vi "Trajectory Builder.vi"() -> ()   [LabVIEW 2025]
uses:
  Types/Limits.ctl
  Types/Overrides.ctl
  Types/Trajectory Data.ctl
  Types/Segment Type.ctl
  Types/Path Type.ctl
  Types/Drive Type.ctl
  Types/Angluar Limits.ctl
  Types/Command Editor Info.ctl
  Types/Single Cmd Info.ctl
  <vilib>/picture/picture.llb/imagedata.ctl
  <vilib>/Utility/miscctls.llb/LVPositionTypeDef.ctl
  Types/Full Command Info.ctl
  <vilib>/Utility/miscctls.llb/LVRowAndColumnTypeDef.ctl
  Types/Internal Path Stuff.ctl
  Types/Aquitaine File Data.ctl
  Types/Decision Tree.ctl
  Types/Sequencing Tree Node.ctl
  <vilib>/event_ctls.llb/lveventtype.ctl
  36995695-6583-4118-8a12-9ab3bbd2de6a.vi
  6a65ebb4-e776-4ba2-b94f-6ff829af6114.vi
  88e6daad-a1e9-44cd-90fd-d41817f6f65e.vi
  36995695-6583-4118-8a12-9ab3bbd2de6a.vi/4611cae3-c7be-41e2-9a5e-ea0ae78a7ced.vi
  6a65ebb4-e776-4ba2-b94f-6ff829af6114.vi/c0db33a9-eb6c-44d9-b982-8563e05d2734.vi
  6a65ebb4-e776-4ba2-b94f-6ff829af6114.vi/ae3535a8-0066-4e8d-a5de-b07ac05a7c65.vi
  6a65ebb4-e776-4ba2-b94f-6ff829af6114.vi/dda8e586-731b-4197-ad83-6a4d05585a0a.vi
  36995695-6583-4118-8a12-9ab3bbd2de6a.vi/4611cae3-c7be-41e2-9a5e-ea0ae78a7ced.vi/19e2e4cb-e3bb-4239-bd5f-680916605f5d.vi
  36995695-6583-4118-8a12-9ab3bbd2de6a.vi/4611cae3-c7be-41e2-9a5e-ea0ae78a7ced.vi/f72612c1-738a-48a1-9fcf-3db66cb27fb3.vi
  36995695-6583-4118-8a12-9ab3bbd2de6a.vi/4611cae3-c7be-41e2-9a5e-ea0ae78a7ced.vi/45406051-8994-464b-8b47-ac12a8cbadfa.vi
  36995695-6583-4118-8a12-9ab3bbd2de6a.vi/4611cae3-c7be-41e2-9a5e-ea0ae78a7ced.vi/dd886480-778c-48b1-8e4a-d6890e1a60dd.vi
  36995695-6583-4118-8a12-9ab3bbd2de6a.vi/4611cae3-c7be-41e2-9a5e-ea0ae78a7ced.vi/2e6e140f-e361-4312-a09e-e37273ac7fd1.vi
  36995695-6583-4118-8a12-9ab3bbd2de6a.vi/4611cae3-c7be-41e2-9a5e-ea0ae78a7ced.vi/3589548e-4c68-4568-af05-72ab28470577.vi
  36995695-6583-4118-8a12-9ab3bbd2de6a.vi/4611cae3-c7be-41e2-9a5e-ea0ae78a7ced.vi/cf64d4f5-91bd-4749-9577-68c6ded0155b.vi
  36995695-6583-4118-8a12-9ab3bbd2de6a.vi/4611cae3-c7be-41e2-9a5e-ea0ae78a7ced.vi/6f6fefe9-f25b-4595-b26f-75715299a794.vi
  36995695-6583-4118-8a12-9ab3bbd2de6a.vi/4611cae3-c7be-41e2-9a5e-ea0ae78a7ced.vi/c74ffb76-1048-4639-9a95-b6de96ba7014.vi
  Global Settings.vi
  <vilib>/Utility/cursorutil.llb/Set Cursor (Icon Pict).vi
  <vilib>/Analysis/1siggen.llb/Ramp Pattern by Delta.vi
  <vilib>/Comparison/Less/Less Functor/Less Functor.lvclass
  <vilib>/Analysis/NI_AALBase.lvlib
panel:
  in  "Open Aquitaine Editor":bool
  in  "Add Paths":bool
  in  "Aquitaine Add Selector":u16(ring) items=["Karthik.aqt"]
  in  "Delete AQT":bool
  in  "Push BORAQT":bool
  in  "Push AQT":bool
  in  "New AQT":bool
  in  "Zero Translational\n Velocity":bool
  in  "Delete":bool
  out "Picture":picture
  in  "New Page Selector":T1(radio)
  in  "Push":bool
  out "?":bool
  out "RS":bool=TRUE
  in  "Cache":T5
  in  "Zero Velocity":bool
  in  "Reverse Path":bool
  in  "Robot Backwards":bool
  out "Duration (s)":dbl format="%#.4g"
  out "Distance (ft)":dbl format="%#.1g"
  in  "Instructions":string="Directions:\nUse mouse to ...\n    move robot position (rectangle with arrow)\n    rotate robot (red arrow)\n    move waypoints (numbered circles)\nClick in open space to add a waypoint\nShift click to delete a waypoint\nHover over a waypoint and use arrow keys to nudge\n\nTime slider and Play button will run robot along path to test for collisions.\n\nNew creates a new path at default location\n\nAppend creates a path using current path's position and heading.\n\nTo add a command, move robot using Time slider and double click the Command in Palette.\n\nYou can modify command timing in the graph or Command Sequencer tree.\n\nEnable/disable a command by clicking on the enable column item.\n\nDelete a command by shift-clicking in the enable column.\n\nTo configure command parameters, Select the command name in the tree, Open Panel, enter parameters, and Inhale the parameters.\n\nYou may sometimes want to type values into WayPoints directly.\n\nOverrides allow you to set accel and V limits for any turn."
  out "Command Palette":picture
  in  "Directory":bool
  in  "Tab Control":T1(tab)
  in  "Vertical Reflection":bool
  in  "Angular Limits":T6={"Velocity (deg/s)"=6.0, "Accel (deg/s^2)"=360.0, "Jerk (deg/s^3)"=1000.0} {"Jerk (deg/s^3)" min=0.01 step=1.0; "Accel (deg/s^2)" min=0.01; "Velocity (deg/s)" min=0.01}
  in  "Path Type":T7
  in  "Overrides":T8 {"Angle Override" step=5.0; "Velocity Override" step=5.0; "Angular Override" step=5.0}
  in  "Horizontal Reflection":bool
  in  "Sample Period (s)":dbl=0.02 min=0.001 max=1.0 format="%#_6f"
  in  "Limits":T9={"Velocity (fps)"=6.0, "Accel (fps^2)"=15.0, "Jerk (fps^3)"=150.0, "StoopidFast (fps)"=6.0} {"StoopidFast (fps)" min=0.01; "Jerk (fps^3)" min=0.01 step=1.0; "Accel (fps^2)" min=0.01; "Velocity (fps)" min=0.01}
  in  "Conditions":T10 {"vFinal (fps)" min=0.0; "vInitial (fps)" min=0.0}
  in  "Drive Type":T11=enum."Holonomic"
  in  "Turn Rate (Bezier)":dbl=5.0 format="%#_13g"
  in  "Origin Reflection":bool
  in  "Current Limit":dbl=50.0 min=0.01
  in  "WayPoints":cluster{"x":dbl, "y":dbl, "th":dbl}[](array[cluster])
  in  "Turn Angle Limit (deg)":dbl=90.0
  in  "Allow Angles > 90":bool=TRUE
  in  "Stoopid Overlap %":dbl min=0.0
  in  "Unjank":bool
  in  "Turn Deceleration":bool=TRUE
  in  "Turn Acceleration":bool=TRUE
  out "Trajectory Data":T12
  in  "Open Command":bool
  in  "Inhale":bool
  in  "Command Sequence":string(tree)
  in  "Projects":u16(ring) items=["Robot Code Template.lvproj"]
  in  "Refresh":bool
  in  "Snap to foot":bool
  in  "Angle Limiter":enum16{"90", "45", "15", "1"}(ring)=enum."15"
  in  "Snap robot to baseline":bool
  in  "Background":u16(ring) items=["Rebuilt", "Reefscape"]
  in  "Robot Color":u32(colorbox)=14421504
  out "Field Size (ft)":cluster{"width":dbl, "height":dbl}={"width"=26.4166, "height"=57.5729} {"width" format="%#.2g"; "height" format="%#.2g"}
  in  "Robot Size (in)":cluster{"width":dbl, "height":dbl}={"width"=24.0, "height"=30.0}
  in  "Hide Path":bool
  in  "Draw?":bool
  in  "Draw Delete":bool
  in  "Draw Menu":i32[](listbox)
  in  "Time (s)":dbl(slide) scale=0.0..1.6400000000000001 scale format="%#.1g"
  in  "Play":bool
  out "fps":dbl[](graph)
  in  "Append":bool
  in  "Filename":string
  in  "Save":bool
  in  "New":bool
  in  "File Manager":enum32{"Bordeaux Files", "Aquitaine Files"}(tab)
  in  "Open":i32[](listbox)
  in  "Tree":string[](tree)
  # "Command Palette"
  # "StupidFast makes each linear segment into a\nvelocity ramp to max speed (for clothoid paths only)"
  # "Nicotine"
  # "A"
  # "V"
  # "O"
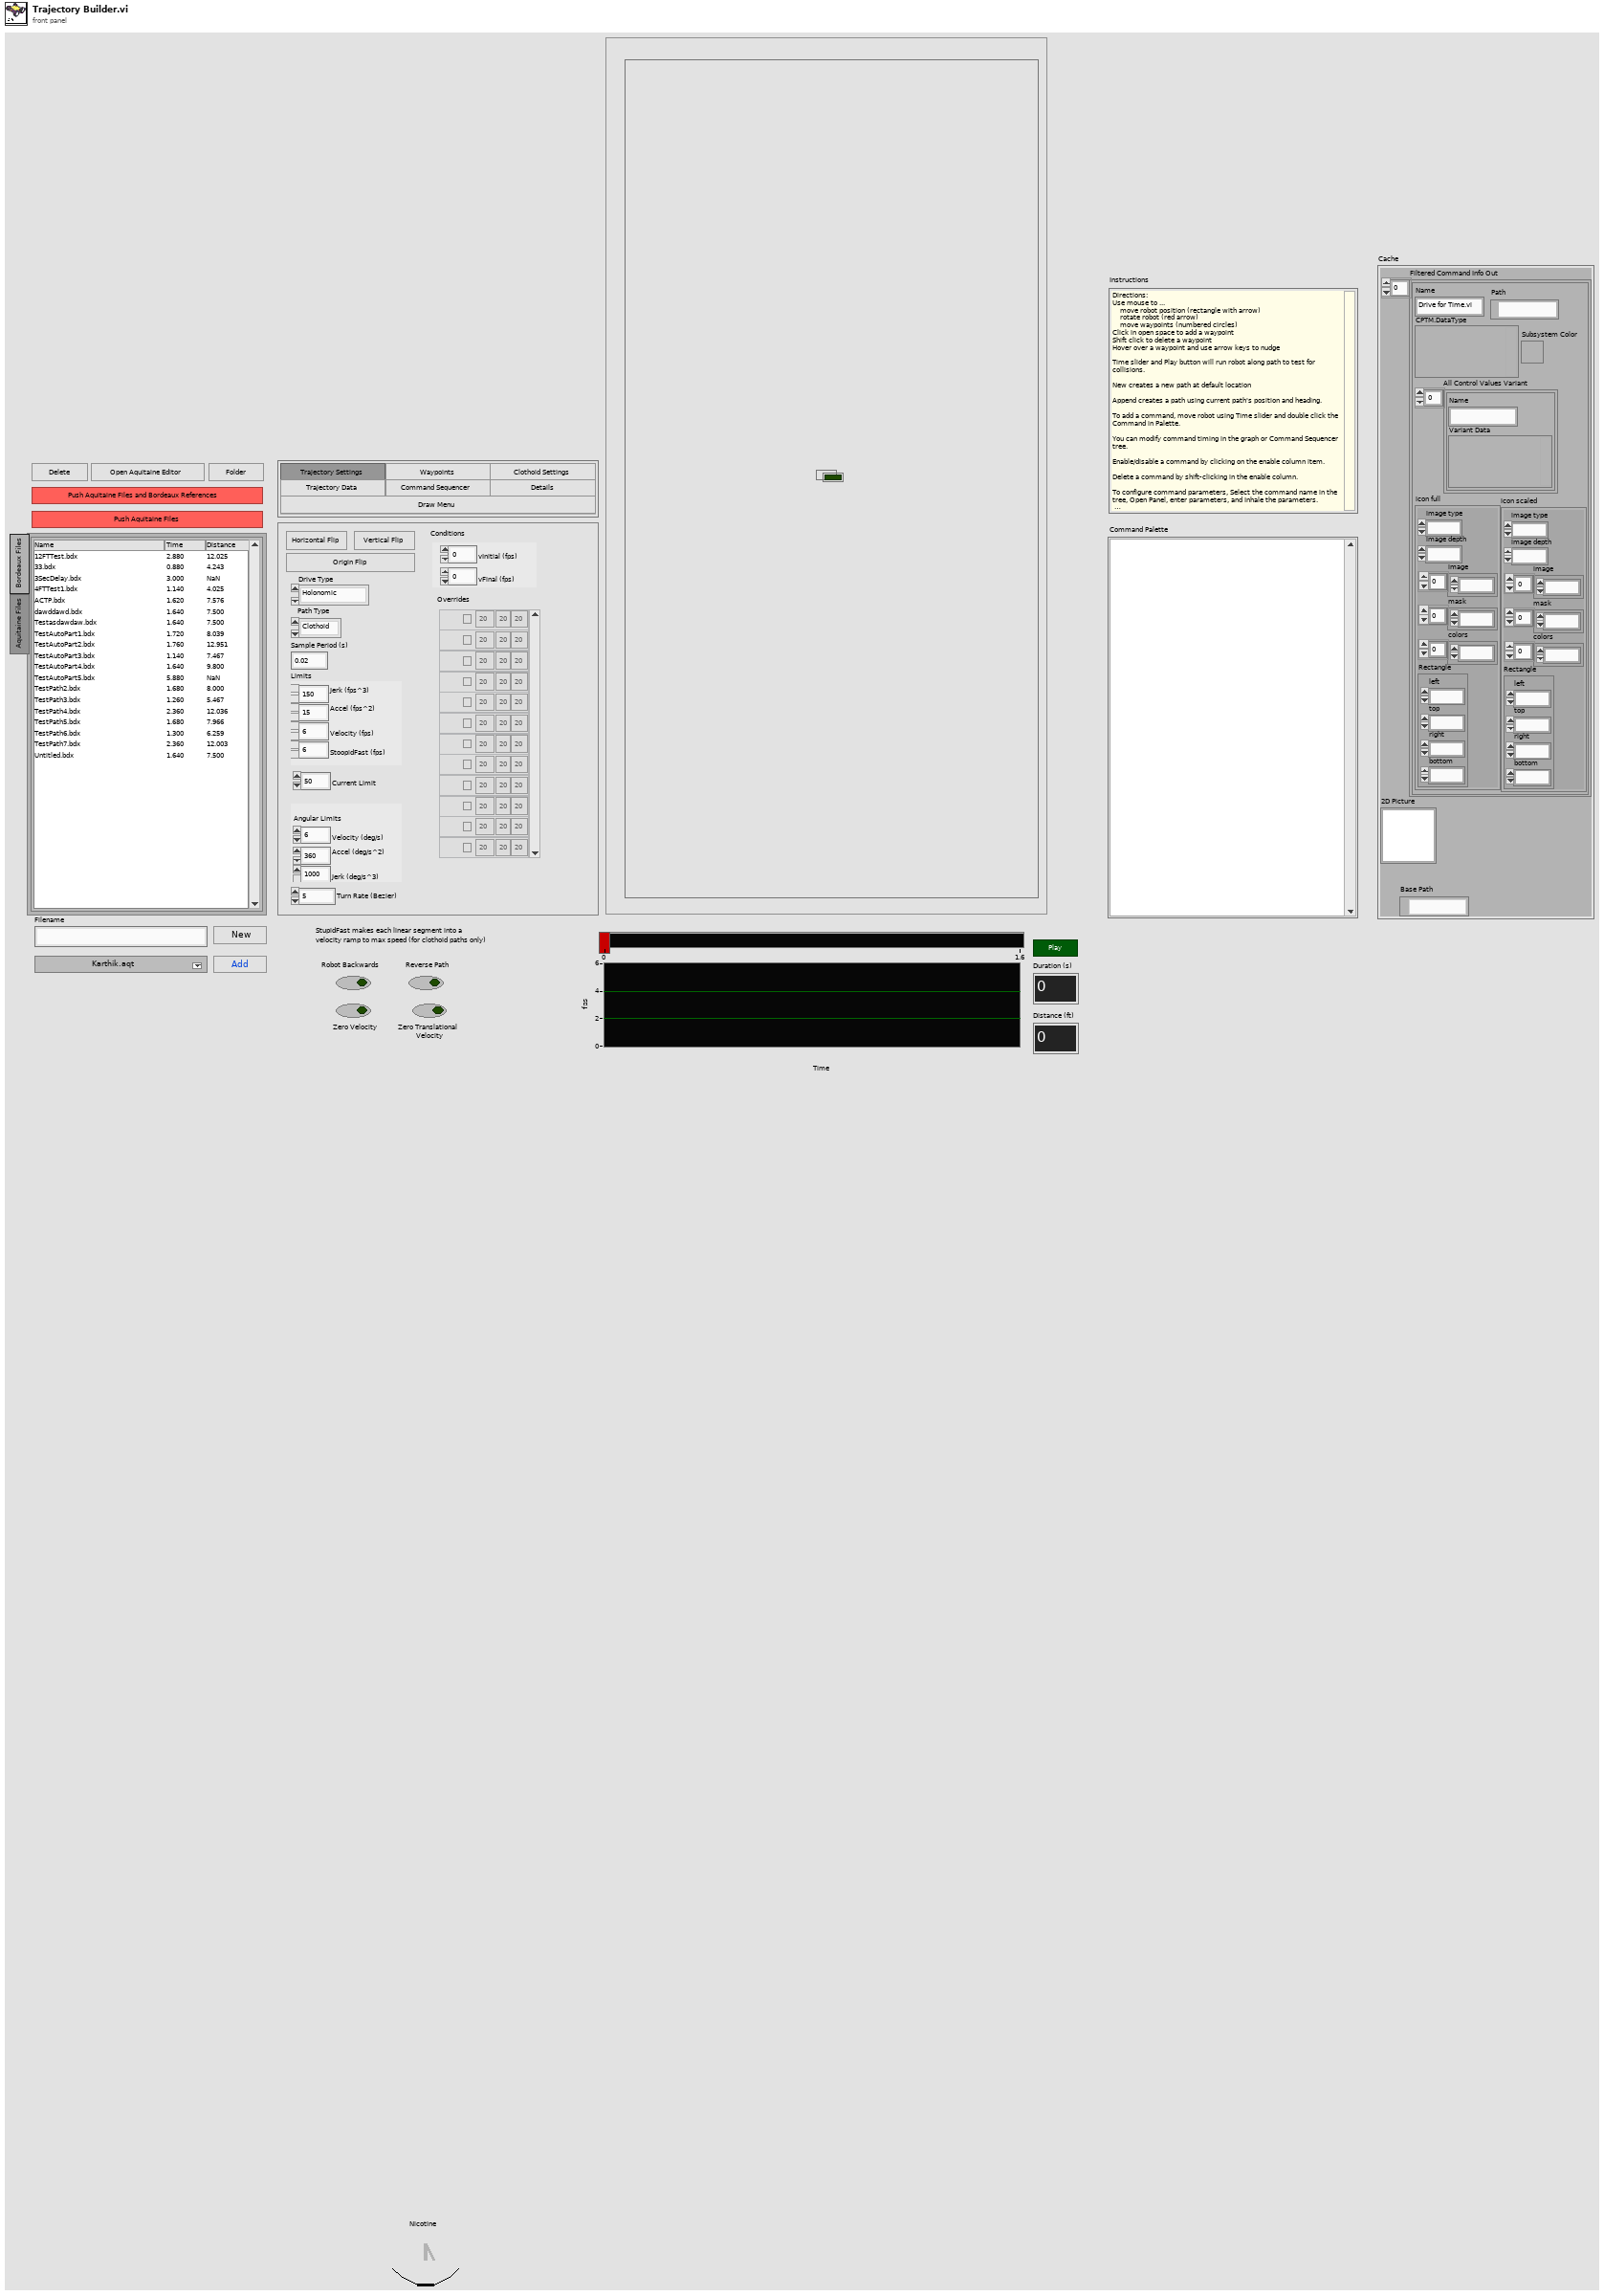
[diagram p1: front panel]
types:
  T1 = enum32{"Trajectory Settings", "Waypoints", "Clothoid Settings", "Trajectory Data", "Command Sequencer", "Details", "Draw Menu"}
  T2 = typedef "Command Editor Info.ctl" = T3[]
  T3 = typedef "Single Cmd Info.ctl" = cluster{"Name":string, "CPTM.DataType":variant, "All Control Values Variant":cluster{"Name":string, "Variant Data":variant}[], "icon full":T4, "icon scaled":T4, "Path":path, "Subsystem Color":u32}
  T4 = typedef "imagedata.ctl" = cluster{"image type":i32, "image depth":i32, "image":u8[], "mask":u8[], "colors":u32[], "Rectangle":cluster{"left":i16, "top":i16, "right":i16, "bottom":i16}}
  T5 = cluster{"Filtered Command Info Out":T2, "2D Picture":picture, "Base Path":path}
  T6 = typedef "Angluar Limits.ctl" = cluster{"Velocity (deg/s)":dbl, "Accel (deg/s^2)":dbl, "Jerk (deg/s^3)":dbl}
  T7 = typedef "Path Type.ctl" = enum16{"Clothoid", "Bezier"}
  T8 = typedef "Overrides.ctl" = cluster{"Count":string, "Angular Override":dbl, "Enabled?":bool, "Velocity Override":dbl, "Angle Override":dbl}[]
  T9 = typedef "Limits.ctl" = cluster{"Velocity (fps)":dbl, "Accel (fps^2)":dbl, "Jerk (fps^3)":dbl, "StoopidFast (fps)":dbl}
  T10 = cluster{"vInitial (fps)":dbl, "vFinal (fps)":dbl}
  T11 = typedef "Drive Type.ctl" = enum16{"Nonholonomic", "Holonomic"}
  T12 = typedef "Trajectory Data.ctl" = cluster{"Segment Name":string, "Type":T13, "Traj Pos Points":cluster{"x":dbl, "y":dbl, "th":dbl}[], "Traj Vel Points":cluster{"V":dbl, "Omega":dbl, "V vector":cluster{"y":dbl, "x":dbl}}[], "Accel Index":i32, "Decel Index":i32}[]
  T13 = typedef "Segment Type.ctl" = enum16{"Accel Straight", "Const Straight", "Blend", "Circle", "Bezier"}
  T14 = enum32{"Trajectory Settings", "Waypoints", "Clothoid Settings", "Trajectory Data", "Command Sequencer", "Details"}
  T15 = cluster{"Sample Period (s)":dbl, "Limits":T9, "Conditions":cluster{"vInitial (fps)":dbl, "vFinal (fps)":dbl}, "Overrides":T8, "Angular Limits":T6}
  T16 = typedef "LVRowAndColumnTypeDef.ctl" = cluster{"Row":i32, "Column":i32}
  T17 = typedef "Full Command Info.ctl" = cluster{"Start Time (s)":dbl, "End Time (s)":dbl, T3, "Visible":bool, "Enabled?":bool}[]
  T18 = typedef "LVPositionTypeDef.ctl" = cluster{"Left":i32, "Top":i32}
  T19 = cluster{"Index":i32, "Pt Test Results":enum16{"Miss", "Rect Hit", "Arrow Hit"}}
  T20 = cluster{"Drag Object":cluster{"Index":i32, "x":dbl, "y":dbl}, "Hover Object":cluster{"Index":i32, "Pt Test Results":enum16{"Miss", "Rect Hit", "Arrow Hit"}}, "Filename":string}
  T21 = cluster{"Trajectory Data":T12, "Points":cluster{"x":dbl, "y":dbl, "th":dbl}[], "output cluster":cluster{"Sample Period (s)":dbl, "Limits":T9, "Conditions":cluster{"vInitial (fps)":dbl, "vFinal (fps)":dbl}, "Overrides":T8, "Angular Limits":T6}, T17}
  T22 = typedef "Internal Path Stuff.ctl" = cluster{"Trajectory Data":T12, "Updated Waypoints":cluster{"x":dbl, "y":dbl, "th":dbl}[], cluster{"Sample Period (s)":dbl, "Limits":T9, "Conditions":cluster{"vInitial (fps)":dbl, "vFinal (fps)":dbl}, "Overrides":T8, "Angular Limits":T6}, "Commands out":T17}
  T23 = cluster{"Sample Period (s)":dbl, cluster{"Velocity (fps)":dbl, "Accel (fps^2)":dbl, "Jerk (fps^3)":dbl, "StoopidFast (fps)":dbl}, "Conditions":cluster{"vInitial (fps)":dbl, "vFinal (fps)":dbl}, "Overrides":T8, "Angular Limits":T6}
  T24 = typedef "Aquitaine File Data.ctl" = cluster{"Path References":path[], "Decision Tree":T25}
  T25 = typedef "Decision Tree.ctl" = cluster{"Tree":T26[], "Node To Index Lookup Map":map{i16, i16[]}}
  T26 = typedef "Sequencing Tree Node.ctl" = cluster{"Node Type":enum16{"Path", "Command", "Leaf"}, "ID":i16, "Path Data":cluster{"Path Name":string, "Outcome Name":string}, "Single Cmd Info":T3, "Child ID":i32[], "Parent ID":i32, "Drawing Info":cluster{"X":i32, "Y":i32, "Width":i32, "Height":i32}}
  T27 = typedef "lveventtype.ctl" = enum32{"Null", "Timeout", "Annotation Menu Selection", "Annotation Menu Selection?", "App Instance Close", "App Instance Close?", "Autoscale Range Change", "Bookmark Info Change", "Cell Edit", "Cell Edit?", "Cursor Grab", "Cursor Grab?", "Cursor Menu Selection", "Cursor Menu Selection?", "Cursor Move", "Cursor Release", "Data Change", "Direction Change", "Display State Change", "Drag Ended", "Drag Enter", "Drag Leave", "Drag Over", "Drag Source Update", "Drag Starting", "Drag Starting?", "Drop", "Exec State Change", "Key Down", "Key Down?", "Key Repeat", "Key Repeat?", "Key Up", "Listbox Double Click", "Menu Activation?", "Menu Selection (App)", "Menu Selection? (App)", "Menu Selection (User)", "Mouse Down", "Mouse Down?", "Mouse Enter", "Mouse Leave", "Mouse Move", "Mouse Up", "Mouse Wheel", "NI Security User Change (App)", "Pane Size", "Panel Close", "Panel Close?", "Panel Resize", "Plot Attribute Change", "Scale Range Change", "Shortcut Menu Activation?", "Shortcut Menu Selection (App)", "Shortcut Menu Selection? (App)", "Shortcut Menu Selection (User)", "Tree Double Click", "Tree Drag", "Tree Drag?", "Tree Drop", "Tree Drop?", "Tree Item Close", "Tree Item Close?", "Tree Item Open", "Tree Item Open?", "User Event", "Value Change"}
  T28 = enum32{"Invalid", "Standard", "Closed", "Hidden", "Minimized", "Maximized"}
  T29 = cluster{"width":dbl, "height":dbl, "width":dbl, "height":dbl}
  T30 = cluster{"status":bool, "code":bool, "source":bool}
  T31 = cluster{"Robot Backwards":bool, "Reverse Path":bool}
  T32 = cluster{cluster{"Robot Backwards":bool, "Reverse Path":bool}, "Trajectory Data":T12, "Commands out":T17, cluster{"Sample Period (s)":dbl, "Limits":T9, "Conditions":cluster{"vInitial (fps)":dbl, "vFinal (fps)":dbl}, "Overrides":T8, "Angular Limits":T6}, "Updated Waypoints":cluster{"x":dbl, "y":dbl, "th":dbl}[], cluster{"Time (s)":dbl, "Distance (ft)":dbl}, "Zero Velocity":bool, cluster{"Drive Type":T11, "Path Type":T7}, "Current Limit":dbl, "Zero Translational\n Velocity":bool}
  T33 = cluster{"Trajectory Data":T12, "Updated Waypoints":cluster{"x":dbl, "y":dbl, "th":dbl}[], cluster{"Sample Period (s)":dbl, "Limits":T9, "Conditions":cluster{"vInitial (fps)":dbl, "vFinal (fps)":dbl}, "Overrides":T8, "Angular Limits":T6}, "Commands out":T17}
  T34 = cluster{"Path References":path[], "Decision Tree":T25}
  T35 = cluster{"Velocity (fps)":dbl, "Accel (fps^2)":dbl, "Jerk (fps^3)":dbl, "StoopidFast (fps)":dbl}
  T36 = cluster{"Trajectory Data":T12, "Points out":cluster{"x":dbl, "y":dbl, "th":dbl}[], "Fields":cluster{"Sample Period (s)":dbl, cluster{"Velocity (fps)":dbl, "Accel (fps^2)":dbl, "Jerk (fps^3)":dbl, "StoopidFast (fps)":dbl}, "Conditions":cluster{"vInitial (fps)":dbl, "vFinal (fps)":dbl}, "Overrides":T8, "Angular Limits":T6}, "Commands out":T17}
  T37 = typedef "LVPoint32TypeDef.ctl" = cluster{"Horizontal":i32, "Vertical":i32}
  T38 = cluster{"Shift":bool, "Ctrl":bool, "Alt":bool, "Cmd":bool, "Opt":bool}
  T39 = typedef "LVBoundsTypeDef.ctl" = cluster{"Width":u32, "Height":u32}
  T40 = cluster{"Snap robot to baseline":bool, "Snap to foot":bool, "Angle Limiter":enum16{"90", "45", "15", "1"}}
  T41 = cluster{i32, "Pt Test Results":enum16{"Miss", "Rect Hit", "Arrow Hit"}}
  T42 = typedef "eventvkey.ctl" = enum16{"ASCII", "Enter", "Return", "Shift", "Ctrl", "Alt", "Cmd", "Opt", "Caps", "NumLock", "Clear", "Break", "Up", "Down", "Left", "Right", "Insert", "Delete", "Home", "End", "PageUp", "PageDown", "Escape", "Help", "Pause", "ScrollLock", "F1", "F2", "F3", "F4", "F5", "F6", "F7", "F8", "F9", "F10", "F11", "F12", "F13", "F14", "F15", "F16", "F17", "F18", "F19", "F20", "F21", "F22", "F23", "F24", "Play", "VolumeUp", "VolumeDown", "Mute", "Two Byte Char"}
  T43 = cluster{"Name":string, "CPTM.DataType":variant, "Get All Control Values Variant":cluster{"Name":string, "Variant Data":variant}[], "Color 256":T4, "Subsystem Color":u32}[]
  T44 = cluster{"Filtered Command Info Out":T2, "2D Picture":picture, "stripped path":path}
  T45 = cluster{"Start Time (s)":dbl, "End Time (s)":dbl, T3, "Visible":bool, "Enabled?":bool}
  T46 = cluster{void, void, cluster{"Label.Text":string, "Value":variant}[], void, void, void, void}
  T47 = cluster{"Time (s)":dbl, "Time (s)":dbl, T3, bool, bool}
  T48 = cluster{"Targets":refnum<vi>[], "Paths":path[], "Projects":u16}
  T49 = cluster{"Name":string, "Color":u32, "Style":i32, "Point Style":i32, "Name Visible":bool, "Allow Drag":bool, "Annotation Mode":i32, "Plot":i32, "Index":i32, "Position":cluster{"X":dbl, "Y":dbl}, "X Scale":i32, "Y Scale":u32, "Show Arrow":bool, "Lock Name":bool, "Plot Area":i32, "Label Offset":cluster{"X":dbl, "Y":dbl}}[]
  T50 = cluster{"Horizontal":dbl, "Vertical":dbl, "th":dbl}
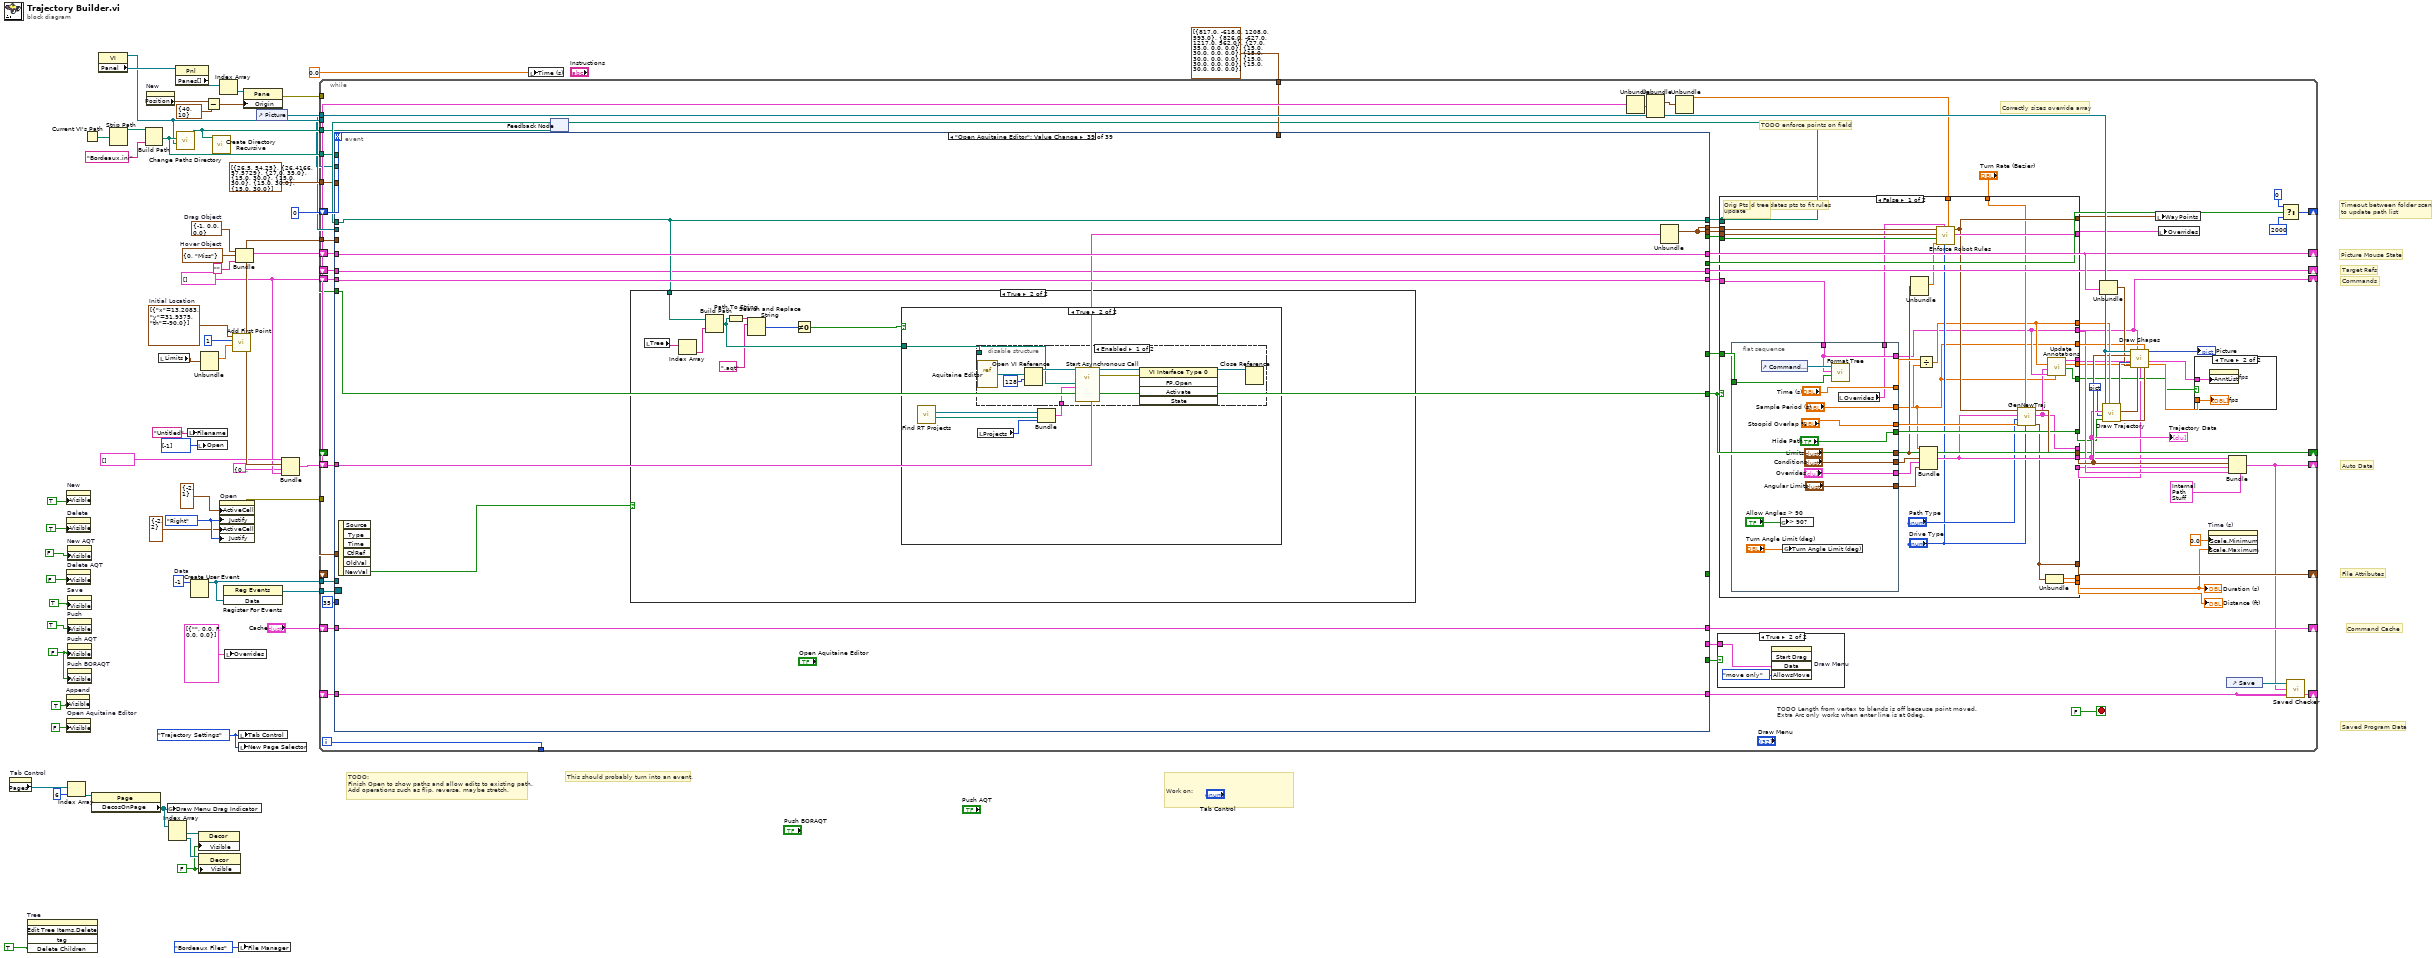
[diagram p0: block diagram]
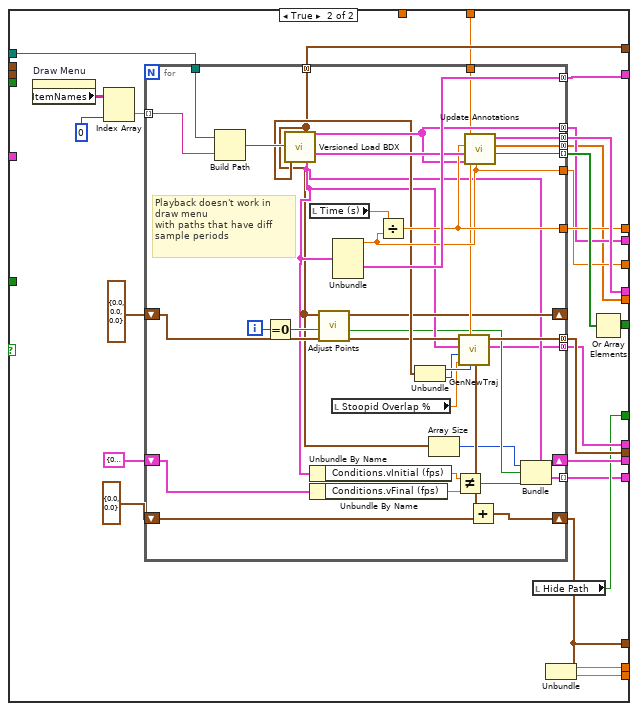
[diagram p2: hidden frame]
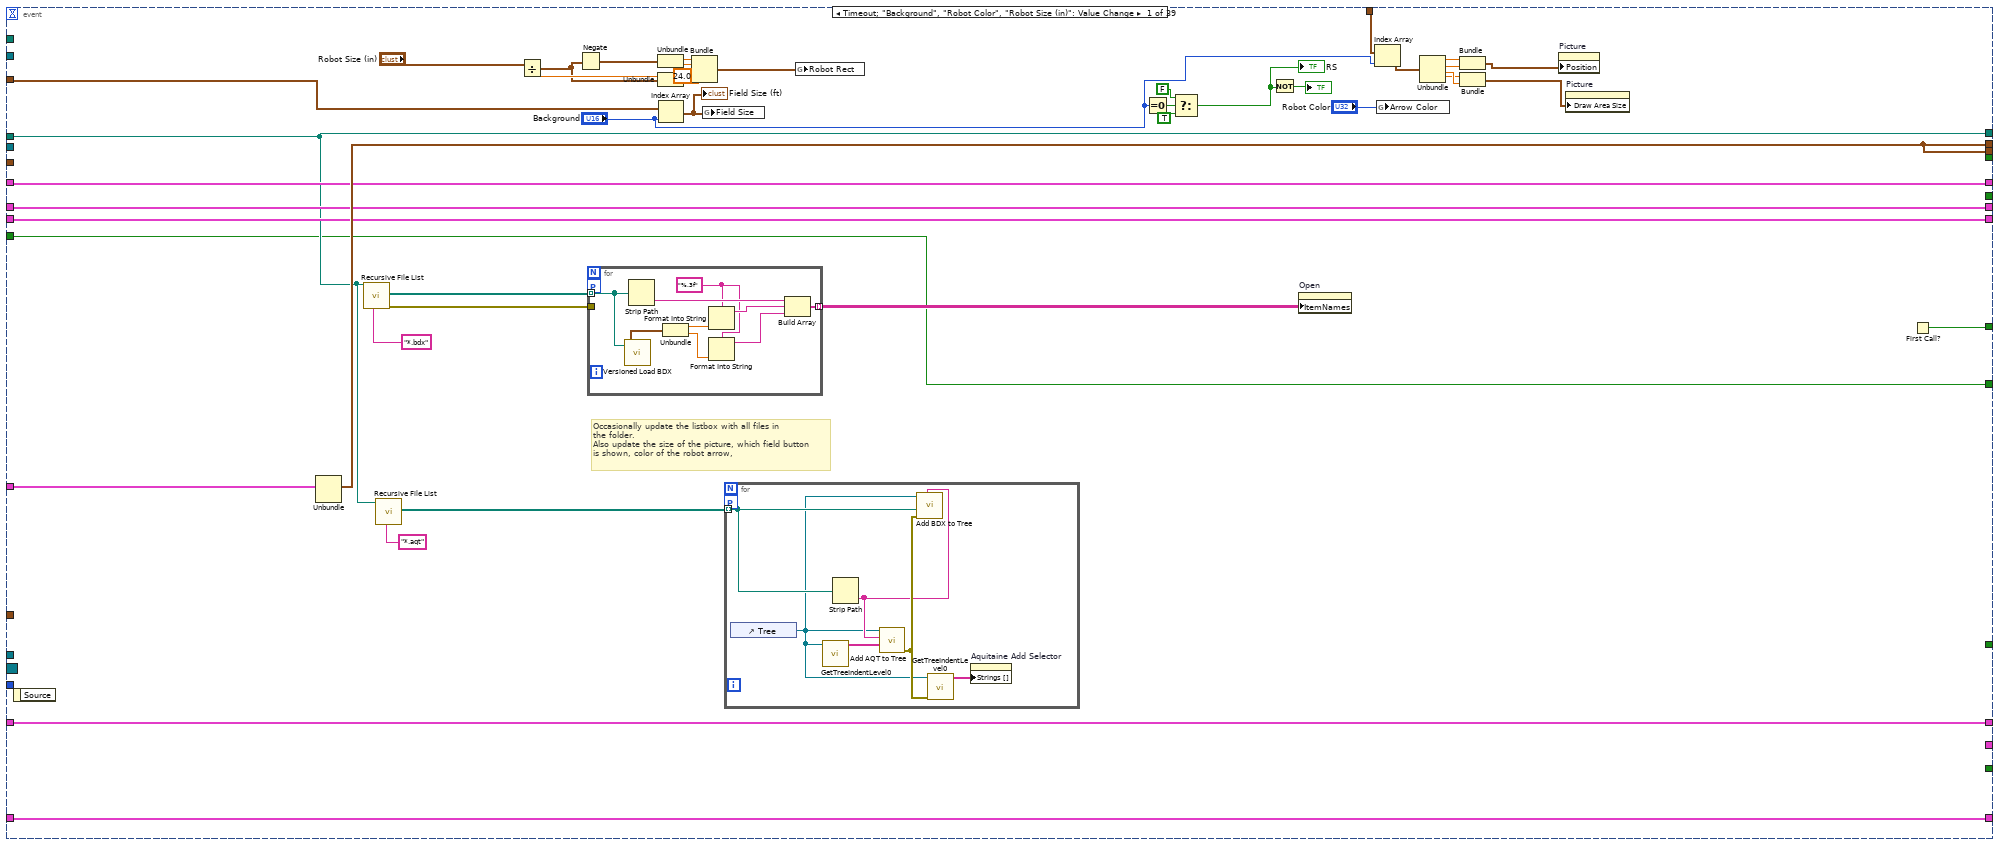
[diagram p4: hidden frame]
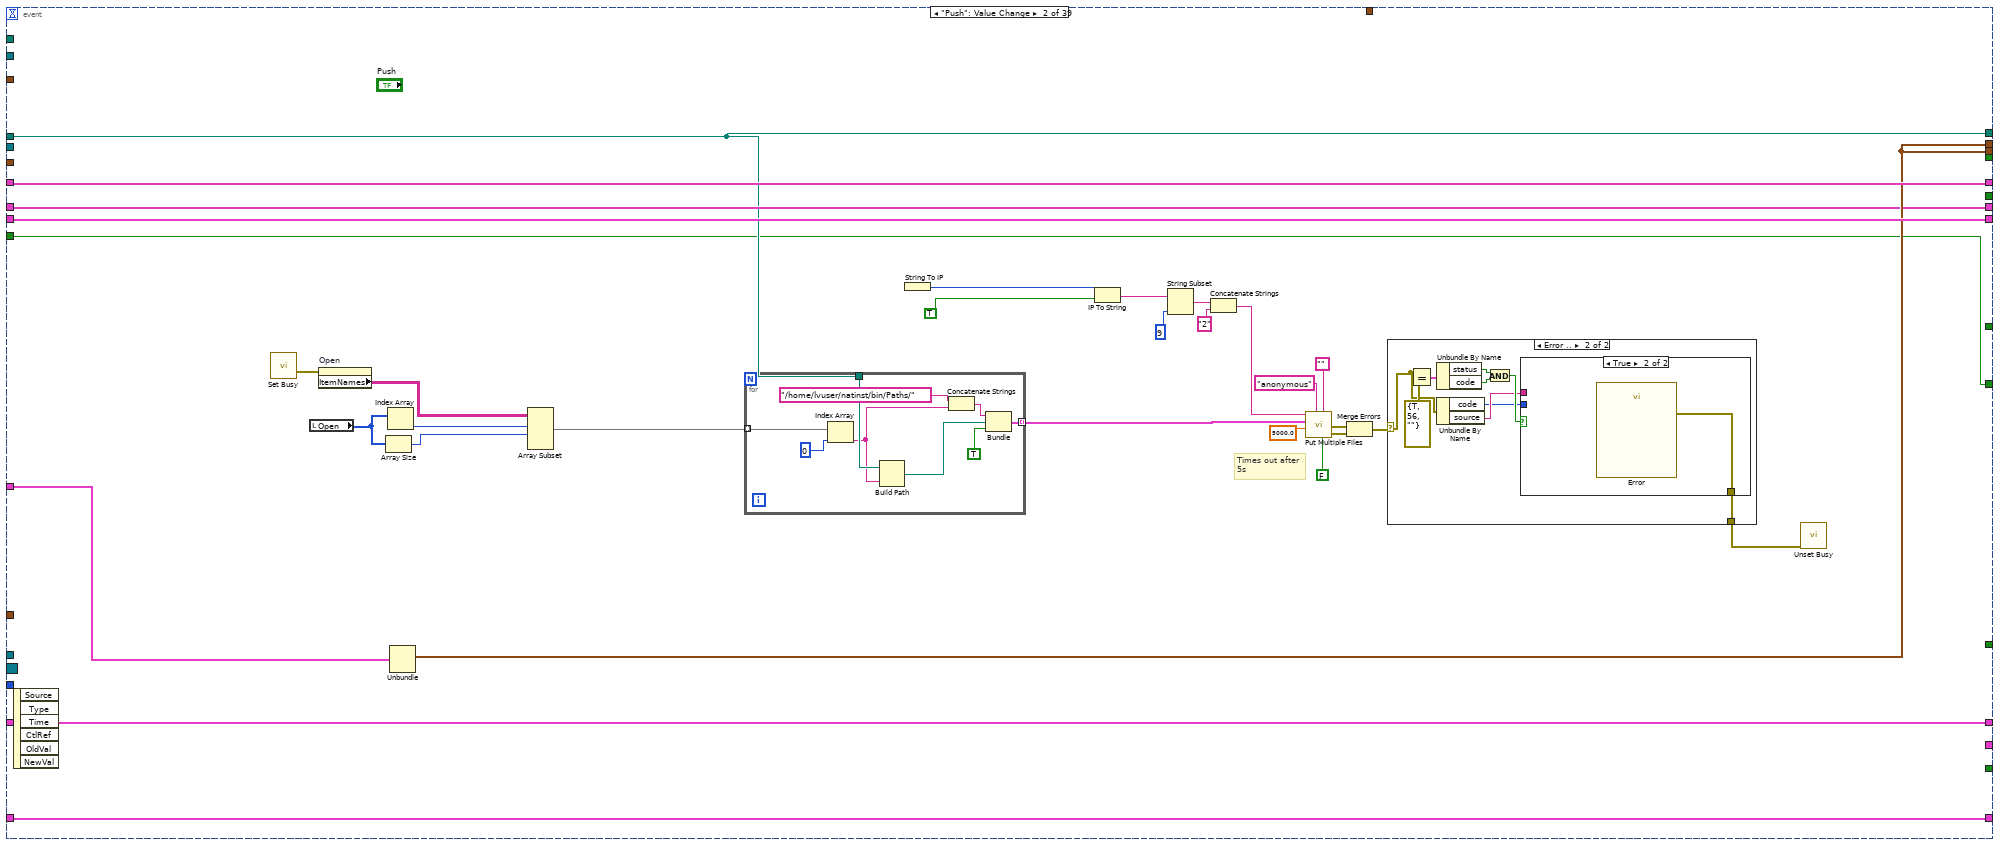
[diagram p5: hidden frame]
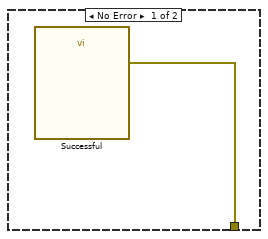
[diagram p6: hidden frame]
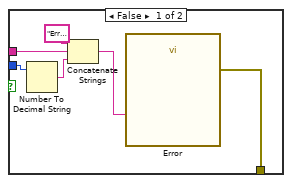
[diagram p7: hidden frame]
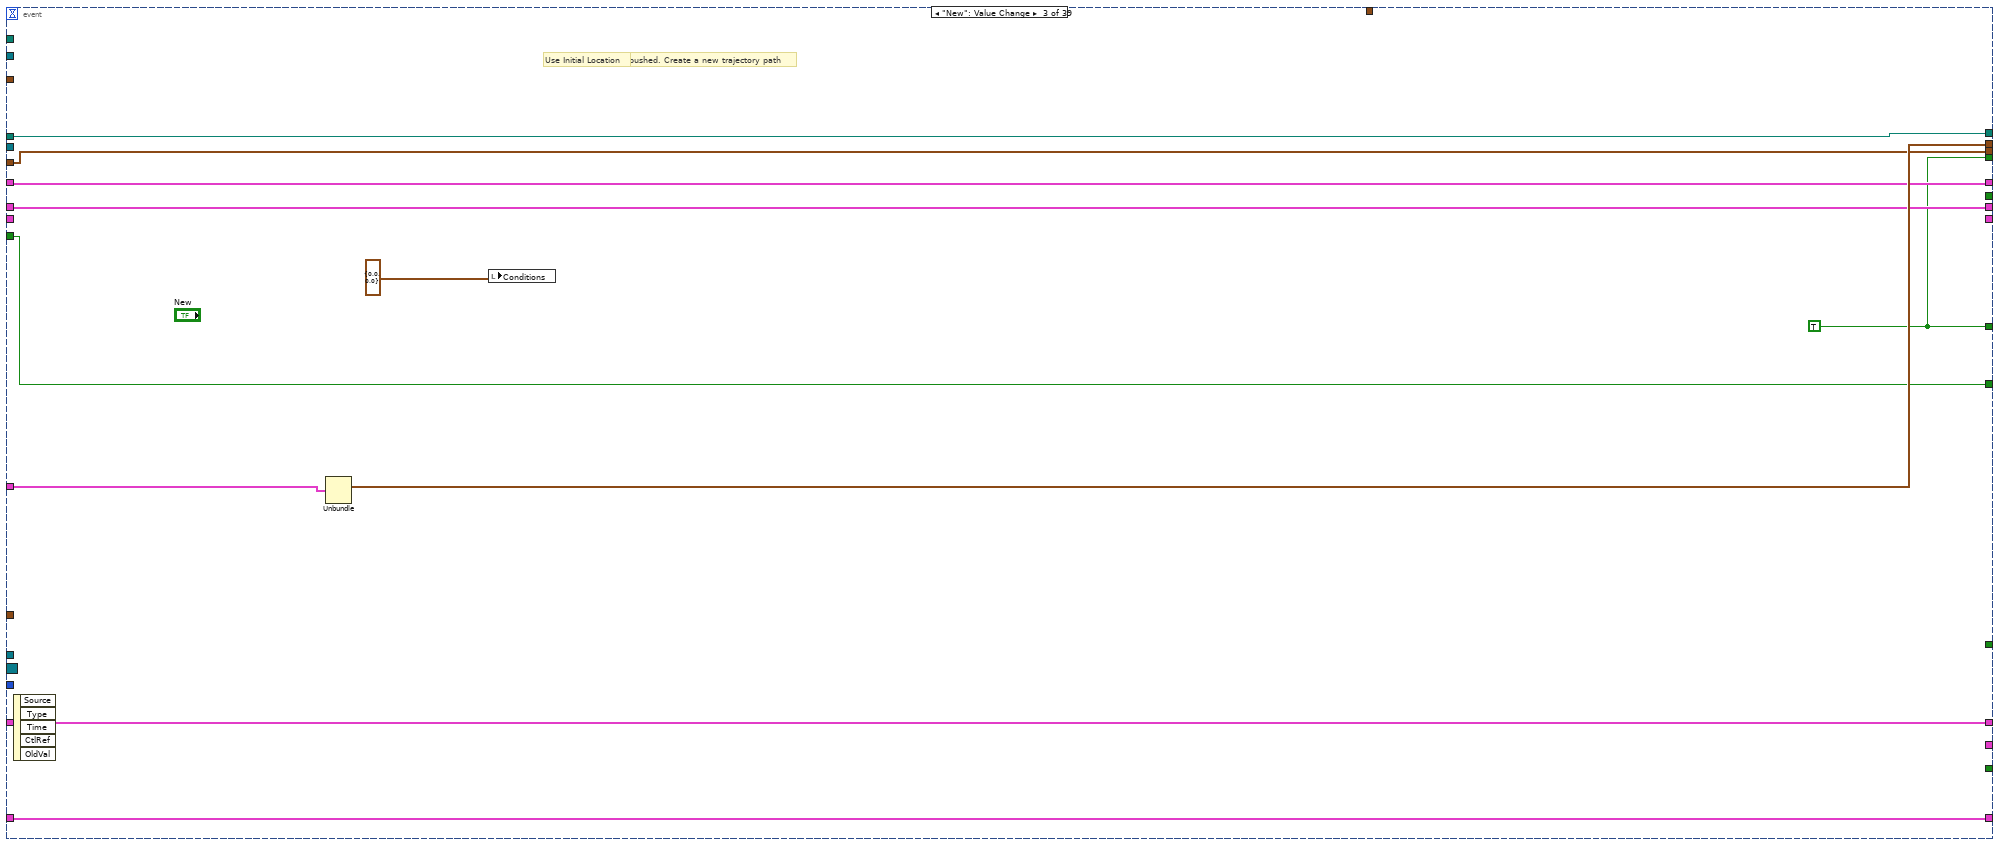
[diagram p8: hidden frame]
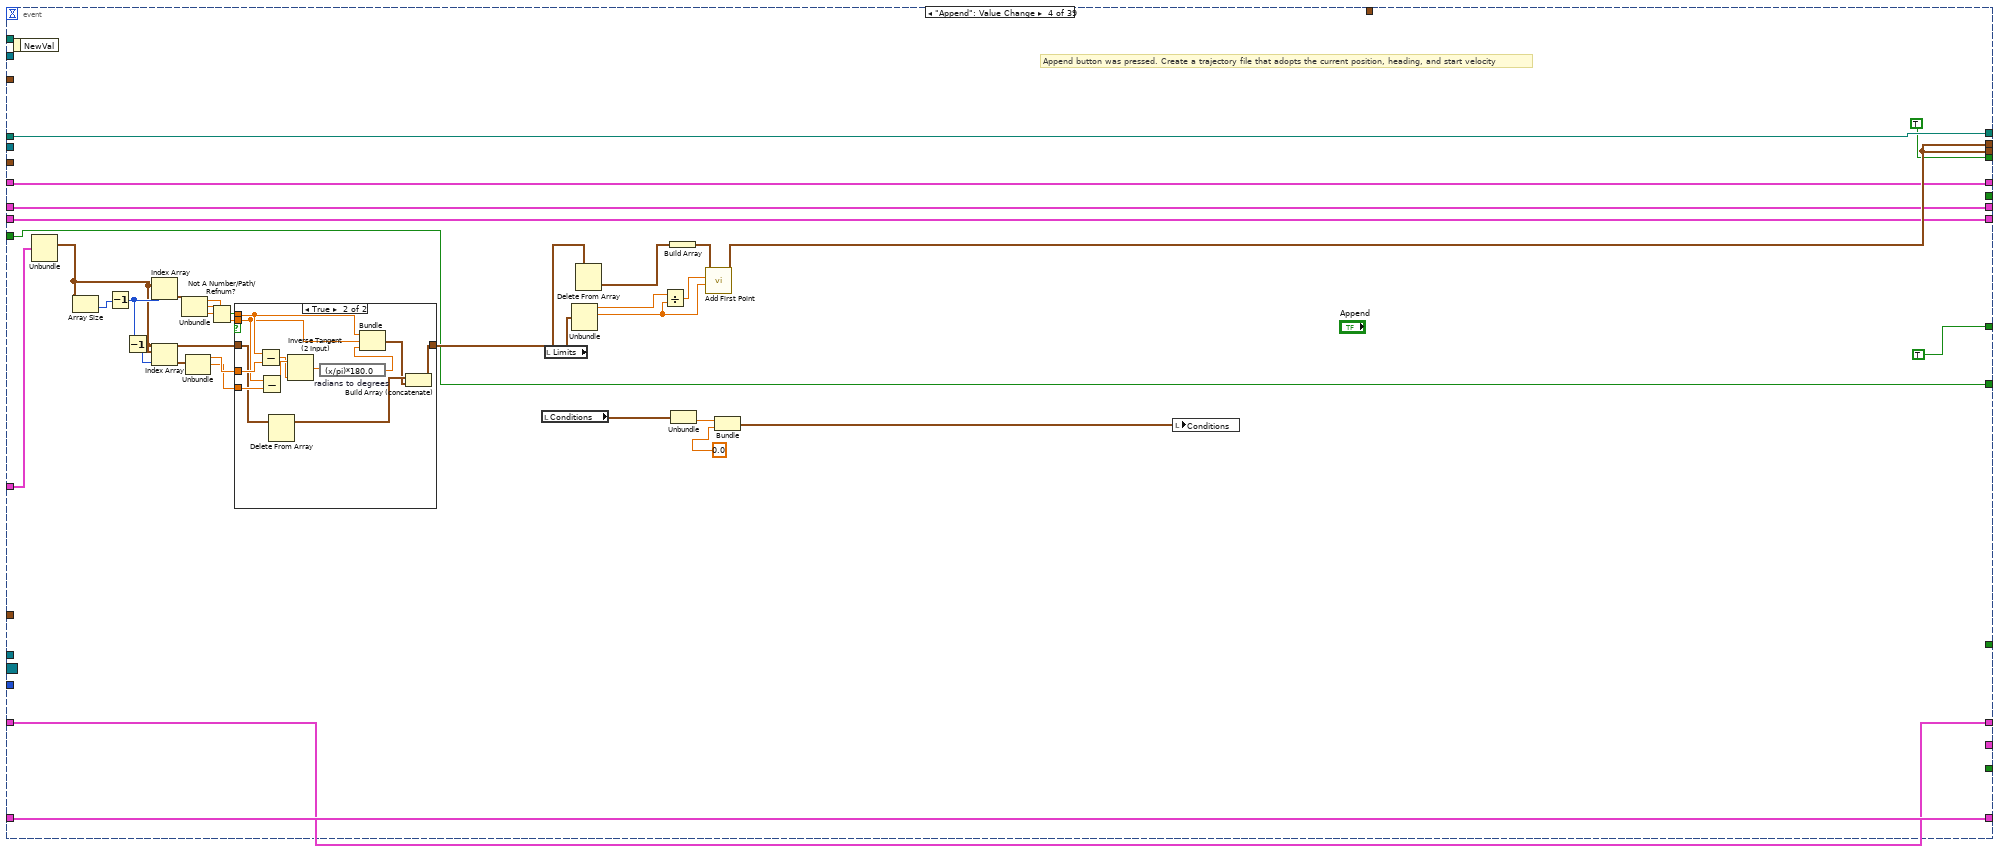
[diagram p9: hidden frame]
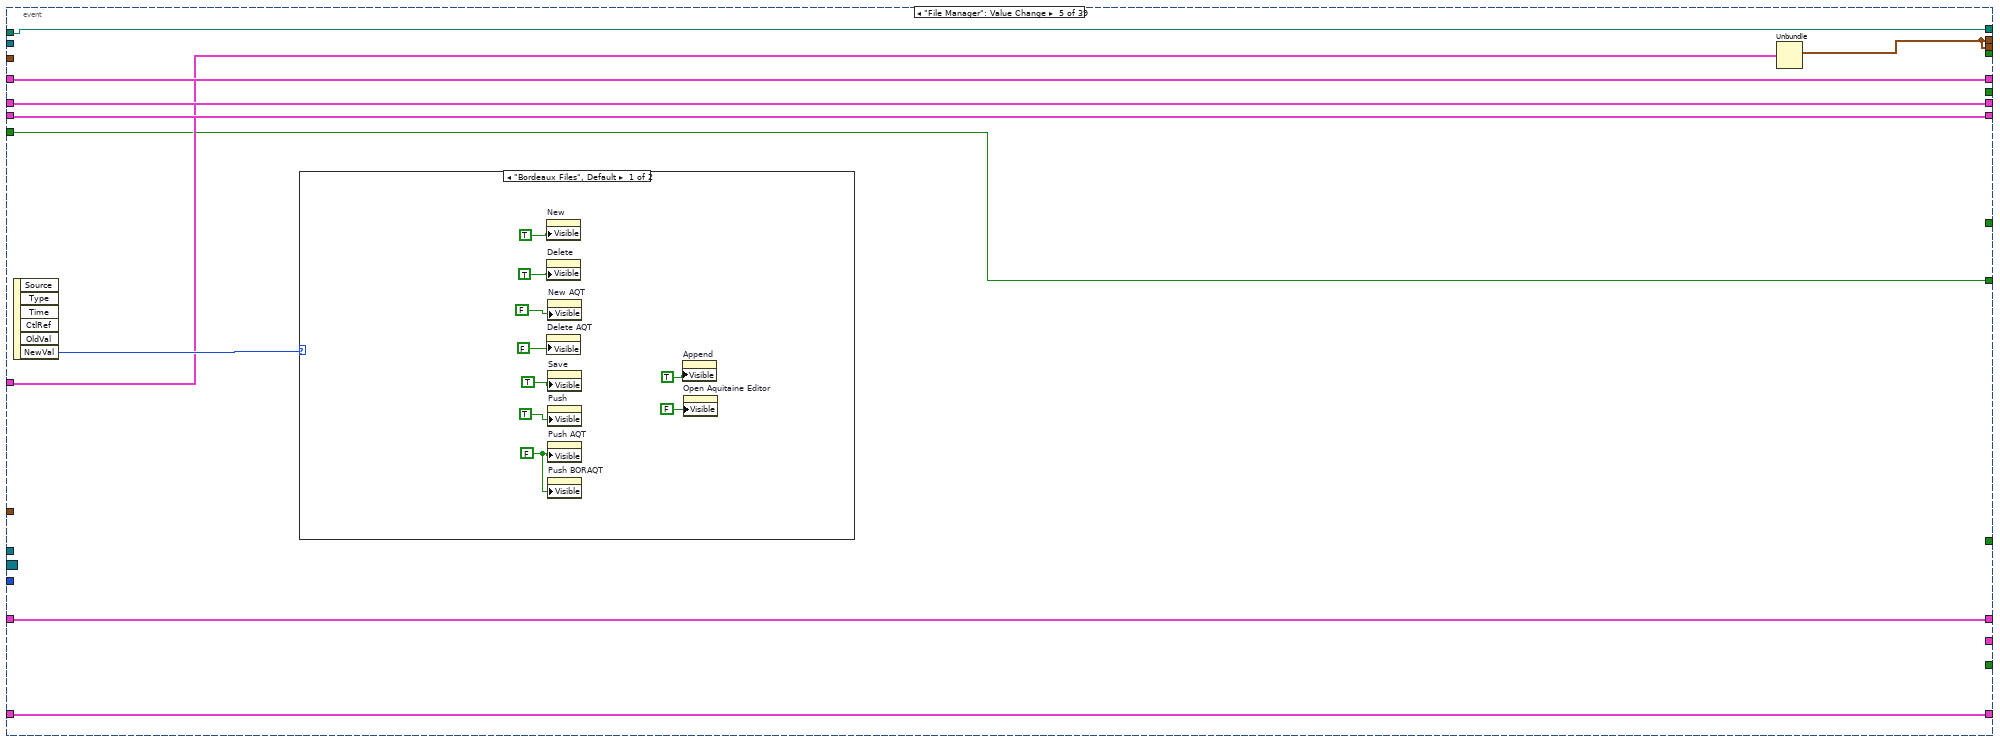
[diagram p11: hidden frame]
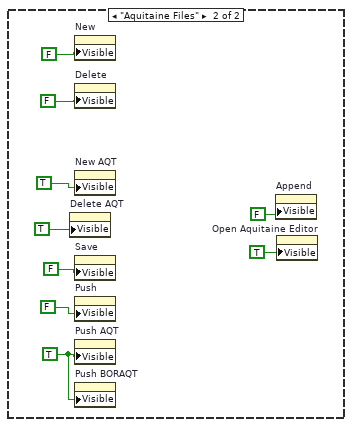
[diagram p12: hidden frame]
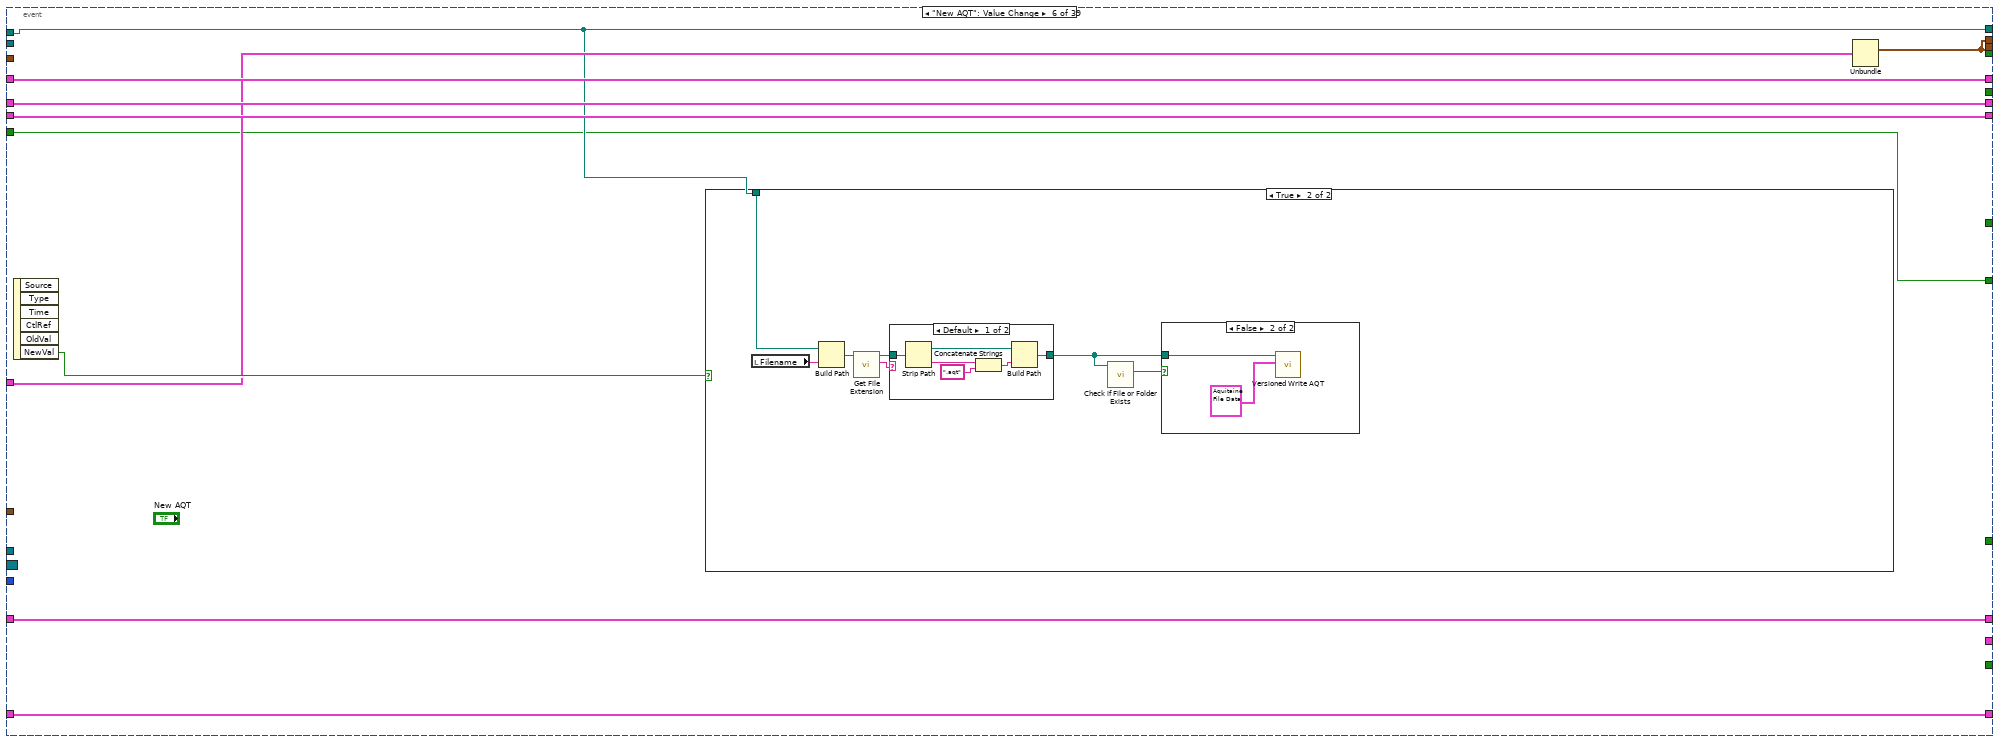
[diagram p13: hidden frame]
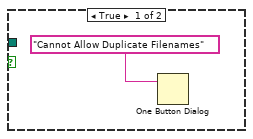
[diagram p15: hidden frame]
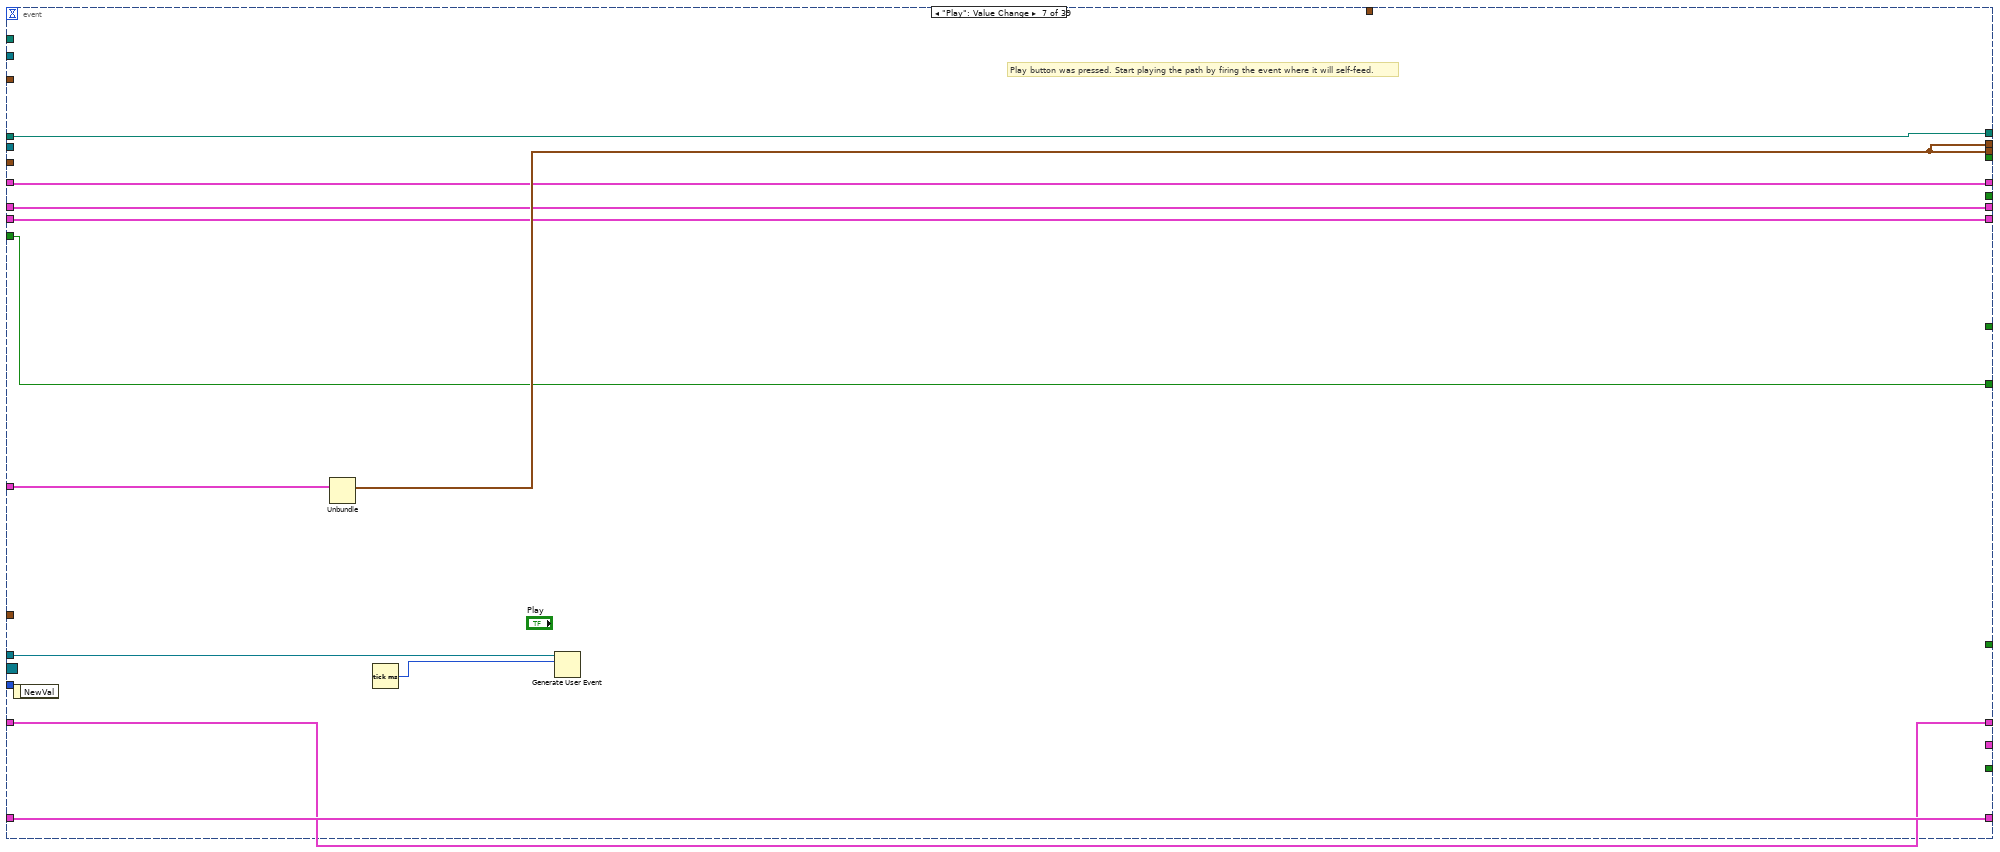
[diagram p17: hidden frame]
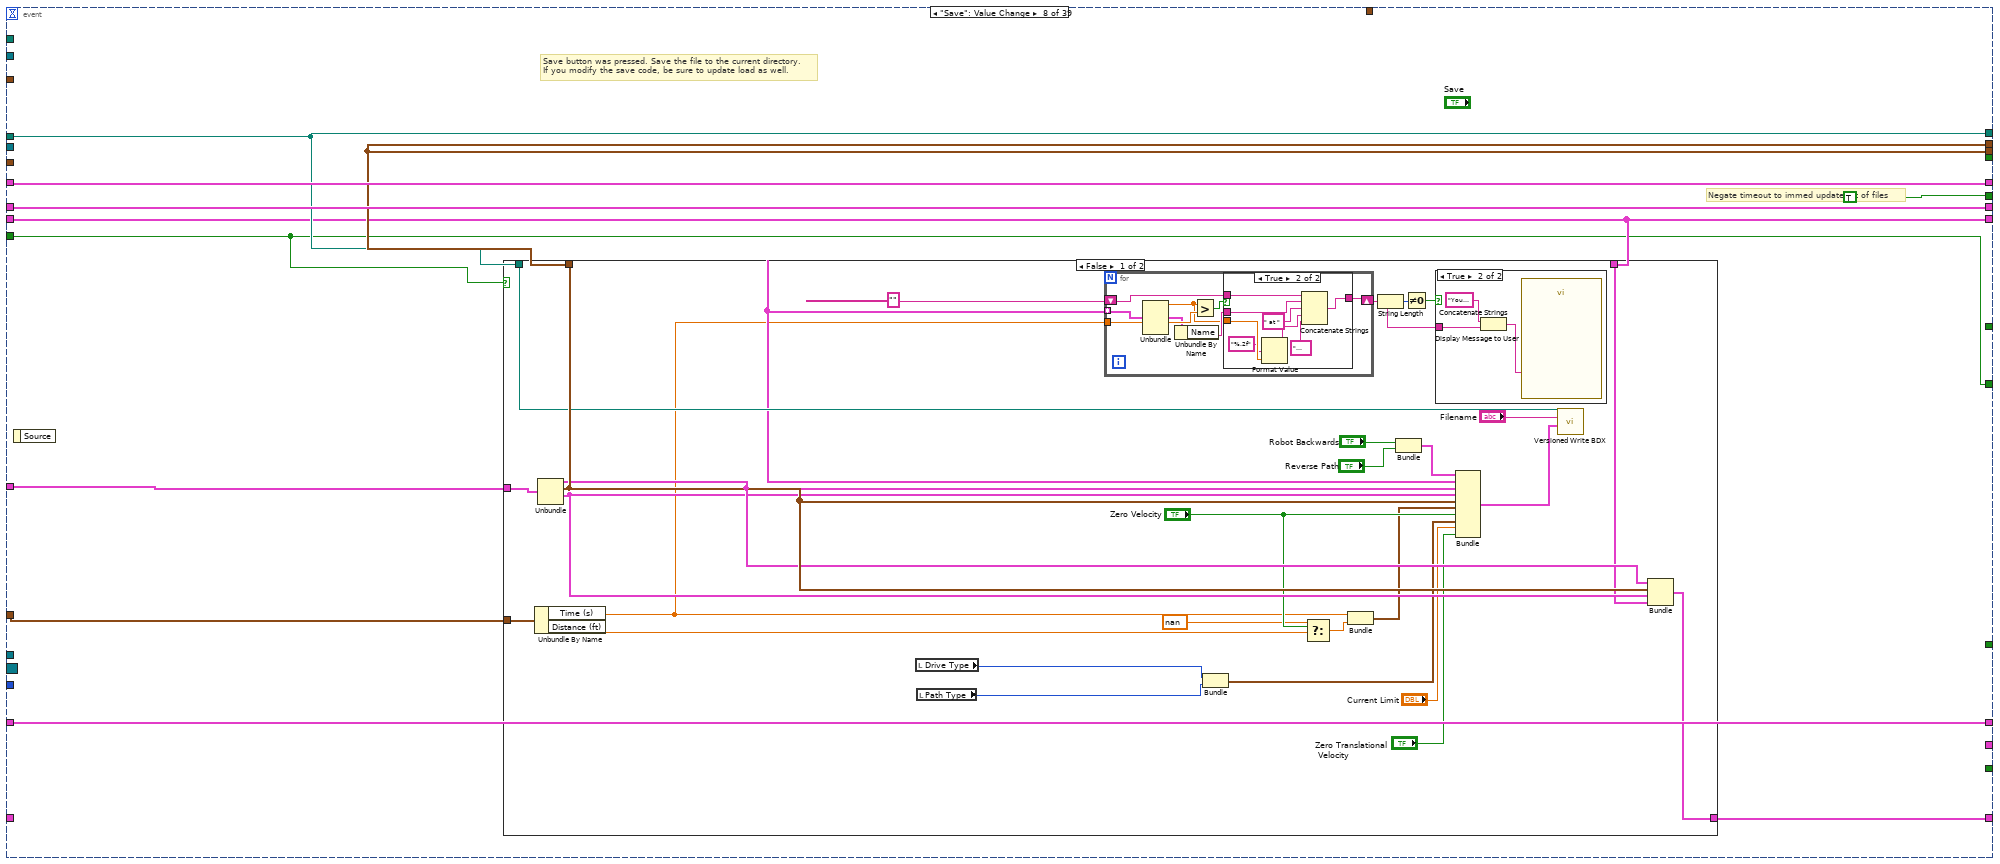
[diagram p18: hidden frame]
diagram:
  w3 = FALSE
  w18 = FALSE ("Visible")
  w21 = T14."Trajectory Settings" ("Tab Control")
  w30 = enum16{"Left", "Center", "Right"}."Right" ("Active Cell:Cell Justification")
  w37 = T17 []
  w51 = -1  # Data
  w48 = T19 {"Index"=0, "Pt Test Results"=enum."Miss"}  # Hover Object
  w47 = cluster{"Index":i32, "x":dbl, "y":dbl} {"Index"=-1, "x"=0.0, "y"=0.0}  # Drag Object
  w59 = cluster{"x":dbl, "y":dbl, "th":dbl}[] [{"x"=13.2083, "y"=31.9375, "th"=-90.0}]  # Initial Location
  # "Saved Program Data"
  # "Command Cache"
  # "File Attributes"
  # "Commands"
  # "Target Refs"
  # "Picture Mouse State"
  # "Auto Data"
  # "Timeout between folder scan\nto update path list"
  # "This should probably turn into an event."
  # "Work on:"
  # "TODO: \nFinish Open to show paths and allow edits to existing path.\nAdd operations such as flip, reverse, maybe stretch."
  n1 = property on="Tab Control" class="TabCtl (strict)"() -> ("Pages"=w9:refnum<vi>[])  [unwired: 2 in, 2 out]
  n2 = invoke on="Tree" class="Tree (strict)" method="Edit Tree Items.Delete"("Delete Children"=TRUE ("Delete Children?")) -> ()  [unwired: 4 in, 5 out]
  n3 = property on="Append" class="Bool"("Visible"=TRUE) -> ()  [unwired: 2 in, 2 out]
  n4 = property on="New" class="Bool"("Visible"=TRUE) -> ()  [unwired: 2 in, 2 out]
  n5 = property on="Delete" class="Bool"("Visible"=TRUE) -> ()  [unwired: 2 in, 2 out]
  n6 = property on="Delete AQT" class="Bool"("Visible"=FALSE) -> ()  [unwired: 2 in, 2 out]
  n7 = property on="Open Aquitaine Editor" class="Bool"("Visible"=FALSE) -> ()  [unwired: 2 in, 2 out]
  n8 = property on="New AQT" class="Bool"("Visible"=FALSE) -> ()  [unwired: 2 in, 2 out]
  n9 = property on="Save" class="Bool"("Visible"=TRUE) -> ()  [unwired: 2 in, 2 out]
  n10 = property on="Push" class="Bool"("Visible"=TRUE) -> ()  [unwired: 2 in, 2 out]
  n11 = property on="Push AQT" class="Bool"("Visible"=w18) -> ()  [unwired: 2 in, 2 out]
  n12 = property on="Push BORAQT" class="Bool"("Visible"=w18) -> ()  [unwired: 2 in, 2 out]
  n13 = Index Array(array=w9, index=6) -> (element=w8:refnum<vi>)
  n14 = Current VI's Path() -> (path=w35:path)
  n15 = property class="Page"(reference=w8) -> ("DecosOnPage"=w6:refnum<vi>[])  [unwired: 1 in, 2 out]
  n16 = property class="VI"() -> (reference out=w26:refnum<vi>, "Panel"=w45:refnum<vi>)  [unwired: 2 in, 1 out]
  n17 = Strip Path(path=w35) -> (stripped path=w34:path)  [unwired: 1 out]
  n18 = Build Path(base path=w34, name or relative path="Bordeaux.ini" ("format string")) -> (appended path=w28:path)
  n19 = property on="New" class="Bool"() -> ("Position"=w41:T18)  [unwired: 2 in, 2 out]
  n20 = local read "Limits"() -> (w56:T9)
  n21 = global write "Global Settings.vi" "Draw Menu Drag Indicator"(w6) -> ()
  n22 = Index Array(array=w6) -> (element #1=w5:refnum<vi>, element #2=w4:refnum<vi>)  [unwired: 2 in]
  n23 = property class="Pnl"(reference=w45) -> ("Panes[]"=w44:refnum<vi>[])  [unwired: 1 in, 2 out]
  n24 = call "Change Paths Directory.vi"("VI Refnum"=w26, "config path"=w28) -> ("Bordeaux paths out"=w27:path)  [unwired: 9 in]
  n25 = local write "Filename"("Untitled" ("Filename")) -> ()
  n26 = Create User Event(user event datatype=w51) -> (user event=w52:refnum<user-event>)  [unwired: 1 in, 1 out]
  n27 = local write "Open"(i32[] [-1] ("Open")) -> ()
  n28 = property on="Property Node" class="Decor"(reference=w5, "Visible"=w3) -> ()  [unwired: 1 in, 2 out]
  n29 = property on="Property Node" class="Decor"(reference=w4, "Visible"=w3) -> ()  [unwired: 1 in, 2 out]
  n30 = Unbundle(w56) -> ("Accel (fps^2)"=w55:dbl)  [unwired: 3 out]
  n31 = Subtract(x=w41, y=T18 {"Left"=40, "Top"=10}) -> (x-y=w40:T18)
  n32 = call <vilib>:"Create Directory Recursive.vi"("directory"=w27) -> ()  [unwired: 4 in, 3 out]
  n33 = Index Array(array=w44) -> (element=w43:refnum<vi>)  [unwired: 1 in]
  n34 = property on="Open" class="MCListbox (strict)"("ActiveCell"=T16 {"Row"=-2, "Column"=1} ("Active Cell:Active Cell"), "Justify"=w30, "ActiveCell"=T16 {"Row"=-2, "Column"=2} ("Active Cell:Active Cell"), "Justify"=w30) -> (error out=w31:errorcluster)  [unwired: 2 in, 1 out]
  n35 = register-events(w52) -> (reference out=w53:refnum<event-registration>)  [unwired: 2 in, 1 out]
  n36 = local write "Overrides"(T8 [{"Count"="", "Angular Override"=0.0, "Enabled?"=FALSE, "Velocity Override"=0.0, "Angle Override"=0.0}] ("Overrides")) -> ()
  n37 = call "Add First Point.vi"("Accel (f/s^2)"=w55, "Time (s)"=1 ("th"), "Initial Points"=w59) -> ("Points"=w50:cluster{"x":dbl, "y":dbl, "th":dbl}[])  [unwired: 8 in]
  n38 = Bundle("Drag Object"=w47, "Hover Object"=w48, "Filename"="") -> (w46:T20)  [unwired: 1 in]
  n39 = local write "New Page Selector"(w21) -> ()
  n40 = local write "File Manager"(enum32{"Bordeaux Files", "Aquitaine Files"}."Bordeaux Files" ("File Manager")) -> ()
  n41 = local write "Tab Control"(w21) -> ()
  n42 = property class="Pane"(reference=w43, "Origin"=w40) -> (error out=w39:errorcluster)  [unwired: 1 in, 1 out]
  n43 = control-ref of="Picture"() -> (w61:refnum<vi>)
  n44 = Bundle("Trajectory Data"=T12 [], "Points"=w50, "output cluster"=T15 {"Sample Period (s)"=0.2, "Limits"={"Velocity (fps)"=6.0, "Accel (fps^2)"=32.0, "Jerk (fps^3)"=1500.0, "StoopidFast (fps)"=12.0}, "Conditions"={"vInitial (fps)"=0.0, "vFinal (fps)"=0.0}, "Overrides"=[], "Angular Limits"={"Velocity (deg/s)"=0.0, "Accel (deg/s^2)"=0.0, "Jerk (deg/s^3)"=0.0}}, w37) -> (w24:T21)  [unwired: 1 in]
  n45 = while {
    tunnel: w50 -> [w129]
    tunnel: w61 -> [w128]
    shift-right: [w105] -> _
    shift-left: 0 -> [w124]
    shift-right: [w80] -> _
    shift-left: _ -> [w123]
    tunnel: w27 -> [w112]
    tunnel: w53 -> [w119]
    tunnel: w52 -> [w118]
    shift-right: [w116] -> _
    shift-left: _ -> [w117]
    shift-right: [w76] -> _
    shift-left: w24 -> [w92]
    shift-right: [w109] -> _
    shift-left: w46 -> [w110]
    shift-right: [w102] -> _
    shift-left: _ -> [w101]
    shift-right: [w99] -> _
    shift-left: "Cache" -> [w100]
    shift-right: [w94] -> _
    shift-left: w37 -> [w97]
    tunnel: w39 -> [_]
    tunnel: cluster{"width":dbl, "height":dbl}[] [{"width"=26.5, "height"=54.25}, {"width"=26.4166, "height"=57.5729}, {"width"=27.0, "height"=35.0}, {"width"=15.0, "height"=30.0}, {"width"=15.0, "height"=30.0}, {"width"=15.0, "height"=30.0}, {"width"=15.0, "height"=30.0}] -> [w89]
    tunnel: [w87] -> _
    tunnel: w31 -> [_]
    tunnel: w28 -> [w83]
    tunnel: w26 -> [w82]
    tunnel: cluster{"width":dbl, "height":dbl, dbl, dbl}[] [{"width"=817.0, "height"=-618.0, 1208.0, 593.0}, {"width"=826.0, "height"=-627.0, 1217.0, 562.0}, {"width"=27.0, "height"=35.0, 0.0, 0.0}, {"width"=15.0, "height"=30.0, 0.0, 0.0}, {"width"=15.0, "height"=30.0, 0.0, 0.0}, {"width"=15.0, "height"=30.0, 0.0, 0.0}, {"width"=15.0, "height"=30.0, 0.0, 0.0}] ("Array") -> [w72]
    shift-right: [w64] -> _
    shift-left: _ -> [w63]
    i -> [w87]
    stop <- FALSE stop-if-true
    # "Correctly sizes override array"
    # "TODO Length from vertex to blends is off because point moved.\nExtra Arc only works when enter line is at 0deg."
    # "TODO enforce points on field"
    n46 = feedback #1(w112) -> (w113:path)
    n47 = event shown="[38] \"Open Aquitaine Editor\": Value Change" {
      selector: w119 -> [_ _ _ _ _ _ _ _ _ _ _ _ _ _ _ _ _ _ _ _ _ _ _ _ _ _ _ _ _ _ _ _ _ _ _ _ _ _ _]
      dyn-events: _ -> [_ _ _ _ _ _ _ _ _ _ _ _ _ _ _ _ _ _ _ _ _ _ _ _ _ _ _ _ _ _ _ _ _ _ _ _ _ _ _]
      timeout: w124 -> [_ _ _ _ _ _ _ _ _ _ _ _ _ _ _ _ _ _ _ _ _ _ _ _ _ _ _ _ _ _ _ _ _ _ _ _ _ _ _]
      tunnel: [w276 w322 w356 w397 w413 w442 w472 w482 w551 w567 w573 w623 w640 w715 w748 w864 w907 w1013 w1041 w1068 w1085 w1108 w1128 w1170 w1220 w1256 w1318 w1348 w1389 w1421 w1439 w1477 w1551 w1592 w1618 w1630 w1653 w1695 w1706] -> w122
      tunnel: w129 -> [_ _ w356 _ _ _ _ _ _ _ _ w623 w641 _ _ _ _ _ _ _ _ _ _ _ _ _ _ _ _ _ _ _ _ _ _ _ _ _ _]
      tunnel: w128 -> [_ _ _ _ _ _ _ _ _ _ _ _ _ _ w747 w850 _ w1000 _ _ _ _ _ _ _ _ _ _ _ _ _ _ _ _ _ _ _ _ _]
      tunnel: w113 -> [w242 w320 w364 w386 w421 w441 w477 w481 w543 w563 w572 w620 w645 w714 w745 w861 w921 w1014 w1055 w1071 w1087 w1114 w1132 w1174 w1226 w1261 w1322 w1353 w1394 w1426 w1437 w1484 w1563 w1600 w1627 w1637 w1652 w1697 w1704]
      tunnel: [w276 w322 w361 w397 w413 w442 w472 w482 w551 w567 w573 w621 w643 w715 w742 w858 w899 w998 w1041 w1068 w1085 w1108 w1128 w1170 w1220 w1256 w1318 w1348 w1389 w1421 w1439 w1477 w1551 w1592 w1618 w1630 w1653 w1695 w1706] -> w121
      tunnel: w123 -> [_ _ _ _ _ _ _ w480 _ _ _ _ _ _ _ _ _ _ _ _ _ _ _ _ _ _ _ _ _ _ _ _ _ _ _ _ _ _ _]
      tunnel: [_ _ w355 TRUE ("Flip Over Center") _ _ _ _ _ _ _ _ TRUE ("Flip Over Center") _ _ _ TRUE ("Flip Over Center") _ _ _ _ _ _ _ _ _ _ _ _ _ _ _ _ _ _ _ _ _ _] -> w81
      tunnel: [w242 w320 w364 w386 w421 w441 w477 w481 w543 w556 w572 w620 w645 w714 w745 w861 w921 w1014 w1055 w1071 w1087 w1114 w1132 w1174 w1226 w1261 w1322 w1353 w1394 w1426 w1437 w1484 w1563 w1600 w1627 w1637 w1652 w1697 w1704] -> w68
      tunnel: w118 -> [_ _ _ _ _ _ w476 _ _ _ _ _ _ _ _ _ _ _ w1036 _ _ _ _ _ _ _ _ _ _ _ _ _ _ _ _ _ _ _ _]
      tunnel: [w278 w327 w363 w387 w420 w449 w475 w488 w553 w569 w580 w628 w650 w722 w744 w860 w920 w1001 w1053 w1070 w1088 w1113 w1131 w1173 w1225 w1260 w1321 w1352 w1393 w1425 w1445 w1483 w1562 w1599 w1626 w1636 w1659 w1702 w1712] -> w116
      tunnel: w117 -> [w278 w327 w363 w387 w420 w449 w475 _ w553 w569 w580 w628 w650 _ w744 w860 w920 w1001 w1053 w1070 w1088 w1113 w1131 w1173 w1225 w1260 w1321 w1352 w1393 w1425 w1445 w1483 w1562 w1599 w1626 w1636 w1659 w1702 w1712]
      tunnel: w92 -> [w277 w323 w362 w385 w414 w443 w473 w487 w552 w568 w574 w622 w644 _ w743 w859 w919 w999 w1042 w1069 w1086 _ w1129 w1171 w1222 w1257 w1319 w1349 w1390 w1422 w1440 w1478 w1552 w1593 w1619 w1631 w1654 w1696 w1707]
      tunnel: w110 -> [w275 w326 w360 w384 w419 w448 w471 w486 w548 w570 w579 w627 w649 w730 w739 w851 w918 w996 w1040 w1067 w1084 w1112 w1127 w1169 w1224 w1259 w1304 w1351 w1392 w1424 w1444 w1482 w1561 w1598 w1625 w1635 w1658 w1701 w1711]
      tunnel: [w275 w326 w360 w384 w419 w448 w471 w486 w549 w570 w579 w627 w649 w730 w741 w855 w918 w996 w1040 w1067 w1084 w1112 w1127 w1169 w1224 w1259 w1305 w1351 w1392 w1424 w1444 w1482 w1561 w1598 w1625 w1635 w1658 w1701 w1711] -> w109
      tunnel: [_ _ _ _ _ _ _ TRUE _ TRUE _ _ _ _ _ _ _ _ _ _ _ _ _ _ _ _ _ _ _ _ _ _ _ _ _ _ _ _ _] -> w104
      tunnel: [w274 w321 w358 w383 w418 w447 w470 w484 w542 w561 w578 w626 w648 w729 w735 w853 w917 w994 w1039 w1062 w1081 w1111 w1130 w1172 w1223 w1258 w1320 w1350 w1391 w1423 w1443 w1481 w1560 w1597 w1624 w1634 w1657 w1700 w1703] -> w102
      tunnel: w101 -> [w274 w321 w358 w383 w418 w447 w470 w484 w542 w561 w578 w626 w648 w729 w735 w853 w917 w994 w1039 w1065 w1081 w1111 w1130 w1172 w1223 w1258 w1320 w1350 w1391 w1423 w1443 w1481 w1560 w1597 w1624 w1634 w1657 w1700 w1703]
      tunnel: w100 -> [w273 w325 w359 w382 w417 w446 w469 w483 w541 w560 w577 w625 w647 w728 w737 w852 w916 w993 w1038 w1064 _ w1110 w1116 w1162 w1213 w1243 w1302 w1338 w1380 w1409 w1442 w1480 w1559 w1596 w1623 w1633 w1656 w1699 w1710]
      tunnel: [w273 w325 w359 w382 w417 w446 w469 w483 w541 w560 w577 w625 w647 w728 w737 w852 w916 w993 w1038 w1064 w1083 w1110 w1116 w1162 w1213 w1243 w1302 w1338 w1380 w1409 w1442 w1480 w1559 w1596 w1623 w1633 w1656 w1699 w1710] -> w99
      tunnel: 35 -> [_ _ _ _ _ _ _ _ _ _ _ _ _ _ _ _ _ _ _ _ _ _ _ _ _ _ _ _ w1382 w1417 _ _ _ _ _ _ _ _ _]
      tunnel: w97 -> [w272 w324 _ w381 w416 w445 w468 w479 w550 w558 w576 w624 w642 _ w736 w849 w915 w992 w1037 w1063 w1082 w1109 w1117 w1160 w1218 w1246 w1307 w1341 w1381 w1411 w1441 w1479 w1558 w1595 w1622 w1632 w1655 w1698 w1709]
      tunnel: [w272 w324 _ w381 w416 w445 w468 w479 w550 w558 w576 w624 w642 w726 w736 w849 w915 w992 w1037 w1063 w1082 w1109 w1117 w1164 w1219 w1244 w1307 w1336 w1381 w1408 w1441 w1479 w1558 w1595 w1622 w1632 w1655 w1698 w1709] -> w96
      tunnel: [w271 _ w355 TRUE ("First Call?: T/F") _ _ _ _ _ _ _ _ TRUE ("First Call?: T/F") TRUE _ _ _ _ _ _ _ _ w1120 w1163 TRUE w1245 _ w1340 _ TRUE _ _ _ _ _ _ _ _ _] -> w95
      tunnel: w89 -> [w260 _ _ _ _ _ _ _ _ _ _ _ _ _ _ w839 w906 w985 _ _ _ _ _ _ _ _ _ _ _ _ _ _ _ _ _ _ _ _ _]
      tunnel: w83 -> [_ _ _ _ _ _ _ _ _ w557 _ _ _ _ _ _ _ _ _ _ _ _ _ _ _ _ _ _ _ _ _ _ _ _ _ _ _ _ _]
      tunnel: w82 -> [_ _ _ _ _ _ _ _ _ w555 _ _ _ _ _ _ _ _ _ _ _ _ _ _ _ _ _ _ _ _ _ _ _ _ _ _ _ _ _]
      tunnel: w72 -> [w251 _ _ _ _ _ _ _ _ _ _ _ _ _ _ _ _ _ _ _ _ _ _ _ _ _ _ _ _ _ _ _ _ _ _ _ _ _ _]
      tunnel: [_ _ _ _ _ _ _ _ _ _ _ _ _ _ _ _ _ _ _ _ _ _ _ _ _ _ _ _ _ _ _ _ _ _ TRUE _ TRUE _ _] -> w71
      tunnel: [_ _ _ _ _ _ _ _ _ _ _ _ _ _ _ _ _ _ _ _ _ _ _ _ _ _ _ _ _ _ _ _ _ _ w1613 _ w1644 _ _] -> w70
      tunnel: [_ _ _ _ _ _ _ _ _ _ _ _ _ _ _ _ _ _ _ _ _ _ _ _ _ _ _ _ _ _ _ _ _ _ _ _ _ w1694 _] -> _
      tunnel: [w240 w297 w354 w365 w412 w440 w467 w478 w539 w554 w571 w614 w637 FALSE w734 w837 w894 w983 w1034 w1060 w1077 w1107 w1115 w1159 w1212 w1241 w1300 w1335 w1379 w1407 w1436 w1465 w1548 w1591 w1612 w1628 w1642 TRUE w1708] -> w64
      tunnel: w63 -> [w240 w297 w354 w365 w412 w440 w467 w478 w539 w554 w571 w614 w637 _ w734 w837 w894 w983 w1034 w1060 w1077 w1107 w1115 w1159 w1212 w1241 w1300 w1335 w1379 w1407 w1436 w1465 w1548 w1591 w1612 w1628 w1642 _ w1708]
      event Timeout; "Background", "Robot Color", "Robot Size (in)": Value Change {
        # "Occasionally update the listbox with all files in\nthe folder.\nAlso update the size of the picture, which field button\nis shown, color of the robot arrow,"
        n48 = event-data() -> ()  [unwired: 1 in, 1 out]
        n49 = Unbundle(w277) -> ("Updated Waypoints"=w276:cluster{"x":dbl, "y":dbl, "th":dbl}[])  [unwired: 3 out]
        n50 = call <vilib>:"Recursive File List.vi"("pattern"="*.bdx", "Folder Path"=w242) -> ("error out"=w279:errorcluster, "All Files in Dir"=w281:path[])  [unwired: 5 in, 3 out]
        n51 = call <vilib>:"Recursive File List.vi"("pattern"="*.aqt", "Folder Path"=w242) -> ("All Files in Dir"=w241:path[])  [unwired: 5 in, 4 out]
        n52 = Divide(x="Robot Size (in)", y=24.0 ("width")) -> (x/y=w267:cluster{"width":dbl, "height":dbl})
        n53 = Negate(x=w267) -> (-x=w268:cluster{"width":dbl, "height":dbl})
        n54 = for {
          tunnel: w281 -> [w294] mode=indexing
          tunnel: [w296] -> w280 mode=indexing
          tunnel: w279 -> [_]
          workers-P: _ -> [_]
          w288 = "%.3f" ("format string")
          n55 = call "Versioned Load BDX.vi"("path"=w294) -> ("Overall"=w293:cluster{"Time (s)":dbl, "Distance (ft)":dbl})  [unwired: 17 in, 9 out]
          n56 = Strip Path(path=w294) -> (name=w295:string)  [unwired: 1 out]
          n57 = Unbundle(w293) -> ("Time (s)"=w292:dbl, "Distance (ft)"=w291:dbl)
          n58 = Format Into String(format string=w288, w292) -> (resulting string=w290:string)  [unwired: 2 in, 1 out]
          n59 = Format Into String(format string=w288, w291) -> (resulting string=w289:string)  [unwired: 2 in, 1 out]
          n60 = Build Array(w295, w290, w289) -> (w296:string[])
        }
        n61 = Unbundle(w268) -> ("width"=w266:dbl, "height"=w265:dbl)
        n62 = Unbundle(w267) -> ("width"=w264:dbl, "height"=w263:dbl)
        n63 = Index Array(array=w260, index="Background") -> (element=w259:cluster{"width":dbl, "height":dbl})
        "Field Size (ft)" <- w259
        n64 = Bundle("width"=w266, "height"=w265, "width"=w264, "height"=w263) -> (w262:T29)  [unwired: 1 in]
        n65 = global write "Global Settings.vi" "Field Size"(w259) -> ()
        n66 = for {
          tunnel: w241 -> [w287] mode=indexing
          workers-P: _ -> [_]
          n67 = control-ref of="Tree"() -> (w282:refnum<vi>)
          n68 = call "GetTreeIndentLevel0.vi"("Tree 2"=w282) -> ("Indent Level 0"=w286:string[])  [unwired: 10 in]
          n69 = Strip Path(path=w287) -> (name=w283:string)  [unwired: 1 out]
          n70 = call "Add AQT to Tree.vi"("Current AQT List"=w286, "AQT Name"=w283, "TreeControl in"=w282) -> ("error out"=w284:errorcluster)  [unwired: 8 in]
          n71 = call "Add BDX to Tree.vi"("AQT Name"=w283, "error in (no error)"=w284, "Path"=w287, "TreeControl in"=w282) -> ()  [unwired: 8 in]
          n72 = call "GetTreeIndentLevel0.vi"("error in (no error)"=w284, "Tree 2"=w282) -> ("Indent Level 0"=w285:string[])  [unwired: 9 in]
          n73 = property on="Aquitaine Add Selector" class="Ring (strict)"("Strings []"=w285) -> ()  [unwired: 2 in, 2 out]
        }
        n74 = global write "Global Settings.vi" "Robot Rect"(w262) -> ()
        n75 = Equal To 0?(x="Background") -> (x = 0?=w257:bool)
        n76 = Select(t=FALSE, s=w257, f=TRUE) -> (s? t:f=w255:bool)
        "RS" <- w255
        n77 = Not(x=w255) -> (.not. x?=→"?":bool)
        n78 = property on="Open" class="MCListbox (strict)"("ItemNames"=w280) -> ()  [unwired: 2 in, 2 out]
        n79 = Index Array(array=w251, index="Background") -> (element=w250:cluster{"width":dbl, "height":dbl, dbl, dbl})
        n80 = global write "Global Settings.vi" "Arrow Color"("Robot Color") -> ()
        n81 = Unbundle(w250) -> ("width"=w249:dbl, "height"=w248:dbl, w245:dbl, w244:dbl)
        n82 = Bundle("width"=w249, "height"=w248) -> (w247:cluster{"width":dbl, "height":dbl})  [unwired: 1 in]
        n83 = Bundle(w244, w245) -> (w246:cluster{dbl, dbl})  [unwired: 1 in]
        n84 = property on="Picture" class="Pict"("Position"=w247) -> ()  [unwired: 2 in, 2 out]
        n85 = property on="Picture" class="Pict"("Draw Area Size"=w246) -> ()  [unwired: 2 in, 2 out]
        n86 = First Call?() -> (First Call?: T/F=w271:bool)
      }
      event "Push": Value Change {
        # "Times out after\n5s"
        n87 = event-data() -> ()  [unwired: 1 in, 6 out]
        n88 = call <vilib>:"Set Busy.vi"() -> ("error out"=w299:errorcluster)  [unwired: 10 in, 1 out]
        n89 = local read "Open"() -> (w315:i32[])
        n90 = property on="Open" class="MCListbox (strict)"(error in=w299) -> ("ItemNames"=w314:string[][])  [unwired: 1 in, 2 out]
        n91 = Array Size(array=w315) -> (size(s)=w316:i32)
        n92 = Index Array(array=w315) -> (element=w317:i32)  [unwired: 1 in]
        n93 = Unbundle(w323) -> ("Updated Waypoints"=w322:cluster{"x":dbl, "y":dbl, "th":dbl}[])  [unwired: 3 out]
        n94 = Array Subset(array=w314, index (row)=w317, length (row)=w316) -> (w313:string[][])  [unwired: 2 in]
        n95 = for {
          tunnel: w313 -> [w353] mode=indexing
          tunnel: w320 -> [w347]
          tunnel: [w348] -> w312 mode=indexing
          n96 = Index Array(array=w353, index=0) -> (element=w346:string)
          n97 = Build Path(base path=w347, name or relative path=w346) -> (appended path=w345:path)
          n98 = Concatenate Strings("/home/lvuser/natinst/bin/Paths/" ("string"), w346) -> (w350:string)
          n99 = Bundle(w350, "appended path"=w345, TRUE) -> (w348:cluster{string, "appended path":path, bool})  [unwired: 1 in]
        }
        n100 = String To IP() -> (0:w306:u32)  [unwired: 1 in]
        n101 = IP To String(1:TRUE ("dot notation? (F)"), 2:w306) -> (0:w300:string)
        n102 = String Subset(string=w300, length (rest)=9 ("length (rest)")) -> (substring=w303:string)  [unwired: 1 in]
        n103 = Concatenate Strings(w303, "2" ("string")) -> (w301:string)
        n104 = call "Put Multiple Files.vi"("active (T)"=FALSE, "password"="", "user"="anonymous", "Open Connection Timeout (ms)"=5000.0, "file specifications"=w312, "host"=w301) -> ("error out"=w308:errorcluster, "file errors"=w309:errorcluster[])  [unwired: 4 in]
        n105 = Merge Errors(w309, w308) -> (w307:errorcluster)
        n106 = case shown="Error .." w307 {
          selector: w307 -> [_ w332]
          tunnel: [w328 w329] -> w298
          frame No Error {
            n107 = call "Successful"() -> ("error out"=w328:errorcluster)  [unwired: 10 in, 1 out]
          }
          frame Error {
            n108 = Equal?(x=w332, y=errorcluster {"status"=TRUE, "code"=56, "source"=""}) -> (x = y?=w336:T30)
            n109 = Unbundle By Name(w336) -> ("status"=w335:bool, "code"=w334:bool)
            n110 = Unbundle By Name(w332) -> ("code"=w330:i32, "source"=w331:string)
            n111 = And(x=w335, y=w334) -> (x .and. y?=w333:bool)
            n112 = case shown="True" w333 {
              tunnel: w331 -> [w342 _]
              tunnel: w330 -> [w341 _]
              tunnel: [w338 w344] -> w329
              frame False {
                n113 = Number To Decimal String(number=w341) -> (decimal integer string=w340:string)  [unwired: 1 in]
                n114 = Concatenate Strings("Error pushing the paths. Please see below for details:\n" ("string"), w342, w340) -> (w339:string)
                n115 = call "Error"("Message"=w339) -> ("error out"=w338:errorcluster)  [unwired: 9 in, 1 out]
              }
              frame True {
                n116 = call "Error"() -> ("error out"=w344:errorcluster)  [unwired: 10 in, 1 out]
              }
            }
          }
        }
        n117 = call <vilib>:"Unset Busy.vi"("error in (no error)"=w298) -> ()  [unwired: 10 in, 1 out]
      }
      event "New": Value Change {
        w355 = TRUE
        # "Button was pushed. Create a new trajectory path"
        # "Use Initial Location"
        n118 = event-data() -> ()  [unwired: 1 in, 5 out]
        n119 = Unbundle(w362) -> ("Updated Waypoints"=w361:cluster{"x":dbl, "y":dbl, "th":dbl}[])  [unwired: 3 out]
        n120 = local write "Conditions"(T10 {"vInitial (fps)"=0.0, "vFinal (fps)"=0.0} ("Conditions")) -> ()
      }
      event "Append": Value Change {
        # "Append button was pressed. Create a trajectory file that adopts the current position, heading, and start velocity"
        n121 = event-data() -> ()  [unwired: 1 in, 1 out]
        n122 = Unbundle(w385) -> ("Updated Waypoints"=w366:cluster{"x":dbl, "y":dbl, "th":dbl}[])  [unwired: 3 out]
        n123 = Array Size(array=w366) -> (size(s)=w375:i32)
        n124 = Decrement(x=w375) -> (x-1=w373:i32)
        n125 = Decrement(x=w373) -> (x-1=w374:i32)
        n126 = Index Array(array=w366, index=w373) -> (element=w378:cluster{"x":dbl, "y":dbl, "th":dbl})
        n127 = Index Array(array=w366, index=w374) -> (element=w372:cluster{"x":dbl, "y":dbl, "th":dbl})
        n128 = Unbundle(w378) -> ("x"=w371:dbl, "y"=w370:dbl, "th"=w377:dbl)
        n129 = Unbundle(w372) -> ("x"=w369:dbl, "y"=w368:dbl)  [unwired: 1 out]
        n130 = Not A Number/Path/Refnum?(number/path/refnum=w377) -> (NaN/Path/Refnum?=w376:bool)
        n131 = case shown="True" w376 {
          tunnel: w371 -> [_ w409]
          tunnel: w370 -> [_ w408]
          tunnel: w369 -> [_ w411]
          tunnel: w368 -> [_ w410]
          tunnel: [w399 w405] -> w367
          tunnel: w366 -> [w399 w407]
          frame False {
          }
          frame True {
            n132 = Subtract(x=w409, y=w411) -> (x-y=w400:dbl)
            n133 = Subtract(x=w408, y=w410) -> (x-y=w401:dbl)
            n134 = Delete From Array(array=w407) -> (array with subset deleted=w406:cluster{"x":dbl, "y":dbl, "th":dbl}[])  [unwired: 2 in, 1 out]
            n135 = Inverse Tangent (2 Input)(1:w400, 2:w401) -> (0:w404:dbl)
            n136 = expression code="(x/pi)*180.0" "radians to degrees"(w404) -> (w403:dbl)
            n137 = Bundle("x"=w409, "y"=w408, w403) -> (w402:cluster{"x":dbl, "y":dbl, dbl})  [unwired: 1 in]
            n138 = Build Array (concatenate)(w406, w402) -> (w405:cluster{"x":dbl, "y":dbl, "th":dbl}[])
          }
        }
        n139 = local read "Conditions"() -> (w394:T10)
        n140 = local read "Limits"() -> (w390:T9)
        n141 = Unbundle(w390) -> ("Velocity (fps)"=w389:dbl, "Accel (fps^2)"=w388:dbl)  [unwired: 2 out]
        n142 = Delete From Array(array=w367) -> (deleted portion=w396:cluster{"x":dbl, "y":dbl, "th":dbl})  [unwired: 2 in, 1 out]
        n143 = Divide(x=w389, y=w388) -> (x/y=w398:dbl)
        n144 = Build Array(w396) -> (w395:cluster{"x":dbl, "y":dbl, "th":dbl}[])
        n145 = Unbundle(w394) -> ("vFinal (fps)"=w393:dbl)  [unwired: 1 out]
        n146 = call "Add First Point.vi"("Accel (f/s^2)"=w388, "Time (s)"=w398, "Initial Points"=w395) -> ("Points"=w397:cluster{"x":dbl, "y":dbl, "th":dbl}[])  [unwired: 8 in]
        n147 = Bundle("vFinal (fps)"=w393, 0.0) -> (w392:cluster{"vFinal (fps)":dbl, dbl})  [unwired: 1 in]
        n148 = local write "Conditions"(w392) -> ()
      }
      event "File Manager": Value Change {
        n149 = event-data() -> ("NewVal"=w415:enum32{"Bordeaux Files", "Aquitaine Files"})  [unwired: 1 in, 5 out]
        n150 = case shown="\"Bordeaux Files\", Default" w415 {
          frame "Bordeaux Files", Default {
            w424 = FALSE ("Visible")
            n151 = property on="New" class="Bool"("Visible"=TRUE) -> ()  [unwired: 2 in, 2 out]
            n152 = property on="Delete" class="Bool"("Visible"=TRUE) -> ()  [unwired: 2 in, 2 out]
            n153 = property on="Delete AQT" class="Bool"("Visible"=FALSE) -> ()  [unwired: 2 in, 2 out]
            n154 = property on="New AQT" class="Bool"("Visible"=FALSE) -> ()  [unwired: 2 in, 2 out]
            n155 = property on="Save" class="Bool"("Visible"=TRUE) -> ()  [unwired: 2 in, 2 out]
            n156 = property on="Push" class="Bool"("Visible"=TRUE) -> ()  [unwired: 2 in, 2 out]
            n157 = property on="Push AQT" class="Bool"("Visible"=w424) -> ()  [unwired: 2 in, 2 out]
            n158 = property on="Push BORAQT" class="Bool"("Visible"=w424) -> ()  [unwired: 2 in, 2 out]
            n159 = property on="Append" class="Bool"("Visible"=TRUE) -> ()  [unwired: 2 in, 2 out]
            n160 = property on="Open Aquitaine Editor" class="Bool"("Visible"=FALSE) -> ()  [unwired: 2 in, 2 out]
          }
          frame "Aquitaine Files" {
            w433 = TRUE ("Visible")
            n161 = property on="Delete AQT" class="Bool"("Visible"=TRUE) -> ()  [unwired: 2 in, 2 out]
            n162 = property on="New" class="Bool"("Visible"=FALSE) -> ()  [unwired: 2 in, 2 out]
            n163 = property on="Delete" class="Bool"("Visible"=FALSE) -> ()  [unwired: 2 in, 2 out]
            n164 = property on="New AQT" class="Bool"("Visible"=TRUE) -> ()  [unwired: 2 in, 2 out]
            n165 = property on="Save" class="Bool"("Visible"=FALSE) -> ()  [unwired: 2 in, 2 out]
            n166 = property on="Push" class="Bool"("Visible"=FALSE) -> ()  [unwired: 2 in, 2 out]
            n167 = property on="Push AQT" class="Bool"("Visible"=w433) -> ()  [unwired: 2 in, 2 out]
            n168 = property on="Push BORAQT" class="Bool"("Visible"=w433) -> ()  [unwired: 2 in, 2 out]
            n169 = property on="Append" class="Bool"("Visible"=FALSE) -> ()  [unwired: 2 in, 2 out]
            n170 = property on="Open Aquitaine Editor" class="Bool"("Visible"=TRUE) -> ()  [unwired: 2 in, 2 out]
          }
        }
        n171 = Unbundle(w414) -> ("Updated Waypoints"=w413:cluster{"x":dbl, "y":dbl, "th":dbl}[])  [unwired: 3 out]
      }
      event "New AQT": Value Change {
        n172 = event-data() -> ("NewVal"=w444:bool)  [unwired: 1 in, 5 out]
        n173 = case shown="True" w444 {
          tunnel: w441 -> [_ w452]
          frame False {
          }
          frame True {
            n174 = local read "Filename"() -> (w453:string)
            n175 = Build Path(base path=w452, name or relative path=w453) -> (appended path=w454:path)
            n176 = call <vilib>:"Get File Extension.vi"("file"=w454) -> ("lowercase file extension"=w455:string, "dup file"=w456:path)  [unwired: 6 in, 3 out]
            n177 = case shown="Default" w455 {
              tunnel: w456 -> [w464 w466]
              tunnel: [w461 w466] -> w450
              frame Default {
                n178 = Strip Path(path=w464) -> (stripped path=w462:path, name=w463:string)
                n179 = Concatenate Strings(w463, ".aqt") -> (w460:string)
                n180 = Build Path(base path=w462, name or relative path=w460) -> (appended path=w461:path)
              }
              frame "aqt" {
              }
            }
            n181 = call <vilib>:"Check if File or Folder Exists.vi"("path"=w450) -> ("file or folder exists?"=w451:bool)  [unwired: 8 in, 2 out]
            n182 = case shown="False" w451 {
              tunnel: w450 -> [_ w459]
              frame True {
                n183 = One Button Dialog(message="Cannot Allow Duplicate Filenames") -> ()  [unwired: 1 in, 1 out]
              }
              frame False {
                n184 = call "Versioned Write AQT.vi"("data"=T24 {"Path References"=[], "Decision Tree"={"Tree"=[], "Node To Index Lookup Map"={}}} ("Aquitaine Data"), "Aquitaine paths in"=w459) -> ()  [unwired: 9 in, 1 out]
              }
            }
          }
        }
        n185 = Unbundle(w443) -> ("Updated Waypoints"=w442:cluster{"x":dbl, "y":dbl, "th":dbl}[])  [unwired: 3 out]
      }
      event "Play": Value Change {
        # "Play button was pressed. Start playing the path by firing the event where it will self-feed."
        n186 = event-data() -> ()  [unwired: 1 in, 1 out]
        n187 = Unbundle(w473) -> ("Updated Waypoints"=w472:cluster{"x":dbl, "y":dbl, "th":dbl}[])  [unwired: 3 out]
        n188 = Tick Count (ms)() -> (millisecond timer value=w474:u32)
        n189 = Generate User Event(user event=w476, event data cluster=w474) -> ()  [unwired: 2 in, 2 out]
      }
      event "Save": Value Change {
        # "Negate timeout to immed update list of files"
        # "Save button was pressed. Save the file to the current directory.\nIf you modify the save code, be sure to update load as well."
        n190 = event-data() -> ()  [unwired: 1 in, 1 out]
        n191 = case shown="False" w478 {
          tunnel: [w516 w537] -> w488
          tunnel: w487 -> [w515 w537]
          tunnel: [w511 w538] -> w482
          tunnel: w481 -> [w508 _]
          tunnel: w480 -> [w503 _]
          tunnel: w479 -> [w497 _]
          frame False {
            n192 = Unbundle By Name(w503) -> ("Time (s)"=w496:dbl, "Distance (ft)"=w501:dbl)
            n193 = Unbundle(w515) -> ("Trajectory Data"=w510:T12, "Updated Waypoints"=w511:cluster{"x":dbl, "y":dbl, "th":dbl}[], w509:T15)  [unwired: 1 out]
            n194 = local read "Drive Type"() -> (w506:T11)
            n195 = local read "Path Type"() -> (w505:T7)
            n196 = for {
              tunnel: w497 -> [w527] mode=indexing
              tunnel: w496 -> [w526]
              shift-right: [w523] -> w492
              shift-left: "" -> [w525]
              n197 = Unbundle(w527) -> ("Start Time (s)"=w521:dbl, w520:T3)  [unwired: 3 out]
              n198 = Unbundle By Name(w520) -> ("Name"=w522:string)
              n199 = Greater?(x=w521, y=w526) -> (0:w524:bool)
              n200 = case shown="True" w524 {
                tunnel: w525 -> [w528 w536]
                tunnel: [w528 w535] -> w523
                tunnel: w522 -> [_ w532]
                tunnel: w521 -> [_ w534]
                frame False {
                }
                frame True {
                  n201 = Format Value(format string="%.2f", value (0)=w534) -> (output string=w530:string)  [unwired: 1 in]
                  n202 = Concatenate Strings(w536, w532, " at " ("string"), w530, " seconds \n" ("string")) -> (w535:string)
                }
              }
            }
            n203 = Bundle("Drive Type"=w506, "Path Type"=w505) -> (w504:cluster{"Drive Type":T11, "Path Type":T7})  [unwired: 1 in]
            n204 = Select(t=nan, s="Zero Velocity", f=w501) -> (s? t:f=w499:dbl)
            n205 = Bundle("Time (s)"=w496, "Distance (ft)"=w499) -> (w498:cluster{"Time (s)":dbl, "Distance (ft)":dbl})  [unwired: 1 in]
            n206 = String Length(string=w492) -> (length=w494:i32)
            n207 = Bundle("Robot Backwards"="Robot Backwards", "Reverse Path"="Reverse Path") -> (w512:T31)  [unwired: 1 in]
            n208 = Not Equal To 0?(x=w494) -> (x != 0?=w493:bool)
            n209 = case shown="True" w493 {
              tunnel: w492 -> [_ w518]
              frame False {
              }
              frame True {
                n210 = Concatenate Strings("You have command(s) that will not be executed during this path.\nThese include:\n", w518) -> (w517:string)
                n211 = call "Display Message to User"("Message"=w517) -> ()  [unwired: 9 in, 2 out]
              }
            }
            n212 = Bundle(w512, "Trajectory Data"=w510, "Commands out"=w497, w509, "Updated Waypoints"=w511, w498, "Zero Velocity"="Zero Velocity", w504, "Current Limit"="Current Limit", "Zero Translational\n Velocity"="Zero Translational\n Velocity") -> (w489:T32)  [unwired: 1 in]
            n213 = call "Versioned Write BDX.vi"("Path Stuff"=w489, "Filename"="Filename", "Bordeaux paths in"=w508) -> ()  [unwired: 9 in]
            n214 = Bundle("Trajectory Data"=w510, "Updated Waypoints"=w511, w509, "Commands out"=w497) -> (w516:T33)  [unwired: 1 in]
          }
          frame True {
            n215 = Unbundle(w537) -> ("Updated Waypoints"=w538:cluster{"x":dbl, "y":dbl, "th":dbl}[])  [unwired: 3 out]
          }
        }
      }
      event "Open Command": Value Change {
        # "Open Panel button was pressed. Open the subVI for the selected command"
        n216 = event-data() -> ()  [unwired: 1 in, 1 out]
        n217 = Unbundle(w552) -> ("Updated Waypoints"=w551:cluster{"x":dbl, "y":dbl, "th":dbl}[])  [unwired: 3 out]
        n218 = Unbundle(w541) -> ("Filtered Command Info Out"=w540:T2)  [unwired: 2 out]
        n219 = call "Open Command Panel.vi"("Cached Commands"=w540, "Commands"=w550, "Tag"="Command Sequence") -> ("Found"=w547:bool)  [unwired: 8 in]
        n220 = Select(t="Command Sequence", s=w547, f="") -> (s? t:f=w544:string)
        n221 = Bundle(cluster=w548, "Filename"=w544) -> (w549:T20)  [unwired: 2 in]
      }
      event "Directory": Value Change {
        # "Negate timeout to immed update list of files"
        # "Directory button was pressed. Put up a file dialog to let the user choose a new directory for loading and saving paths.\nUpdate the titlebar."
        n222 = event-data() -> ()  [unwired: 1 in, 1 out]
        n223 = Unbundle(w568) -> ("Updated Waypoints"=w567:cluster{"x":dbl, "y":dbl, "th":dbl}[])  [unwired: 3 out]
        n224 = call "File Dialog"("start path"=w563, "prompt"="Path Folder", "button label"="Select") -> ("selected path"=w562:path, "error out"=w564:errorcluster)  [unwired: 9 in, 2 out]
        n225 = Select(t=w563, s=w564, f=w562) -> (s? t:f=w556:path)
        n226 = call "Change Paths Directory.vi"("VI Refnum"=w555, "config path"=w557, "Bordeaux paths directory"=w556) -> ()  [unwired: 8 in, 1 out]
      }
      event "Delete AQT": Value Change {
        n227 = event-data() -> ("NewVal"=w575:bool)  [unwired: 1 in, 5 out]
        n228 = case shown="True" w575 {
          tunnel: w572 -> [_ w585]
          frame False {
          }
          frame True {
            n229 = property on="Tree" class="Tree (strict)"() -> ("Value"=w583:string[])  [unwired: 2 in, 2 out]
            n230 = Index Array(array=w583) -> (element=w582:string)  [unwired: 1 in]
            n231 = invoke on="Tree" class="Tree (strict)" method="Navigate Tree.Get Parent"("tag"=w582) -> ("Navigate Tree:Get Parent"=w581:string)  [unwired: 3 in, 3 out]
            n232 = Empty String/Path?(string/path=w581) -> (empty?=w584:bool)
            n233 = case shown="False" w584 {
              tunnel: w583 -> [w592 w600]
              tunnel: w585 -> [w590 w599]
              tunnel: w581 -> [w591 _]
              frame False {
                n234 = Build Path(base path=w590, name or relative path=w591) -> (appended path=w589:path)
                n235 = call "Versioned Load AQT.vi"("Path"=w589) -> ("data"=w588:T34)  [unwired: 10 in]
                n236 = Unbundle(w588) -> ("Path References"=w593:path[])  [unwired: 1 out]
                n237 = for {
                  tunnel: w593 -> [w595] mode=indexing
                  tunnel: w592 -> [w598]
                  tunnel: [w595] -> w587 mode=indexing if=w594
                  n238 = String To Path(string=w598) -> (path=w597:path[])
                  n239 = Search 1D Array(1D array=w597, element=w595) -> (index of element=w596:i32)  [unwired: 1 in]
                  n240 = Less Than 0?(x=w596) -> (x < 0?=w594:bool)
                }
                n241 = Bundle(cluster=w588, "Path References"=w587) -> (w586:T34)  [unwired: 1 in]
                n242 = call "Versioned Write AQT.vi"("data"=w586, "Aquitaine paths in"=w589) -> ()  [unwired: 9 in, 1 out]
              }
              frame True {
                n243 = for {
                  tunnel: w600 -> [w607] mode=indexing
                  tunnel: w599 -> [w608]
                  # "aqt"
                  n244 = Concatenate Strings("Are you sure you want to delete AQT File: " ("message"), w607, "?" ("string")) -> (w606:string)
                  n245 = Two Button Dialog(message=w606, 1:"No" ("F button name (\"Cancel\")"), 2:"Yes" ("T button name (\"OK\")")) -> (T button?=w601:bool)
                  n246 = case shown="True" w601 {
                    selector: w601 -> [_ w610]
                    tunnel: w608 -> [_ w613]
                    tunnel: w607 -> [_ w612]
                    frame False {
                    }
                    frame True {
                      n247 = invoke on="Tree" class="Tree (strict)" method="Edit Tree Items.Delete"("tag"=w612, "Delete Children"=w610) -> (error out=w609:errorcluster)  [unwired: 3 in, 4 out]
                      n248 = Build Path(base path=w613, name or relative path=w612) -> (appended path=w611:path)
                      n249 = Delete(path (use dialog)=w611, error in=w609) -> ()  [unwired: 3 in, 3 out]
                    }
                  }
                }
              }
            }
          }
        }
        n250 = Unbundle(w574) -> ("Updated Waypoints"=w573:cluster{"x":dbl, "y":dbl, "th":dbl}[])  [unwired: 3 out]
      }
      event "Delete": Value Change {
        n251 = event-data() -> ()  [unwired: 1 in, 6 out]
        n252 = Unbundle(w622) -> ("Updated Waypoints"=w621:cluster{"x":dbl, "y":dbl, "th":dbl}[])  [unwired: 3 out]
        n253 = local read "Open"() -> (w617:i32[])
        n254 = property on="Open" class="MCListbox (strict)"() -> ("ItemNames"=w619:string[][])  [unwired: 2 in, 2 out]
        n255 = Array Size(array=w617) -> (size(s)=w616:i32)
        n256 = Index Array(array=w617) -> (element=w618:i32)  [unwired: 1 in]
        n257 = Array Subset(array=w619, index (row)=w618, length (row)=w616) -> (w615:string[][])  [unwired: 2 in]
        n258 = for {
          tunnel: w615 -> [w635] mode=indexing
          tunnel: w620 -> [w636]
          n259 = Index Array(array=w635, index=0) -> (element=w629:string)
          n260 = String To Path(string=w629) -> (path=w630:path)
          n261 = Build Path(base path=w636, name or relative path=w630) -> (appended path=w633:path)
          n262 = Delete(path (use dialog)=w633, confirm (F)=FALSE) -> (error out=w631:errorcluster)  [unwired: 3 in, 2 out]
          n263 = call <vilib>:"Clear Errors.vi"("error in (no error)"=w631) -> ()  [unwired: 5 in, 2 out]
        }
      }
      event "Open": Shortcut Menu Selection (User) {
        n264 = event-data() -> ("ItemTag"=w646:string)  [unwired: 1 in, 7 out]
        n265 = case shown="\"Delete Path(s)\"" w646 {
          tunnel: w645 -> [_ _ _ w680 _]
          tunnel: w644 -> [w653 w658 w673 w677 w693]
          tunnel: [w652 w657 w672 w676 w692] -> w643
          tunnel: w641 -> [w651 _ w671 w675 _]
          tunnel: [w651 w657 w671 w675 w692] -> w640
          frame "False", Default {
            n266 = Unbundle(w653) -> ("Updated Waypoints"=w652:cluster{"x":dbl, "y":dbl, "th":dbl}[])  [unwired: 3 out]
          }
          frame "Move to Draw Menu" {
            n267 = local read "Open"() -> (w668:i32[])
            n268 = property on="Open" class="MCListbox (strict)"() -> ("ItemNames"=w667:string[][])  [unwired: 2 in, 2 out]
            n269 = Index Array(array=w668) -> (element=w670:i32)  [unwired: 1 in]
            n270 = Array Size(array=w668) -> (size(s)=w669:i32)
            n271 = property on="Draw Menu" class="MCListbox (strict)"() -> ("ItemNames"=w664:string[][])  [unwired: 2 in, 2 out]
            n272 = Unbundle(w658) -> ("Updated Waypoints"=w657:cluster{"x":dbl, "y":dbl, "th":dbl}[])  [unwired: 3 out]
            n273 = Array Subset(array=w667, index (row)=w670, length (row)=w669) -> (w666:string[][])  [unwired: 2 in]
            n274 = Index Array(array=w664, index (col)=0) -> (element=w660:string[])  [unwired: 1 in]
            n275 = Index Array(array=w666, index (col)=0) -> (element=w659:string[])  [unwired: 1 in]
            n276 = Build Array (concatenate)(w660, w659) -> (w656:string[])
            n277 = vi-ref "Compare Strings.vi"() -> (w654:refnum<vi>)
            n278 = call "Sort 1D Array.vim"("less function (built-in <)"=w654, "unsorted array"=w656) -> ("sorted array"=w655:string[])  [unwired: 9 in]
            n279 = Build Array(w655) -> (w662:string[][])
            n280 = Transpose 2D Array(2D array=w662) -> (transposed array=w661:string[][])
            n281 = property on="Draw Menu" class="MCListbox (strict)"("ItemNames"=w661) -> ()  [unwired: 2 in, 2 out]
          }
          frame "New Path" {
            n282 = Unbundle(w673) -> ("Updated Waypoints"=w672:cluster{"x":dbl, "y":dbl, "th":dbl}[])  [unwired: 3 out]
            n283 = local write "Conditions"(T10 {"vInitial (fps)"=0.0, "vFinal (fps)"=0.0} ("Conditions")) -> ()
          }
          frame "Delete Path(s)" {
            n284 = local read "Open"() -> (w678:i32[])
            n285 = Unbundle(w677) -> ("Updated Waypoints"=w676:cluster{"x":dbl, "y":dbl, "th":dbl}[])  [unwired: 3 out]
            n286 = property on="Open" class="MCListbox (strict)"() -> ("ItemNames"=w679:string[][])  [unwired: 2 in, 2 out]
            n287 = Array Size(array=w678) -> (size(s)=w682:i32)
            n288 = Index Array(array=w678) -> (element=w683:i32)  [unwired: 1 in]
            n289 = Array Subset(array=w679, index (row)=w683, length (row)=w682) -> (w681:string[][])  [unwired: 2 in]
            n290 = for {
              tunnel: w681 -> [w690] mode=indexing
              tunnel: w680 -> [w691]
              n291 = Index Array(array=w690, index=0) -> (element=w684:string)
              n292 = String To Path(string=w684) -> (path=w685:path)
              n293 = Build Path(base path=w691, name or relative path=w685) -> (appended path=w688:path)
              n294 = Delete(path (use dialog)=w688, confirm (F)=FALSE) -> (error out=w686:errorcluster)  [unwired: 3 in, 2 out]
              n295 = call <vilib>:"Clear Errors.vi"("error in (no error)"=w686) -> ()  [unwired: 5 in, 2 out]
            }
          }
          frame "Append to Path" {
            n296 = local read "Limits"() -> (w702:T9)
            n297 = Unbundle(w693) -> ("Updated Waypoints"=w695:cluster{"x":dbl, "y":dbl, "th":dbl}[])  [unwired: 3 out]
            n298 = local read "Conditions"() -> (w703:T10)
            n299 = Unbundle(w702) -> ("Velocity (fps)"=w697:dbl, "Accel (fps^2)"=w696:dbl)  [unwired: 2 out]
            n300 = Delete From Array(array=w695) -> (deleted portion=w700:cluster{"x":dbl, "y":dbl, "th":dbl})  [unwired: 2 in, 1 out]
            n301 = Divide(x=w697, y=w696) -> (x/y=w701:dbl)
            n302 = Build Array(w700) -> (w699:cluster{"x":dbl, "y":dbl, "th":dbl}[])
            n303 = Unbundle(w703) -> ("vFinal (fps)"=w698:dbl)  [unwired: 1 out]
            n304 = call "Add First Point.vi"("Accel (f/s^2)"=w696, "Time (s)"=w701, "Initial Points"=w699) -> ("Points"=w692:cluster{"x":dbl, "y":dbl, "th":dbl}[])  [unwired: 8 in]
            n305 = Bundle("vFinal (fps)"=w698, 0.0) -> (w704:cluster{"vFinal (fps)":dbl, dbl})  [unwired: 1 in]
            n306 = local write "Conditions"(w704) -> ()
          }
        }
      }
      event "Open": Double Click {
        # "When a path file is double clicked, load it and update the controls/indicators on the panel"
        n307 = event-data() -> ("Row"=w708:i32)  [unwired: 1 in, 8 out]
        n308 = property on="Open" class="MCListbox (strict)"() -> ("ItemNames"=w733:string[][])  [unwired: 2 in, 2 out]
        n309 = Index Array(array=w733, index (row)=w708, index (col)=0) -> (element=w709:string)
        n310 = Build Path(base path=w714, name or relative path=w709) -> (appended path=w732:path)
        n311 = local write "Filename"(w709) -> ()
        n312 = call "Versioned Load BDX.vi"("path"=w732) -> ("Trajectory Meta"=w713:cluster{"Drive Type":T11, "Path Type":T7}, "Current Limit"=w707:dbl, "Points out"=w715:cluster{"x":dbl, "y":dbl, "th":dbl}[], "Fields"=w720:T23, "Commands out"=w726:T17, "Zero V"=w721:bool, "Reversals"=w725:T31, "Trajectory Data"=w731:T12, "Zero Translational Velocity"=w706:bool)  [unwired: 17 in, 1 out]
        n313 = Unbundle(w725) -> ("Robot Backwards"=w724:bool, "Reverse Path"=w723:bool)
        n314 = Unbundle(w720) -> ("Sample Period (s)"=w719:dbl, w718:T35, "Conditions"=w717:T10, "Overrides"=w716:T8)  [unwired: 1 out]
        n315 = Unbundle(w713) -> ("Drive Type"=w712:T11, "Path Type"=w711:T7)
        n316 = local write "Zero Translational\n Velocity"(w706) -> ()
        n317 = local write "Current Limit"(w707) -> ()
        n318 = local write "Robot Backwards"(w724) -> ()
        n319 = local write "Zero Velocity"(w721) -> ()
        n320 = local write "Reverse Path"(w723) -> ()
        n321 = local write "Limits"(w718) -> ()
        n322 = local write "Drive Type"(w712) -> ()
        n323 = local write "Path Type"(w711) -> ()
        n324 = local write "Sample Period (s)"(w719) -> ()
        n325 = local write "Overrides"(w716) -> ()
        n326 = local write "Conditions"(w717) -> ()
        n327 = Bundle("Trajectory Data"=w731, "Points out"=w715, "Fields"=w720, "Commands out"=w726) -> (w722:T36)  [unwired: 1 in]
      }
      event "Picture": Mouse Down {
        # "Object being clicked"
        # "Process a mouse down on the picture control. Only left clicks do anything.\nDetermine if any object was clicked on and mark it as the drag object for \nmouse move messages."
        n328 = event-data() -> ("Coords"=w749:T37, "Button"=w751:u16, "Mods"=w750:cluster{"Double Click":bool, "Menu Key":bool}, "PlatMods"=w746:T38)  [unwired: 1 in]
        n329 = Unbundle(w739) -> ("Drag Object"=w738:cluster{"Index":i32, "x":dbl, "y":dbl})  [unwired: 2 out]
        n330 = Unbundle(w743) -> ("Updated Waypoints"=w742:cluster{"x":dbl, "y":dbl, "th":dbl}[])  [unwired: 3 out]
        n331 = case shown="1" w751 {
          tunnel: w750 -> [_ _ w763]
          tunnel: w749 -> [_ _ w768]
          tunnel: w742 -> [w755 w759 w769]
          tunnel: [w755 w759 w773] -> w748
          tunnel: w747 -> [_ _ w770]
          tunnel: w738 -> [w753 w756 w764]
          tunnel: [w752 w758 w765] -> w740
          tunnel: w746 -> [_ _ w761]
          frame 0, Default {
            # "middle mouse?"
            n332 = Bundle(cluster=w753, "Index"=-1) -> (w752:cluster{"Index":i32, "x":dbl, "y":dbl})  [unwired: 2 in]
          }
          frame 2 {
            # "Right Button"
            n333 = Bundle(cluster=w756, "Index"=-1) -> (w758:cluster{"Index":i32, "x":dbl, "y":dbl})  [unwired: 2 in]
          }
          frame 1 {
            # "Left Button"
            n334 = Unbundle By Name(w763) -> ("Double Click"=w762:bool)
            n335 = property on="Picture" class="Pict"() -> ("Position"=w772:T18, "Draw Area Size"=w771:T39)  [unwired: 2 in, 2 out]
            n336 = Unbundle By Name(w761) -> ("Shift"=w760:bool)
            n337 = call "Point Test Shapes.vi"("Coords"=w768, "Points"=w769, "Picture in"=w770) -> ("Pt Test Results"=w767:enum16{"Miss", "Rect Hit", "Arrow Hit"}, "Results"=w766:T19)  [unwired: 7 in]
            n338 = case shown="\"Miss\", Default" w767 {
              tunnel: w762 -> [_ _ w820]
              tunnel: w769 -> [w777 w805 w814]
              tunnel: w766 -> [_ w803 w821]
              tunnel: [w780 w806 w815] -> w773
              tunnel: w768 -> [w781 _ _]
              tunnel: w772 -> [w779 _ _]
              tunnel: w771 -> [w778 _ _]
              tunnel: [w775 w798 w817] -> w765
              tunnel: w764 -> [w774 _ w818]
              tunnel: w760 -> [w776 _ w810]
              frame "Miss", Default {
                n339 = case shown="True" w776 {
                  tunnel: w781 -> [w793 _]
                  tunnel: [w790 w797] -> w780
                  tunnel: w779 -> [w789 _]
                  tunnel: w778 -> [w788 _]
                  tunnel: w777 -> [w784 w797]
                  tunnel: [w783 w796] -> w775
                  tunnel: w774 -> [_ w794]
                  frame False {
                    n340 = call "Map to Feet.vi"("Draw Area Size"=w788, "Position"=w789, "Coords (px)"=w793) -> ("Point (ft)"=w787:cluster{dbl, dbl})  [unwired: 8 in]
                    n341 = Array Size(array=w784) -> (size(s)=w782:i32)
                    n342 = Unbundle(w787) -> (w786:dbl, w785:dbl)
                    n343 = Bundle(w786, w785, nan) -> (w791:cluster{dbl, dbl, dbl})  [unwired: 1 in]
                    n344 = Bundle(w782, w786, w785) -> (w783:cluster{i32, dbl, dbl})  [unwired: 1 in]
                    n345 = Build Array (concatenate)(w784, w791) -> (w790:cluster{"x":dbl, "y":dbl, "th":dbl}[])
                  }
                  frame True {
                    n346 = Bundle(cluster=w794, "Index"=-1) -> (w796:cluster{"Index":i32, "x":dbl, "y":dbl})  [unwired: 2 in]
                  }
                }
              }
              frame "Arrow Hit" {
                # "start tracking rotation"
                n347 = Unbundle(w803) -> ("Index"=w802:i32)  [unwired: 1 out]
                n348 = Index Array(array=w805, index=w802) -> (element=w804:cluster{"x":dbl, "y":dbl, "th":dbl})
                n349 = Unbundle(w804) -> ("x"=w801:dbl, "y"=w800:dbl, "th"=w808:dbl)
                n350 = Bundle(cluster=w804, "th"=w808) -> (w807:cluster{"x":dbl, "y":dbl, "th":dbl})  [unwired: 2 in]
                n351 = Bundle(-2, "x"=w801, "y"=w800) -> (w798:cluster{i32, "x":dbl, "y":dbl})  [unwired: 1 in]
                n352 = Replace Array Subset(array=w805, new element=w807) -> (w806:cluster{"x":dbl, "y":dbl, "th":dbl}[])  [unwired: 1 in]
              }
              frame "Rect Hit" {
                n353 = Unbundle(w821) -> ("Index"=w819:i32)  [unwired: 1 out]
                n354 = Array Size(array=w814) -> (size(s)=w813:i32)
                n355 = Greater?(x=w813, y=2) -> (0:w811:bool)
                n356 = And(x=w810, y=w811) -> (x .and. y?=w809:bool)
                n357 = case shown="True" w809 {
                  tunnel: w820 -> [w825 _]
                  tunnel: w819 -> [w824 w828]
                  tunnel: [w823 -1 ("length")] -> w816
                  tunnel: w814 -> [w822 w831]
                  tunnel: [w822 w830] -> w815
                  frame False {
                    n358 = case shown="False" w825 {
                      tunnel: w824 -> [w826 _]
                      tunnel: [w826 -1] -> w823
                      frame False {
                      }
                      frame True {
                        # "TODO Toggle last pt"
                      }
                    }
                  }
                  frame True {
                    n359 = case shown="0" w828 {
                      tunnel: w831 -> [w832 w836]
                      tunnel: w828 -> [_ w835]
                      tunnel: [w832 w833] -> w830
                      frame 0 {
                      }
                      frame Default {
                        n360 = Delete From Array(array=w836, length=1, index=w835) -> (array with subset deleted=w833:cluster{"x":dbl, "y":dbl, "th":dbl}[])  [unwired: 1 out]
                      }
                    }
                  }
                }
                n361 = Bundle(cluster=w818, "Index"=w816) -> (w817:cluster{"Index":i32, "x":dbl, "y":dbl})  [unwired: 2 in]
              }
            }
          }
        }
        n362 = Bundle(cluster=w739, "Drag Object"=w740) -> (w741:T20)  [unwired: 2 in]
      }
      event "Picture": Mouse Move; "Picture": Mouse Up {
        # "If an object was clicked on and is being moved, update position.\nIf nothing is being dragged, you may be hovering over an object and\nwant to draw it differently."
        n363 = event-data() -> ("Type"=w863:T27, "Coords"=w865:T37)  [unwired: 1 in]
        n364 = local read "Robot Size (in)"() -> (w845:cluster{"width":dbl, "height":dbl})
        n365 = Index Array(array=w839) -> (element=w840:cluster{"width":dbl, "height":dbl})  [unwired: 1 in]
        n366 = Unbundle By Name(w845) -> ("width"=w843:dbl)
        n367 = Unbundle By Name(w840) -> ("width"=w838:dbl)  [unwired: 1 out]
        n368 = Divide(x=w843, y=24.0) -> (x/y=w842:dbl)
        n369 = Subtract(x=w838, y=w842) -> (x-y=w841:dbl)
        n370 = Unbundle(w859) -> ("Updated Waypoints"=w858:cluster{"x":dbl, "y":dbl, "th":dbl}[])  [unwired: 3 out]
        n371 = Unbundle(w851) -> ("Drag Object"=w854:cluster{"Index":i32, "x":dbl, "y":dbl})  [unwired: 2 out]
        n372 = Unbundle(w854) -> ("Index"=w862:i32)  [unwired: 2 out]
        n373 = case shown="-1" w862 {
          selector: w862 -> [w876 _]
          tunnel: w865 -> [w885 w893]
          tunnel: [w883 w892] -> w856
          tunnel: [w880 w891] -> w864
          tunnel: w858 -> [w881 w891]
          tunnel: [w877 w890] -> w857
          tunnel: w854 -> [w868 w890]
          tunnel: w863 -> [w878 _]
          tunnel: "Snap to foot" -> [w873 _]
          tunnel: "Snap robot to baseline" -> [w874 _]
          tunnel: "Angle Limiter" -> [w875 _]
          tunnel: w850 -> [w867 w889]
          tunnel: w849 -> [_ w888]
          tunnel: w841 -> [w866 _]
          frame Default {
            # "Mouse up changes indes to break tracking,\notherwise update coords"
            n374 = property on="Picture" class="Pict"() -> ("Position"=w886:T18, "Draw Area Size"=w887:T39)  [unwired: 2 in, 2 out]
            n375 = Bundle("Snap robot to baseline"=w874, "Snap to foot"=w873, "Angle Limiter"=w875) -> (w872:T40)  [unwired: 1 in]
            n376 = Equal?(x=lveventtype."Mouse Up" ("Type"), y=w878) -> (x = y?=w871:bool)
            n377 = call "Map to Feet.vi"("Draw Area Size"=w887, "Position"=w886, "Coords (px)"=w885) -> ("Point (ft)"=w884:cluster{dbl, dbl})  [unwired: 8 in]
            n378 = call "Handle Pos and Rot.vi"("Starting Line Y"=w866, "Mouse Up"=w871, "Picture in"=w867, "Option"=w872, "Coord (ft)"=w884, "Index"=w876, "Points in"=w881) -> ("Points out"=w880:cluster{"x":dbl, "y":dbl, "th":dbl}[])  [unwired: 4 in]
            n379 = Bundle(cluster=w868, "Index"=-1) -> (w869:cluster{"Index":i32, "x":dbl, "y":dbl})  [unwired: 2 in]
            n380 = Bundle(w876, "Pt Test Results"=enum16{"Miss", "Rect Hit", "Arrow Hit"}."Rect Hit") -> (w883:T41)  [unwired: 1 in]
            n381 = Select(t=w869, s=w871, f=w868) -> (s? t:f=w877:cluster{"Index":i32, "x":dbl, "y":dbl})
          }
          frame -1 {
            n382 = call "Point Test Shapes.vi"("Commands"=w888, "Coords"=w893, "Points"=w891, "Picture in"=w889) -> ("Results"=w892:T19)  [unwired: 6 in, 1 out]
          }
        }
        n383 = Bundle(cluster=w851, "Drag Object"=w857, "Hover Object"=w856) -> (w855:T20)  [unwired: 1 in]
      }
      event "Origin Reflection", "Sample Period (s)", "Horizontal Reflection", "Conditions", "Vertical Reflection": Value Change {
        # "Don't updates pts to fit rules"
        # "Changes to any of these controls will update the picture and other indicators to be consistent."
        n384 = event-data() -> ("CtlRef"=w902:refnum<vi>)  [unwired: 1 in]
        n385 = control-ref of="Vertical Reflection"() -> (w910:refnum<vi>)
        n386 = control-ref of="Origin Reflection"() -> (w903:refnum<vi>)
        n387 = control-ref of="Horizontal Reflection"() -> (w923:refnum<vi>)
        n388 = Index Array(array=w906) -> (element=w905:cluster{"width":dbl, "height":dbl})  [unwired: 1 in]
        n389 = Unbundle By Name(w905) -> ("width"=w904:dbl, "height"=w900:dbl)
        n390 = Equal?(x=w902, y=w903) -> (x = y?=w901:bool)
        n391 = Equal?(x=w923, y=w902) -> (x = y?=w908:bool)
        n392 = Equal?(x=w902, y=w910) -> (x = y?=w898:bool)
        n393 = Unbundle(w919) -> ("Updated Waypoints"=w899:cluster{"x":dbl, "y":dbl, "th":dbl}[])  [unwired: 3 out]
        n394 = case shown="True" w901 {
          tunnel: w899 -> [w924 w927]
          tunnel: [w924 w925] -> w896
          frame False {
          }
          frame True {
            n395 = Index Array(array=w927) -> (element=w926:cluster{"x":dbl, "y":dbl, "th":dbl})  [unwired: 1 in]
            n396 = for {
              tunnel: w927 -> [w945] mode=indexing
              tunnel: w926 -> [w944]
              tunnel: [w928] -> w925 mode=indexing
              n397 = Unbundle(w944) -> ("x"=w942:dbl, "y"=w940:dbl)  [unwired: 1 out]
              n398 = Unbundle(w945) -> ("x"=w938:dbl, "y"=w936:dbl, "th"=w935:dbl)
              n399 = Multiply(x=2.0, y=w942) -> (x*y=w939:dbl)
              n400 = Subtract(x=w939, y=w938) -> (x-y=w931:dbl)
              n401 = Add(x=w935, y=180.0) -> (x+y=w933:dbl)
              n402 = Multiply(x=2.0, y=w940) -> (x*y=w937:dbl)
              n403 = Quotient & Remainder(x=w933, y=360.0) -> (x-y*floor(x/y)=w929:dbl)  [unwired: 1 out]
              n404 = Subtract(x=w937, y=w936) -> (x-y=w930:dbl)
              n405 = Bundle(w931, w930, w929) -> (w928:cluster{dbl, dbl, dbl})  [unwired: 1 in]
            }
          }
        }
        n406 = case shown="True" w908 {
          tunnel: w899 -> [w961 w964]
          tunnel: [w961 w963] -> w909
          tunnel: w904 -> [_ w962]
          frame False {
          }
          frame True {
            n407 = for {
              tunnel: w964 -> [w974] mode=indexing
              tunnel: [w971] -> w963 mode=indexing
              tunnel: w962 -> [w968]
              n408 = Unbundle(w974) -> ("x"=w973:dbl, "y"=w972:dbl, "th"=w966:dbl)
              n409 = Negate(x=w973) -> (-x=w970:dbl)
              n410 = Subtract(x=180.0, y=w966) -> (x-y=w965:dbl)
              n411 = Add(x=w968, y=w970) -> (x+y=w969:dbl)
              n412 = Bundle(w969, "y"=w972, w965) -> (w971:cluster{dbl, "y":dbl, dbl})  [unwired: 1 in]
            }
          }
        }
        n413 = case shown="True" w898 {
          tunnel: w899 -> [w946 w949]
          tunnel: [w946 w948] -> w897
          tunnel: w900 -> [_ w947]
          frame False {
          }
          frame True {
            n414 = for {
              tunnel: w949 -> [w959] mode=indexing
              tunnel: [w960] -> w948 mode=indexing
              tunnel: w947 -> [w950]
              n415 = Unbundle By Name(w959) -> ("y"=w958:dbl, "x"=w957:dbl, "th"=w954:dbl)
              n416 = Negate(x=w958) -> (-x=w952:dbl)
              n417 = Negate(x=w954) -> (-x=w953:dbl)
              n418 = Add(x=w950, y=w952) -> (x+y=w951:dbl)
              n419 = Swap Values(12:w951, 14:w957) -> (1:w956:dbl, 3:w955:dbl)  [unwired: 1 in]
              n420 = Bundle(w956, w955, w953) -> (w960:cluster{dbl, dbl, dbl})  [unwired: 1 in]
            }
          }
        }
        n421 = Select(t=w897, s=w898, f=w896) -> (s? t:f=w895:cluster{"x":dbl, "y":dbl, "th":dbl}[])
        n422 = Select(t=w909, s=w908, f=w895) -> (s? t:f=w907:cluster{"x":dbl, "y":dbl, "th":dbl}[])
        n423 = local read "Path Type"() -> (w914:T7)
        n424 = case shown="\"Clothoid\", Default" w914 {
          tunnel: "Unjank" -> [_ w978]
          tunnel: w919 -> [_ w977]
          tunnel: "Turn Acceleration" -> [_ w976]
          tunnel: "Turn Deceleration" -> [_ w975]
          frame "Bezier" {
          }
          frame "Clothoid", Default {
            n425 = case shown="True" w978 {
              tunnel: w977 -> [_ w979]
              tunnel: w976 -> [_ w982]
              tunnel: w975 -> [_ w981]
              frame False {
              }
              frame True {
                n426 = call "Turn Smother.vi"("Ignore Deceleration"=w981, "Ignore Acceleration"=w982, "Internal Path Stuff"=w979) -> ("Overrides"=w980:T8)  [unwired: 1 in]
                n427 = local write "Overrides"(w980) -> ()
              }
            }
          }
        }
      }
      event Key Down?; event type 5.0.x8000000b {
        # "If hovering over an object, nudge using arrow keys"
        n428 = event-data() -> ("VKey"=w1005:T42)  [unwired: 1 in]
        n429 = Index Array(array=w985) -> (element=w986:cluster{"width":dbl, "height":dbl})  [unwired: 1 in]
        n430 = local read "Robot Size (in)"() -> (w988:cluster{"width":dbl, "height":dbl})
        n431 = Unbundle By Name(w986) -> ("width"=w984:dbl)  [unwired: 1 out]
        n432 = Unbundle By Name(w988) -> ("width"=w990:dbl)
        n433 = Divide(x=w990, y=24.0) -> (x/y=w989:dbl)
        n434 = local read "Snap robot to baseline"() -> (w1012:bool)
        n435 = Unbundle(w999) -> ("Updated Waypoints"=w998:cluster{"x":dbl, "y":dbl, "th":dbl}[])  [unwired: 3 out]
        n436 = Subtract(x=w984, y=w989) -> (x-y=w987:dbl)
        n437 = local read "Angle Limiter"() -> (w1010:enum16{"90", "45", "15", "1"})
        n438 = local read "Snap to foot"() -> (w1011:bool)
        n439 = Unbundle(w996) -> ("Hover Object"=w997:T19)  [unwired: 2 out]
        n440 = case shown="\"Up\"" w1005 {
          tunnel: [cluster{dbl, dbl} {0.0, 0.0} ("Coord (ft)") cluster{dbl, dbl} {0.0, 0.1} ("Coord (ft)") cluster{dbl, dbl} {0.0, -0.1} ("Coord (ft)") cluster{dbl, dbl} {-0.1, 0.0} ("Coord (ft)") cluster{dbl, dbl} {0.1, 0.0} ("Coord (ft)")] -> w1007
          tunnel: [_ w1026 w1028 w1030 w1032] -> w1003
          tunnel: TRUE ("Delta") -> [_ w1026 w1028 w1030 w1032]
          frame Default {
          }
          frame "Up" {
          }
          frame "Down" {
          }
          frame "Left" {
          }
          frame "Right" {
          }
        }
        n441 = Unbundle(w997) -> ("Index"=w995:i32, "Pt Test Results"=w1004:enum16{"Miss", "Rect Hit", "Arrow Hit"})
        n442 = Bundle("Snap robot to baseline"=w1012, "Snap to foot"=w1011, "Angle Limiter"=w1010) -> (w1009:T40)  [unwired: 1 in]
        n443 = case shown="\"Rect Hit\", Default" w1004 {
          tunnel: [w1015 w1024] -> w1013
          tunnel: w1000 -> [_ w1023]
          tunnel: w1009 -> [_ w1022]
          tunnel: w998 -> [w1015 w1021]
          tunnel: TRUE ("Delta") -> [_ w1020]
          tunnel: w1007 -> [_ w1019]
          tunnel: w1003 -> [_ w1018]
          tunnel: [_ w1018] -> w1002
          tunnel: w995 -> [_ w1017]
          tunnel: w987 -> [_ w1016]
          frame "Miss" {
          }
          frame "Rect Hit", Default {
            n444 = call "Handle Pos and Rot.vi"("Starting Line Y"=w1016, "Delta"=w1020, "Picture in"=w1023, "Option"=w1022, "Coord (ft)"=w1019, "Index"=w1017, "Points in"=w1021) -> ("Points out"=w1024:cluster{"x":dbl, "y":dbl, "th":dbl}[])  [unwired: 4 in]
          }
        }
        n445 = event-data("Discard?"=w1002) -> ()  [unwired: 1 in, 1 out]
      }
      event User Event {
        # "Fire events to animate the timeline\nuntil we reach the end"
        n446 = event-data() -> ("Data"=w1049:i32)  [unwired: 1 in]
        n447 = Unbundle(w1042) -> ("Updated Waypoints"=w1041:cluster{"x":dbl, "y":dbl, "th":dbl}[])  [unwired: 3 out]
        n448 = Tick Count (ms)() -> (millisecond timer value=w1052:u32)
        n449 = Subtract(x=w1052, y=w1049) -> (x-y=w1051:u32)
        n450 = Multiply(x=w1051, y=0.001) -> (x*y=w1048:dbl)
        n451 = local read "Duration (s)"() -> (w1035:dbl)
        n452 = Quotient & Remainder(x=w1048, y=0.02) -> (floor(x/y)=w1046:dbl)  [unwired: 1 out]
        n453 = Wait (ms)(milliseconds to wait=u32 50) -> ()  [unwired: 1 out]
        n454 = Multiply(x=0.02, y=w1046) -> (x*y=w1045:dbl)
        n455 = Less Or Equal?(x=w1045, y=w1035) -> (x <= y?=w1054:bool)
        n456 = case shown="True" w1054 {
          tunnel: w1036 -> [_ w1059]
          tunnel: w1049 -> [_ w1057]
          tunnel: w1045 -> [_ w1058]
          tunnel: w1035 -> [w1056 _]
          frame False {
            n457 = local write "Time (s)"(w1056) -> ()
          }
          frame True {
            n458 = Generate User Event(user event=w1059, event data cluster=w1057) -> ()  [unwired: 2 in, 2 out]
            n459 = local write "Time (s)"(w1058) -> ()
          }
        }
      }
      event "New Page Selector": Value Change {
        # "If looking at the commands, look at projects for one with a RIO target"
        n460 = event-data() -> ("NewVal"=w1066:T1)  [unwired: 1 in]
        n461 = Unbundle(w1069) -> ("Updated Waypoints"=w1068:cluster{"x":dbl, "y":dbl, "th":dbl}[])  [unwired: 3 out]
        n462 = case shown="\"Command Sequencer\"" w1066 {
          tunnel: [w1072 w1073] -> w1062
          tunnel: w1065 -> [w1072 _]
          frame "Trajectory Settings", Default {
          }
          frame "Command Sequencer" {
            n463 = call "Find RT Projects.vi"() -> ("Paths"=w1074:path[], "Targets"=w1075:refnum<vi>[], "Project Names"=w1076:string[])  [unwired: 9 in]
            n464 = property on="Projects" class="Ring (strict)"("Strings []"=w1076) -> ()  [unwired: 2 in, 2 out]
            n465 = Bundle("Targets"=w1075, "Paths"=w1074) -> (w1073:cluster{"Targets":refnum<vi>[], "Paths":path[]})  [unwired: 1 in]
          }
        }
        n466 = local write "Tab Control"("New Page Selector") -> ()
      }
      event "Refresh": Value Change {
        # "Refresh button was pressed. Reload the command info from the project.\nLater, maybe store this in a file because it takes awhile to recompute."
        n467 = event-data() -> ()  [unwired: 1 in, 1 out]
        n468 = Unbundle(w1086) -> ("Updated Waypoints"=w1085:cluster{"x":dbl, "y":dbl, "th":dbl}[])  [unwired: 3 out]
        n469 = flat-sequence {
          tunnel: [w1089] -> w1079
          tunnel: w1081 -> [w1090]
          tunnel: [w1100] -> w1080
          tunnel: w1079 -> [w1091]
          tunnel: [w1091] -> w1078
          tunnel: [w1106] -> w1083
          tunnel: w1080 -> [w1106]
          tunnel: w1078 -> [w1105]
          frame #0 {
            n470 = call <vilib>:"Set Busy.vi"() -> ("error out"=w1089:errorcluster)  [unwired: 10 in, 1 out]
          }
          frame #1 {
            n471 = Unbundle(w1090) -> ("Targets"=w1096:refnum<vi>[], "Paths"=w1095:path[])
            n472 = Index Array(array=w1096, index="Projects") -> (element=w1104:refnum<vi>)
            n473 = Index Array(array=w1095, index="Projects") -> (element=w1093:path)
            n474 = Strip Path(path=w1093) -> (stripped path=w1092:path)  [unwired: 1 out]
            n475 = call "Find Command Names.vi"("project root path"=w1092, "TargetItem in"=w1104) -> ("Paths"=w1103:path[], "Command Info"=w1102:T43)  [unwired: 8 in]
            n476 = global read "Global Settings.vi" "Icon Scale Factor"() -> (w1097:dbl)
            n477 = call "Format Commands to Tree.vi"("Paths"=w1103, "Command Info"=w1102) -> ("2D Picture"=w1101:picture, "Filtered Command Info Out"=w1099:T2)  [unwired: 8 in]
            n478 = call "Resize Icons.vi"("Scale Factor"=w1097, "Filtered Command Info Out"=w1099) -> ("Filtered Command Info Out"=w1098:T2)  [unwired: 9 in]
            n479 = local write "Command Palette"(w1101) -> ()
            n480 = Bundle("Filtered Command Info Out"=w1098, "2D Picture"=w1101, "stripped path"=w1092) -> (w1100:T44)  [unwired: 1 in]
            n481 = local write "Cache"(w1100) -> ()
          }
          frame #2 {
            n482 = call <vilib>:"Unset Busy.vi"("error in (no error)"=w1105) -> ()  [unwired: 10 in, 1 out]
          }
        }
        n483 = call-poly <vilib>:"Set Cursor.vi"() -> ()  [unwired: 10 in, 2 out]
      }
      event "WayPoints": Value Change {
        # "If the waypoints control is hand-edited, pass the new data along to update the picture and other indicators\nand make it consistent"
        n484 = event-data() -> ("NewVal"=w1108:cluster{"x":dbl, "y":dbl, "th":dbl}[])  [unwired: 1 in]
      }
      event event #0x53 {
        # "This is an alternative to the Inhale button. Notice that it doesn't actually modify anything at the\nmoment."
        n485 = event-data() -> ("VIName"=w1119:string)  [unwired: 1 in]
        n486 = Unbundle(w1129) -> ("Updated Waypoints"=w1128:cluster{"x":dbl, "y":dbl, "th":dbl}[])  [unwired: 3 out]
        n487 = Unbundle(w1127) -> ("Filename"=w1118:string)  [unwired: 2 out]
        n488 = Search and Replace String(input string=w1118, search string=w1119, replace string=w1119) -> (number of replacements=w1124:i32)  [unwired: 5 in, 3 out]
        n489 = call "Find Command with Tag.vi"("Command Tag"=w1118, "Commands"=w1117) -> ("Index"=w1125:i32, "Found Command"=w1126:T45, "Found"=w1122:bool)  [unwired: 7 in]
        n490 = Not Equal To 0?(x=w1124) -> (x != 0?=w1123:bool)
        n491 = And(x=w1122, y=w1123) -> (x .and. y?=w1121:bool)
        n492 = disable-structure shown="Enabled" {
          disable-tunnel: w1126 -> [w1137 _]
          disable-tunnel: w1125 -> [w1136 _]
          disable-tunnel: w1121 -> [w1135 _]
          disable-tunnel: [w1134 _] -> w1120
          disable-tunnel: w1117 -> [w1133 _]
          frame Disabled {
            n493 = case shown="True" w1135 {
              tunnel: w1137 -> [_ w1145]
              tunnel: w1136 -> [_ w1151]
              tunnel: w1133 -> [w1138 w1153]
              tunnel: [w1138 w1152] -> _
              tunnel: [_ FALSE] -> w1134
              frame False {
              }
              frame True {
                n494 = Unbundle(w1145) -> ("Visible"=w1140:bool)  [unwired: 4 out]
                n495 = Unbundle(w1140) -> (w1150)  [unwired: 6 out]
                n496 = Open VI Reference(vi path=w1150) -> (vi reference=w1148:refnum<vi>)  [unwired: 5 in, 1 out]
                n497 = property class="VI"(reference=w1148) -> (reference out=w1143:refnum<vi>, "Panel"=w1149:refnum<vi>)  [unwired: 1 in, 1 out]
                n498 = property class="Pnl"(reference=w1149) -> ("Controls[]"=w1147:refnum<vi>[])  [unwired: 1 in, 2 out]
                n499 = for {
                  tunnel: w1147 -> [w1158] mode=indexing
                  tunnel: [w1155] -> w1146 mode=indexing
                  shift-right: [w1154] -> w1142
                  shift-left: w1143 -> [w1154]
                  n500 = property class="Ctl"(reference=w1158) -> ("Label.Text"=w1157:string, "Value"=w1156:variant)  [unwired: 1 in, 2 out]
                  n501 = Bundle("Label.Text"=w1157, "Value"=w1156) -> (w1155:cluster{"Label.Text":string, "Value":variant})  [unwired: 1 in]
                }
                n502 = Bundle(cluster=w1140, w1146) -> (w1139:T46)  [unwired: 6 in]
                n503 = Bundle(cluster=w1145, "Visible"=w1139) -> (w1144:T45)  [unwired: 4 in]
                n504 = Replace Array Subset(array=w1153, new element=w1144, index=w1151) -> (w1152:T17)
                n505 = Close Reference(reference=w1142) -> ()  [unwired: 1 in, 1 out]
              }
            }
          }
          frame Enabled {
          }
        }
      }
      event "Inhale": Value Change {
        # "Inhale button was pressed. Get the value of the controls/parameters and make them the\nvalues that will be used for the command."
        n506 = event-data() -> ()  [unwired: 1 in, 1 out]
        n507 = Unbundle(w1171) -> ("Updated Waypoints"=w1170:cluster{"x":dbl, "y":dbl, "th":dbl}[])  [unwired: 3 out]
        n508 = Unbundle(w1169) -> ("Filename"=w1168:string)  [unwired: 2 out]
        n509 = Unbundle(w1162) -> ("Filtered Command Info Out"=w1161:T2)  [unwired: 2 out]
        n510 = call "Find Command with Tag.vi"("Command Tag"=w1168, "Commands"=w1160) -> ("Index"=w1165:i32, "Found Command"=w1166:T45, "Found"=w1167:bool)  [unwired: 7 in]
        n511 = case shown="True" w1167 {
          tunnel: w1166 -> [_ w1193]
          tunnel: w1165 -> [_ w1198]
          tunnel: w1160 -> [w1175 w1200]
          tunnel: [w1175 w1199] -> w1164
          tunnel: [_ TRUE] -> w1163
          tunnel: w1161 -> [_ w1179]
          frame False {
          }
          frame True {
            n512 = Unbundle(w1193) -> (w1177:T3)  [unwired: 4 out]
            n513 = Unbundle(w1177) -> ("Name"=w1180:string, "Path"=w1197:path)  [unwired: 5 out]
            n514 = Open VI Reference(vi path=w1197) -> (vi reference=w1181:refnum<vi>, error out=w1185:errorcluster)  [unwired: 5 in]
            n515 = Unbundle(w1185) -> ("code"=w1184:i32)  [unwired: 2 out]
            n516 = Not Equal?(x=w1184, y=0) -> (x != y?=w1182:bool)
            n517 = case shown="True" w1182 {
              tunnel: w1181 -> [w1201 w1205]
              tunnel: w1180 -> [_ w1204]
              tunnel: w1179 -> [_ w1203]
              tunnel: [w1201 w1202] -> w1178
              frame False {
              }
              frame True {
                n518 = call "Replace Command with Cached Command.vi"("Cached Commands"=w1203, "Name"=w1204, "VI in"=w1205) -> ("VI out"=w1202:refnum<vi>)  [unwired: 8 in]
              }
            }
            n519 = property class="VI"(reference=w1178) -> (reference out=w1191:refnum<vi>, "Panel"=w1196:refnum<vi>)  [unwired: 1 in, 1 out]
            n520 = property class="Pnl"(reference=w1196) -> (reference out=w1189:refnum<vi>, "Controls[]"=w1195:refnum<vi>[])  [unwired: 1 in, 1 out]
            n521 = for {
              tunnel: w1195 -> [w1211] mode=indexing
              tunnel: [w1208] -> w1194 mode=indexing
              shift-right: [w1207] -> w1188
              shift-left: w1191 -> [w1207]
              shift-right: [w1206] -> _
              shift-left: w1189 -> [w1206]
              n522 = property class="Ctl"(reference=w1211) -> ("Label.Text"=w1210:string, "Value"=w1209:variant)  [unwired: 1 in, 2 out]
              n523 = Bundle("Label.Text"=w1210, "Value"=w1209) -> (w1208:cluster{"Label.Text":string, "Value":variant})  [unwired: 1 in]
            }
            n524 = Bundle(cluster=w1177, "All Control Values Variant"=w1194) -> (w1176:T3)  [unwired: 6 in]
            n525 = Bundle(cluster=w1193, w1176) -> (w1192:T45)  [unwired: 4 in]
            n526 = Replace Array Subset(array=w1200, new element=w1192, index=w1198) -> (w1199:T17)
            n527 = property class="VI"(reference=w1188, "FP.State"=T28."Closed" ("Front Panel Window:State")) -> (reference out=w1187:refnum<vi>)  [unwired: 1 in, 1 out]
            n528 = Close Reference(reference=w1187) -> ()  [unwired: 1 in, 1 out]
          }
        }
      }
      event "fps": Cursor Move {
        # "The red cursor on the velocity graph was moved to a new location. Update the time slider to be in sync"
        n529 = event-data() -> ("CursIdx"=w1215:i32, "CursLoc"=w1221:cluster{"X":dbl, "Y":dbl})  [unwired: 1 in]
        n530 = Unbundle(w1222) -> ("Updated Waypoints"=w1220:cluster{"x":dbl, "y":dbl, "th":dbl}[])  [unwired: 3 out]
        n531 = Array Size(array=w1218) -> (size(s)=w1217:i32)
        n532 = Greater?(x=w1217, y=w1215) -> (0:w1216:bool)
        n533 = case shown="False" w1216 {
          tunnel: w1221 -> [w1229 w1234]
          tunnel: w1218 -> [w1227 w1232]
          tunnel: [w1227 w1231] -> w1219
          tunnel: w1215 -> [_ w1230]
          frame False {
            n534 = Unbundle(w1229) -> ("X"=w1228:dbl)  [unwired: 1 out]
            n535 = local write "Time (s)"(w1228) -> ()
          }
          frame True {
            n536 = Unbundle(w1234) -> ("X"=w1233:dbl)  [unwired: 1 out]
            n537 = in-place {
              in-place-border: w1233 -> [w1237]
              n538 = in-place-array #2(w1232, w1230) -> (w1236:T45)
              n539 = Bundle(cluster=w1236, "Start Time (s)"=w1237) -> (w1235:T45)  [unwired: 4 in]
              n540 = in-place-array #2(w1235) -> (w1231:T17)  [unwired: 1 out]
            }
          }
        }
      }
      event "Command Sequence": Mouse Down {
        # "second column, tag starting with // indicates an enable click"
        # "Handle a click on a row of the tree within the Command Sequencer tab.\nThis only handles the enable/disable click"
        n541 = event-data() -> ("CtlRef"=w1254:refnum<vi>, "Coords"=w1255:T37, "PlatMods.Shift"=w1242:bool)  [unwired: 1 in]
        n542 = Unbundle(w1257) -> ("Updated Waypoints"=w1256:cluster{"x":dbl, "y":dbl, "th":dbl}[])  [unwired: 3 out]
        n543 = invoke class="Tree (strict)" method="Point To Row Column"(reference=w1254, "Point"=w1255) -> ("Tag"=w1247:string, "Col"=w1238:i32)  [unwired: 6 in, 6 out]
        n544 = String Subset(string=w1247, length (rest)=2 ("length (rest)")) -> (substring=w1253:string)  [unwired: 1 in]
        n545 = Equal?(x=i32[] [4, 3] ("length (rest)"), y=w1238) -> (x = y?=w1240:bool[])
        n546 = Equal?(x="//", y=w1253) -> (x = y?=w1249:bool)
        n547 = Or Array Elements(Boolean array=w1240) -> (logical OR=w1239:bool)
        n548 = And(x=w1249, y=w1239) -> (x .and. y?=w1248:bool)
        n549 = case shown="True" w1248 {
          tunnel: w1246 -> [w1262 w1269]
          tunnel: w1247 -> [_ w1273]
          tunnel: [w1262 w1268] -> w1244
          tunnel: [_ TRUE] -> w1245
          tunnel: w1242 -> [_ w1263]
          tunnel: w1238 -> [_ w1265]
          frame False {
          }
          frame True {
            # "click on enable of a command"
            n550 = Equal?(x=w1265, y=4) -> (x = y?=w1266:bool)
            n551 = call "Find Command with Tag.vi"("Command Tag"=w1273, "Commands"=w1269) -> ("Index"=w1270:i32, "Found Command"=w1271:T45, "Found"=w1272:bool)  [unwired: 7 in]
            n552 = And(x=w1266, y=w1263) -> (x .and. y?=w1267:bool)
            n553 = case shown="True" w1267 {
              tunnel: w1272 -> [w1280 _]
              tunnel: w1271 -> [w1279 _]
              tunnel: w1270 -> [w1278 w1296]
              tunnel: w1269 -> [w1277 w1299]
              tunnel: [w1276 w1298] -> w1268
              tunnel: w1265 -> [w1275 _]
              frame False {
                # "Toggle"
                n554 = case shown="True" w1280 {
                  tunnel: w1279 -> [_ w1283]
                  tunnel: w1278 -> [_ w1286]
                  tunnel: w1277 -> [w1281 w1287]
                  tunnel: [w1281 w1284] -> w1276
                  tunnel: w1275 -> [_ w1282]
                  frame False {
                  }
                  frame True {
                    n555 = case shown="3, Default" w1282 {
                      tunnel: [w1291 w1295] -> w1285
                      tunnel: w1283 -> [w1290 w1294]
                      frame 3, Default {
                        n556 = Unbundle(w1290) -> ("Visible"=w1289:bool)  [unwired: 4 out]
                        n557 = Not(x=w1289) -> (.not. x?=w1288:bool)
                        n558 = Bundle(cluster=w1290, "Visible"=w1288) -> (w1291:T45)  [unwired: 4 in]
                      }
                      frame 4 {
                        n559 = Unbundle(w1294) -> ("Enabled?"=w1293:bool)  [unwired: 4 out]
                        n560 = Not(x=w1293) -> (.not. x?=w1292:bool)
                        n561 = Bundle(cluster=w1294, "Enabled?"=w1292) -> (w1295:T45)  [unwired: 4 in]
                      }
                    }
                    n562 = Replace Array Subset(array=w1287, new element=w1285, index=w1286) -> (w1284:T17)
                  }
                }
              }
              frame True {
                # "Delete"
                n563 = Delete From Array(array=w1299, length=1, index=w1296) -> (array with subset deleted=w1298:T17)  [unwired: 1 out]
              }
            }
          }
        }
      }
      event "Command Sequence": Double Click {
        # "This handles a double-click of a command in the first column. This opens the panel \nand updates the parameters to the values in the command."
        n564 = event-data() -> ("CtlRef"=w1316:refnum<vi>, "Coords"=w1317:T37)  [unwired: 1 in]
        n565 = Unbundle(w1319) -> ("Updated Waypoints"=w1318:cluster{"x":dbl, "y":dbl, "th":dbl}[])  [unwired: 3 out]
        n566 = invoke class="Tree (strict)" method="Point To Row Column"(reference=w1316, "Point"=w1317) -> ("Tag"=w1306:string, "Col"=w1311:i32)  [unwired: 6 in, 6 out]
        n567 = String Subset(string=w1306, length (rest)=2 ("length (rest)")) -> (substring=w1315:string)  [unwired: 1 in]
        n568 = Equal?(x=0 ("length (rest)"), y=w1311) -> (x = y?=w1310:bool)
        n569 = Equal?(x="//", y=w1315) -> (x = y?=w1309:bool)
        n570 = And(x=w1309, y=w1310) -> (x .and. y?=w1308:bool)
        n571 = Unbundle(w1302) -> ("Filtered Command Info Out"=w1301:T2)  [unwired: 2 out]
        n572 = case shown="True" w1308 {
          tunnel: w1307 -> [_ w1328]
          tunnel: w1306 -> [_ w1326]
          tunnel: [_ w1325] -> w1303
          tunnel: w1301 -> [_ w1323]
          frame False {
          }
          frame True {
            n573 = call "Open Command Panel.vi"("Cached Commands"=w1323, "Commands"=w1328, "Tag"=w1326) -> ("Found"=w1327:bool)  [unwired: 8 in]
            n574 = Select(t=w1326, s=w1327, f="") -> (s? t:f=w1325:string)
          }
        }
        n575 = Bundle(cluster=w1304, "Filename"=w1303) -> (w1305:T20)  [unwired: 2 in]
      }
      event "Command Sequence": Edit Cell? {
        w1334 = 2 ("length (rest)")
        # "This allows you to enter time  directly using the tree cell"
        n576 = event-data() -> ("String"=w1343:string, "Tag"=w1342:string, "Col"=w1330:i32)  [unwired: 1 in]
        n577 = Unbundle(w1349) -> ("Updated Waypoints"=w1348:cluster{"x":dbl, "y":dbl, "th":dbl}[])  [unwired: 3 out]
        n578 = Equal?(x=w1334, y=w1330) -> (x = y?=w1333:bool)
        n579 = Equal?(x=w1330, y=1 ("lower limit")) -> (x = y?=w1332:bool)
        n580 = String Subset(string=w1342, length (rest)=w1334) -> (substring=w1347:string)  [unwired: 1 in]
        n581 = Or(x=w1333, y=w1332) -> (x .or. y?=w1331:bool)
        n582 = Equal?(x="//", y=w1347) -> (x = y?=w1345:bool)
        n583 = And(x=w1345, y=w1331) -> (x .and. y?=w1344:bool)
        n584 = case shown="True" w1344 {
          tunnel: [TRUE _] -> w1339
          tunnel: w1343 -> [_ w1364]
          tunnel: w1341 -> [w1354 w1361]
          tunnel: w1342 -> [_ w1360]
          tunnel: [w1354 w1362] -> w1337
          tunnel: w1330 -> [_ w1356]
          frame False {
          }
          frame True {
            n585 = Scan From String(input string=w1364) -> (output 1=w1363:dbl)  [unwired: 4 in, 3 out]
            n586 = call "Find Command with Tag.vi"("Command Tag"=w1360, "Commands"=w1361) -> ("Index"=w1358:i32, "Found Command"=w1357:T45, "Found"=w1359:bool)  [unwired: 7 in]
            n587 = case shown="True" w1359 {
              tunnel: w1361 -> [w1365 w1371]
              tunnel: [w1365 w1372] -> w1362
              tunnel: w1363 -> [_ w1366]
              tunnel: w1358 -> [_ w1369]
              tunnel: w1357 -> [_ w1368]
              tunnel: w1356 -> [_ w1367]
              frame False {
              }
              frame True {
                n588 = case shown="2" w1367 {
                  tunnel: w1366 -> [w1375 w1376]
                  tunnel: [w1374 w1378] -> w1370
                  tunnel: w1368 -> [w1373 w1377]
                  frame 1, Default {
                    n589 = Bundle(cluster=w1373, "Start Time (s)"=w1375) -> (w1374:T45)  [unwired: 4 in]
                  }
                  frame 2 {
                    n590 = Bundle(cluster=w1377, "End Time (s)"=w1376) -> (w1378:T45)  [unwired: 4 in]
                  }
                }
                n591 = Replace Array Subset(array=w1371, new element=w1370, index=w1369) -> (w1372:T17)
              }
            }
          }
        }
        n592 = Sort 1D Array(array=w1337) -> (sorted array=w1336:T17)
        n593 = Not(x=w1339) -> (.not. x?=w1340:bool)
        n594 = event-data("Discard?"=w1339) -> ()  [unwired: 1 in, 1 out]
      }
      event "Command Palette": Mouse Move {
        # "Draw the hilite for the row that the mouse is over"
        n595 = event-data() -> ("Coords"=w1387:T37)  [unwired: 1 in]
        n596 = Unbundle(w1390) -> ("Updated Waypoints"=w1389:cluster{"x":dbl, "y":dbl, "th":dbl}[])  [unwired: 3 out]
        n597 = control-ref of="Command Palette"() -> (w1383:refnum<vi>)
        n598 = call "Picture Coord to Row.vi"("Row Height"=w1382, "Coords"=w1387, "Picture in"=w1383) -> ("Row Index"=w1384:i32, "Clicked in canvas"=w1386:bool)  [unwired: 7 in]
        n599 = Unbundle(w1380) -> ("Filtered Command Info Out"=w1385:T2, "2D Picture"=w1388:picture)  [unwired: 1 out]
        n600 = case shown="True" w1386 {
          tunnel: w1388 -> [_ w1398]
          tunnel: w1385 -> [_ _]
          tunnel: w1382 -> [_ w1396]
          tunnel: w1384 -> [_ w1395]
          frame False {
          }
          frame True {
            n601 = Multiply(x=w1395, y=w1396) -> (x*y=w1401:i32)
            n602 = Add(x=w1401, y=w1396) -> (x+y=w1402:i32)
            n603 = Bundle(0, w1401, 300, w1402) -> (w1403:cluster{i32, i32, i32, i32})  [unwired: 1 in]
            n604 = call <vilib>:"Draw Rectangle.vi"("rect"=w1403, "fill?(F)"=TRUE, "color(black)"=u32 10539263) -> ("new picture"=w1405:picture)  [unwired: 6 in]
            n605 = Concatenate Strings(w1405, w1398) -> (→"Command Palette":picture)
          }
        }
      }
      event "Command Palette": Mouse Down {
        # "When a double click occurs in the command palette,\nadd the command to the command list at time T."
        n606 = event-data() -> ("Coords"=w1418:T37, "Mods"=w1420:cluster{"Double Click":bool, "Menu Key":bool})  [unwired: 1 in, 1 out]
        n607 = control-ref of="Command Palette"() -> (w1419:refnum<vi>)
        n608 = Unbundle(w1422) -> ("Updated Waypoints"=w1421:cluster{"x":dbl, "y":dbl, "th":dbl}[])  [unwired: 3 out]
        n609 = call "Picture Coord to Row.vi"("Row Height"=w1417, "Coords"=w1418, "Picture in"=w1419) -> ("Row Index"=w1413:i32, "Clicked in canvas"=w1416:bool)  [unwired: 7 in]
        n610 = Unbundle(w1420) -> ("Double Click"=w1415:bool)  [unwired: 1 out]
        n611 = Unbundle(w1409) -> ("Filtered Command Info Out"=w1412:T2)  [unwired: 2 out]
        n612 = Compound Arithmetic op=AND(w1416, w1415) -> (w1414:bool)
        n613 = case shown="True" w1414 {
          tunnel: w1413 -> [_ w1434]
          tunnel: w1412 -> [_ w1435]
          tunnel: w1411 -> [w1427 w1432]
          tunnel: [w1427 w1433] -> w1408
          frame False {
          }
          frame True {
            w1428 = TRUE
            n614 = local read "Time (s)"() -> (w1430:dbl)
            n615 = Index Array(array=w1435, index=w1434) -> (element=w1429:T3)
            n616 = Bundle("Time (s)"=w1430, "Time (s)"=w1430, w1429, w1428, w1428) -> (w1431:T47)  [unwired: 1 in]
            n617 = call "Insert Into Sorted Array.vim"("element"=w1431, "sorted array in"=w1432) -> ("sorted array out"=w1433:T17)  [unwired: 9 in]
          }
        }
      }
      event "Add Paths": Value Change {
        n618 = event-data() -> ("NewVal"=w1438:bool)  [unwired: 1 in]
        n619 = case shown="True" w1438 {
          tunnel: w1437 -> [_ w1463]
          frame False {
          }
          frame True {
            n620 = property on="Aquitaine Add Selector" class="Ring (strict)"() -> ("RingText.Text"=w1464:string)  [unwired: 2 in, 2 out]
            n621 = property on="Open" class="MCListbox (strict)"() -> ("ItemNames"=w1459:string[][])  [unwired: 2 in, 2 out]
            n622 = local read "Open"() -> (w1460:i32[])
            n623 = Array Size(array=w1460) -> (size(s)=w1461:i32)
            n624 = Index Array(array=w1460) -> (element=w1462:i32)  [unwired: 1 in]
            n625 = Build Path(base path=w1463, name or relative path=w1464) -> (appended path=w1454:path)
            n626 = Array Subset(array=w1459, index (row)=w1462, length (row)=w1461) -> (w1458:string[][])  [unwired: 2 in]
            n627 = Index Array(array=w1458, index (col)=0) -> (element=w1456:string[])  [unwired: 1 in]
            n628 = call "Versioned Load AQT.vi"("Path"=w1454) -> ("data"=w1450:T34)  [unwired: 10 in]
            n629 = String To Path(string=w1456) -> (path=w1452:path[])
            n630 = Unbundle(w1450) -> ("Path References"=w1453:path[])  [unwired: 1 out]
            n631 = Build Array (concatenate)(w1453, w1452) -> (w1451:path[])
            n632 = call "Remove Duplicates From 1D Array.vim"("array"=w1451) -> ("array with duplicates removed"=w1449:path[])  [unwired: 10 in]
            n633 = Path To String(path=w1449) -> (string=w1448:string[])
            n634 = Sort 1D Array(array=w1448) -> (sorted array=w1447:string[])
            n635 = String To Path(string=w1447) -> (path=w1446:path[])
            n636 = Bundle(cluster=w1450, "Path References"=w1446) -> (w1455:T34)  [unwired: 1 in]
            n637 = call "Versioned Write AQT.vi"("data"=w1455, "Aquitaine paths in"=w1454) -> ()  [unwired: 9 in, 1 out]
          }
        }
        n638 = Unbundle(w1440) -> ("Updated Waypoints"=w1439:cluster{"x":dbl, "y":dbl, "th":dbl}[])  [unwired: 3 out]
      }
      event "Draw Menu": Drop {
        n639 = event-data() -> ("Coords"=w1466:T37, "Available Data Names"=w1468:string[])  [unwired: 1 in]
        n640 = Search 1D Array(1D array=w1468, element="Listbox") -> (index of element=w1471:i32)  [unwired: 1 in]
        n641 = Search 1D Array(1D array=w1468, element="PATH_NAMES") -> (index of element=w1469:i32)  [unwired: 1 in]
        n642 = Not Equal?(x=w1471, y=-1) -> (x != y?=w1467:bool)
        n643 = Not Equal?(x=w1469, y=-1) -> (x != y?=w1473:bool)
        n644 = case shown="True" w1473 {
          tunnel: [w1486 w1529] -> w1474
          tunnel: w1467 -> [w1487 _]
          tunnel: w1466 -> [w1485 w1532]
          frame False {
            n645 = case shown="True" w1487 {
              tunnel: [FALSE TRUE] -> w1486
              tunnel: w1485 -> [_ w1501]
              frame False {
              }
              frame True {
                w1494 = FALSE ("Visible")
                n646 = invoke on="Draw Menu" class="MCListbox (strict)" method="Point To Row Column"("Point"=w1501) -> ("CellPosition"=w1500:T16)  [unwired: 6 in, 6 out]
                n647 = property on="Draw Menu" class="MCListbox (strict)"() -> ("ItemNames"=w1499:string[][])  [unwired: 2 in, 2 out]
                n648 = Get Drag Drop Data(8:i32[] [], 9:"Listbox" ("data name")) -> (3:w1502:i32[])  [unwired: 1 in, 1 out]
                n649 = Array Size(array=w1502) -> (size(s)=w1490:i32)
                n650 = Index Array(array=w1502) -> (element=w1491:i32)  [unwired: 1 in]
                n651 = Unbundle(w1500) -> ("Row"=w1492:i32)  [unwired: 1 out]
                n652 = Add(x=w1490, y=w1491) -> (x+y=w1489:i32)
                n653 = In Range and Coerce(upper limit=w1489, x=w1492, lower limit=w1491) -> (In Range?=w1493:bool)  [unwired: 1 out]
                n654 = case shown="False" w1493 {
                  tunnel: w1491 -> [_ w1525]
                  tunnel: w1499 -> [_ w1520]
                  tunnel: w1492 -> [_ w1516]
                  tunnel: w1490 -> [_ w1510]
                  tunnel: [errorcluster {"status"=FALSE, "code"=0, "source"=""} ("error out") w1508] -> w1495
                  frame True {
                  }
                  frame False {
                    n655 = Index Array(array=w1520, index (col)=0) -> (element=w1518:string[])  [unwired: 1 in]
                    n656 = Array Size(array=w1518) -> (size(s)=w1515:i32)
                    n657 = Delete From Array(array=w1518, length=w1510, index=w1525) -> (deleted portion=w1528:string[], array with subset deleted=w1527:string[])
                    n658 = Less?(x=w1516, y=w1515) -> (x < y?=w1519:bool)
                    n659 = Select(t=w1516, s=w1519, f=w1515) -> (s? t:f=w1517:i32)
                    n660 = Less?(x=w1517, y=w1525) -> (x < y?=w1526:bool)
                    n661 = Subtract(x=w1517, y=w1510) -> (x-y=w1521:i32)
                    n662 = Select(t=w1517, s=w1526, f=w1521) -> (s? t:f=w1512:i32)
                    n663 = Decrement(x=w1510) -> (x-1=w1509:i32)
                    n664 = Insert Into Array(array=w1527, index=w1512, new element=w1528) -> (w1524:string[])
                    n665 = Add(x=w1509, y=w1512) -> (x+y=w1513:i32)
                    n666 = Build Array(w1524) -> (w1523:string[][])
                    n667 = call-poly <vilib>:"Ramp Pattern.vi"("start"=w1512, "end"=w1513, "delta"=1.0) -> ("Ramp Pattern"=w1511:dbl[])  [unwired: 6 in, 2 out]
                    n668 = Transpose 2D Array(2D array=w1523) -> (transposed array=w1522:string[][])
                    n669 = property on="Draw Menu" class="MCListbox (strict)"("Value"=w1511) -> ()  [unwired: 2 in, 2 out]
                    n670 = property on="Draw Menu" class="MCListbox (strict)"("ItemNames"=w1522) -> (error out=w1508:errorcluster)  [unwired: 2 in, 1 out]
                  }
                }
                n671 = global read "Global Settings.vi" "Draw Menu Drag Indicator"() -> (w1498:refnum<vi>[])
                n672 = Index Array(array=w1498) -> (element #1=w1497:refnum<vi>, element #2=w1496:refnum<vi>)  [unwired: 2 in]
                n673 = property on="Property Node" class="Decor"(reference=w1497, error in=w1495, "Visible"=w1494) -> ()  [unwired: 2 out]
                n674 = property on="Property Node" class="Decor"(reference=w1496, error in=w1495, "Visible"=w1494) -> ()  [unwired: 2 out]
              }
            }
          }
          frame True {
            n675 = invoke on="Draw Menu" class="MCListbox (strict)" method="Point To Row Column"("Point"=w1532) -> ("CellPosition"=w1531:T16)  [unwired: 6 in, 6 out]
            n676 = Unbundle(w1531) -> ("Row"=w1530:i32)  [unwired: 1 out]
            n677 = Get Drag Drop Data(8:string[][] [], 9:"PATH_NAMES" ("data name")) -> (3:w1533:string[][])  [unwired: 1 in, 1 out]
            n678 = case shown="0.." w1530 {
              tunnel: w1533 -> [_ w1544]
              tunnel: [FALSE ("Accepted?") TRUE ("Accepted?")] -> w1529
              frame Default {
              }
              frame 0.. {
                n679 = Array Size(array=w1544) -> (size(s)=w1543:i32[])
                n680 = property on="Draw Menu" class="MCListbox (strict)"() -> ("ItemNames"=w1547:string[][])  [unwired: 2 in, 2 out]
                n681 = Multiply Array Elements(1:w1543) -> (0:w1542:i32)
                n682 = Reshape Array(w1544, w1542) -> (w1545:string[])
                n683 = Index Array(array=w1547, index (col)=0) -> (element=w1546:string[])  [unwired: 1 in]
                n684 = Build Array (concatenate)(w1546, w1545) -> (w1541:string[])
                n685 = Build Array(w1541) -> (w1540:string[][])
                n686 = Transpose 2D Array(2D array=w1540) -> (transposed array=w1539:string[][])
                n687 = property on="Draw Menu" class="MCListbox (strict)"("ItemNames"=w1539) -> ()  [unwired: 2 in, 2 out]
              }
            }
          }
        }
        n688 = Unbundle(w1478) -> ("Updated Waypoints"=w1477:cluster{"x":dbl, "y":dbl, "th":dbl}[])  [unwired: 3 out]
        n689 = event-data("Accepted?"=w1474) -> ()  [unwired: 1 in, 1 out]
      }
      event "Draw Menu": event type 3.0.xa000003a {
        n690 = event-data() -> ("Coords"=w1549:T37, "Available Data Names"=w1554:string[])  [unwired: 1 in, 7 out]
        n691 = Search 1D Array(1D array=w1554, element="PATH_NAMES") -> (index of element=w1555:i32)  [unwired: 1 in]
        n692 = Equal?(x=w1555, y=-1) -> (x = y?=w1553:bool)
        n693 = case shown="True" w1553 {
          tunnel: w1549 -> [_ w1590]
          frame False {
          }
          frame True {
            n694 = invoke on="Draw Menu" class="MCListbox (strict)" method="Point To Row Column"("Point"=w1590) -> ("CellPosition"=w1585:T16)  [unwired: 6 in, 6 out]
            n695 = property on="Draw Menu" class="MCListbox (strict)"() -> ("ItemNames"=w1571:string[][])  [unwired: 2 in, 2 out]
            n696 = Index Array(array=w1571, index (col)=0) -> (element=w1569:string[])  [unwired: 1 in]
            n697 = Array Size(array=w1569) -> (size(s)=w1567:i32)
            n698 = Unbundle(w1585) -> ("Row"=w1564:i32)  [unwired: 1 out]
            n699 = Less?(x=w1564, y=w1567) -> (x < y?=w1568:bool)
            n700 = Select(t=w1564, s=w1568, f=w1567) -> (s? t:f=w1566:i32)
            n701 = global read "Global Settings.vi" "Draw Menu Drag Indicator"() -> (w1589:refnum<vi>[])
            n702 = Multiply(x=w1566, y=18) -> (x*y=w1584:i32)
            n703 = Add(x=w1584, y=118) -> (x+y=w1577:i32)
            n704 = Add(x=114, y=w1584) -> (x+y=w1583:i32)
            n705 = Index Array(array=w1589) -> (element #1=w1587:refnum<vi>, element #2=w1588:refnum<vi>)  [unwired: 2 in]
            n706 = Bundle(723, w1583) -> (w1580:cluster{i32, i32})  [unwired: 1 in]
            n707 = Bundle(369, w1577) -> (w1579:cluster{i32, i32})  [unwired: 1 in]
            n708 = property class="Decor"(reference=w1587, "Position"=w1580) -> (reference out=w1576:refnum<vi>, error out=w1575:errorcluster)  [unwired: 1 in]
            n709 = property class="Decor"(reference=w1588, "Position"=w1579) -> (reference out=w1574:refnum<vi>, error out=w1573:errorcluster)  [unwired: 1 in]
            n710 = Greater Or Equal To 0?(x=w1564) -> (x >= 0?=w1565:bool)
            n711 = property class="Decor"(reference=w1576, error in=w1575, "Visible"=w1565) -> ()  [unwired: 2 out]
            n712 = property class="Decor"(reference=w1574, error in=w1573, "Visible"=w1565) -> ()  [unwired: 2 out]
          }
        }
        n713 = event-data("Accepted?"=TRUE) -> ()  [unwired: 1 in, 1 out]
        n714 = Unbundle(w1552) -> ("Updated Waypoints"=w1551:cluster{"x":dbl, "y":dbl, "th":dbl}[])  [unwired: 3 out]
      }
      event "Draw Delete": Value Change {
        n715 = event-data() -> ("NewVal"=w1594:bool)  [unwired: 1 in, 5 out]
        n716 = case shown="True" w1594 {
          frame False {
          }
          frame True {
            n717 = local read "Draw Menu"() -> (w1602:i32[])
            n718 = property on="Draw Menu" class="MCListbox (strict)"() -> ("ItemNames"=w1608:string[][])  [unwired: 2 in, 2 out]
            n719 = Reverse 1D Array(array=w1602) -> (reversed array=w1601:i32[])
            n720 = Index Array(array=w1608, index (col)=0) -> (element=w1604:string[])  [unwired: 1 in]
            n721 = for {
              tunnel: w1601 -> [w1610] mode=indexing
              shift-right: [w1609] -> w1603
              shift-left: w1604 -> [w1611]
              n722 = Delete From Array(array=w1611, index=w1610) -> (array with subset deleted=w1609:string[])  [unwired: 1 in, 1 out]
            }
            n723 = Build Array(w1603) -> (w1606:string[][])
            n724 = Transpose 2D Array(2D array=w1606) -> (transposed array=w1605:string[][])
            n725 = property on="Draw Menu" class="MCListbox (strict)"("ItemNames"=w1605) -> ()  [unwired: 2 in, 2 out]
          }
        }
        n726 = Unbundle(w1593) -> ("Updated Waypoints"=w1592:cluster{"x":dbl, "y":dbl, "th":dbl}[])  [unwired: 3 out]
      }
      event "Draw Menu": Drag Starting? {
        n727 = event-data() -> ()  [unwired: 1 in, 10 out]
        n728 = local read "Draw Menu"() -> (w1617:i32[])
        n729 = To Variant(anything=w1617) -> (Variant=w1616:variant)
        n730 = Bundle("Listbox", "Variant"=w1616) -> (w1614:cluster{string, "Variant":variant})  [unwired: 1 in]
        n731 = Build Array(w1614) -> (w1613:cluster{string, "Variant":variant}[])
        n732 = Unbundle(w1619) -> ("Updated Waypoints"=w1618:cluster{"x":dbl, "y":dbl, "th":dbl}[])  [unwired: 3 out]
        n733 = event-data("Discard?"=TRUE) -> ()  [unwired: 3 in, 1 out]
      }
      event "Draw Menu": Drag Ended {
        n734 = event-data() -> ("Result"=w1629:enum16{"Drop Cancel", "Drop Move", "Drop Copy"})  [unwired: 1 in, 4 out]
        n735 = case shown="\"Drop Cancel\"" w1629 {
          frame "Drop Cancel" {
            w1638 = FALSE ("Visible")
            n736 = global read "Global Settings.vi" "Draw Menu Drag Indicator"() -> (w1641:refnum<vi>[])
            n737 = Index Array(array=w1641) -> (element #1=w1640:refnum<vi>, element #2=w1639:refnum<vi>)  [unwired: 2 in]
            n738 = property on="Property Node" class="Decor"(reference=w1640, "Visible"=w1638) -> ()  [unwired: 1 in, 2 out]
            n739 = property on="Property Node" class="Decor"(reference=w1639, "Visible"=w1638) -> ()  [unwired: 1 in, 2 out]
          }
          frame Default {
          }
        }
        n740 = Unbundle(w1631) -> ("Updated Waypoints"=w1630:cluster{"x":dbl, "y":dbl, "th":dbl}[])  [unwired: 3 out]
      }
      event "Tree", "Open": Drag Starting? {
        n741 = event-data() -> ("CtlRef"=w1651:refnum<vi>)  [unwired: 1 in, 9 out]
        n742 = property class="Ctl"(reference=w1651) -> ("ClassName"=w1646:string)  [unwired: 1 in, 2 out]
        n743 = case shown="\"MulticolumnListbox\", Default" w1646 {
          tunnel: w1652 -> [_ w1670]
          tunnel: [w1660 w1669] -> w1647
          frame "MulticolumnListbox", Default {
            n744 = property on="Open" class="MCListbox (strict)"() -> ("ItemNames"=w1665:string[][])  [unwired: 2 in, 2 out]
            n745 = local read "Open"() -> (w1666:i32[])
            n746 = Array Size(array=w1666) -> (size(s)=w1667:i32)
            n747 = Index Array(array=w1666) -> (element=w1668:i32)  [unwired: 1 in]
            n748 = Array Subset(array=w1665, index (row)=w1668, length (row)=w1667) -> (w1664:string[][])  [unwired: 2 in]
            n749 = Index Array(array=w1664, index (col)=0) -> (element=w1662:string[])  [unwired: 1 in]
            n750 = Build Array(w1662) -> (w1661:string[][])
            n751 = Transpose 2D Array(2D array=w1661) -> (transposed array=w1660:string[][])
          }
          frame "TreeControl" {
            n752 = local read "Tree"() -> (w1671:string[])
            n753 = Index Array(array=w1671) -> (element=w1674:string)  [unwired: 1 in]
            n754 = String To Path(string=w1674) -> (path=w1673:path)
            n755 = call <vilib>:"Get File Extension.vi"("file"=w1673) -> ("lowercase file extension"=w1672:string)  [unwired: 6 in, 4 out]
            n756 = case shown="\"aqt\"" w1672 {
              tunnel: w1671 -> [w1677 w1685]
              tunnel: w1670 -> [_ w1684]
              tunnel: [w1675 w1683] -> w1669
              frame "False", Default {
                n757 = for {
                  tunnel: w1677 -> [w1682] mode=indexing
                  tunnel: [w1678] -> w1676 mode=indexing
                  n758 = Match Pattern(string=w1682, regular expression=".bdx") -> (before substring=w1680:string, match substring=w1679:string)  [unwired: 1 in, 2 out]
                  n759 = Concatenate Strings(w1680, w1679) -> (w1678:string)
                }
                n760 = Build Array(w1676) -> (w1675:string[][])
              }
              frame "aqt" {
                n761 = for {
                  tunnel: w1685 -> [w1690] mode=indexing
                  tunnel: w1684 -> [w1692]
                  tunnel: [w1686] -> w1683 mode=indexing
                  n762 = String To Path(string=w1690) -> (path=w1691:path)
                  n763 = Build Path(base path=w1692, name or relative path=w1691) -> (appended path=w1689:path)
                  n764 = call "Versioned Load AQT.vi"("Path"=w1689) -> ("data"=w1688:T34)  [unwired: 10 in]
                  n765 = Unbundle(w1688) -> ("Path References"=w1687:path[])  [unwired: 1 out]
                  n766 = Path To String(path=w1687) -> (string=w1686:string[])
                }
              }
            }
          }
        }
        n767 = To Variant(anything=w1647) -> (Variant=w1650:variant)
        n768 = Bundle("PATH_NAMES", "Variant"=w1650) -> (w1648:cluster{string, "Variant":variant})  [unwired: 1 in]
        n769 = Build Array(w1648) -> (w1644:cluster{string, "Variant":variant}[])
        n770 = event-data("Discard?"=TRUE) -> ()  [unwired: 3 in, 1 out]
        n771 = Unbundle(w1654) -> ("Updated Waypoints"=w1653:cluster{"x":dbl, "y":dbl, "th":dbl}[])  [unwired: 3 out]
      }
      event "Draw?": Value Change {
        n772 = event-data() -> ("NewVal"=w1694:bool)  [unwired: 1 in, 5 out]
        n773 = Unbundle(w1696) -> ("Updated Waypoints"=w1695:cluster{"x":dbl, "y":dbl, "th":dbl}[])  [unwired: 3 out]
      }
      event "Open Aquitaine Editor": Value Change {
        n774 = event-data() -> ("NewVal"=w1705:bool)  [unwired: 1 in, 5 out]
        n775 = case shown="True" w1705 {
          tunnel: w1704 -> [_ w1720]
          frame False {
          }
          frame True {
            n776 = local read "Tree"() -> (w1719:string[])
            n777 = Index Array(array=w1719) -> (element=w1718:string)  [unwired: 1 in]
            n778 = Build Path(base path=w1720, name or relative path=w1718) -> (appended path=w1716:path)
            n779 = Path To String(path=w1716) -> (string=w1715:string)
            n780 = Search and Replace String(input string=w1715, search string=".aqt") -> (number of replacements=w1713:i32)  [unwired: 6 in, 3 out]
            n781 = Not Equal To 0?(x=w1713) -> (x != 0?=w1717:bool)
            n782 = case shown="True" w1717 {
              tunnel: w1716 -> [_ w1725]
              frame False {
              }
              frame True {
                n783 = call "Find RT Projects.vi"() -> ("Paths"=w1721:path[], "Targets"=w1722:refnum<vi>[])  [unwired: 9 in, 1 out]
                n784 = local read "Projects"() -> (w1724:u16)
                n785 = Bundle("Targets"=w1722, "Paths"=w1721, "Projects"=w1724) -> (w1723:T48)  [unwired: 1 in]
                n786 = disable-structure shown="Enabled" {
                  disable-tunnel: w1725 -> [w1730 w1735]
                  disable-tunnel: w1723 -> [w1726 w1734]
                  frame Enabled {
                    n787 = vi-ref "Aquitaine Editor.vi"() -> (w1732:refnum<vi>)
                    n788 = Open VI Reference(vi path=w1732, options=128) -> (vi reference=w1731:refnum<vi>)  [unwired: 4 in, 1 out]
                    n789 = call-by-ref "Start Asynchronous Call"(reference=w1731, "Project Info"=w1726, "Path"=w1730) -> (reference out=w1729:refnum<vi>, error out=w1728:errorcluster)  [unwired: 11 in]
                    n790 = invoke class="VI Interface Type 0" method="FP.Open"(reference=w1729, error in=w1728) -> (reference out=w1727:refnum<vi>)  [unwired: 3 in, 4 out]
                    n791 = Close Reference(reference=w1727) -> ()  [unwired: 1 in, 1 out]
                  }
                  frame Disabled {
                    n792 = call "Aquitaine Editor.vi"("Project Info"=w1734, "Path"=w1735) -> ()  [unwired: 10 in]
                  }
                }
              }
            }
          }
        }
        n793 = Unbundle(w1707) -> ("Updated Waypoints"=w1706:cluster{"x":dbl, "y":dbl, "th":dbl}[])  [unwired: 3 out]
      }
    }
    n794 = feedback-in #1(w68) -> ()
    n795 = Unbundle(w92) -> (w91:T15)  [unwired: 3 out]
    n796 = Unbundle(w91) -> ("Limits"=w93:T9)  [unwired: 4 out]
    n797 = Unbundle(w93) -> ("Velocity (fps)"=w90:dbl)  [unwired: 3 out]
    n798 = case shown="True" w71 {
      tunnel: w70 -> [_ w238]
      frame False {
      }
      frame True {
        n799 = invoke on="Draw Menu" class="MCListbox (strict)" method="Start Drag"("Data"=w238, "AllowsMove"=enum32{"copy or move", "copy only", "move only"}."move only" ("Drag Mode")) -> ()  [unwired: 3 in, 5 out]
      }
    }
    n800 = case shown="False" w64 {
      tunnel: w122 -> [w161 _]
      tunnel: w121 -> [w160 _]
      tunnel: [w137 w192] -> w120
      tunnel: [w159 w188] -> w114
      tunnel: [w135 w187] -> w111
      tunnel: [w134 w190] -> w103
      tunnel: w96 -> [w158 _]
      tunnel: w95 -> [w157 _]
      tunnel: [w136 w191] -> w94
      tunnel: w90 -> [w156 _]
      tunnel: [w155 w181] -> w88
      tunnel: [w153 w182] -> w86
      tunnel: w81 -> [w150 _]
      tunnel: [w149 w185] -> w80
      tunnel: [w148 w183] -> w79
      tunnel: [w147 w184] -> w78
      tunnel: [w145 w196] -> w75
      tunnel: [w141 w197] -> w74
      tunnel: "Turn Rate (Bezier)" -> [w138 w189]
      tunnel: w68 -> [_ w199]
      tunnel: [w133 w195] -> w67
      tunnel: [w132 w186] -> w66
      tunnel: [w131 w193] -> w65
      tunnel: [_ w177] -> w62
      frame False {
        # "False value updates pts to fit rules"
        # "command tree\nupdate"
        # "New Pts"
        # "Orig Pts"
        n801 = flat-sequence {
          tunnel: ["Time (s)"] -> w162
          tunnel: ["Sample Period (s)"] -> w134
          tunnel: ["Limits"] -> w152
          tunnel: ["Conditions"] -> w144
          tunnel: [w170] -> w136
          tunnel: ["Overrides"] -> w143
          tunnel: w158 -> [w170]
          tunnel: w157 -> [w172]
          tunnel: ["Hide Path"] -> w155
          tunnel: ["Stoopid Overlap %"] -> w154
          tunnel: ["Angular Limits"] -> w142
          tunnel: [w164] -> w139
          frame #0 {
            n802 = control-ref of="Command Sequence"() -> (w173:refnum<vi>)
            n803 = global write "Global Settings.vi" "> 90?"("Allow Angles > 90") -> ()
            n804 = global write "Global Settings.vi" "Turn Angle Limit (deg)"("Turn Angle Limit (deg)") -> ()
            n805 = call "Format Tree.vi"("Update"=w172, "Commands"=w170, "Tree Refnum"=w173) -> ()  [unwired: 9 in]
            n806 = local read "Overrides"() -> (w164:T8)
          }
        }
        n807 = Unbundle(w152) -> ("Accel (fps^2)"=w151:dbl)  [unwired: 3 out]
        n808 = Divide(x=w162, y=w134) -> (x/y=w137:dbl)
        n809 = Bundle("Sample Period (s)"=w134, "Limits"=w152, "Conditions"=w144, "Overrides"=w143, "Angular Limits"=w142) -> (w153:T15)  [unwired: 1 in]
        n810 = call "Enforce Robot Rules.vi"("max V"=w156, "Drive Type"="Drive Type", "Overrides"=w139, "turn accel"=w151, "Disable"=w150, "New Points"=w161, "Original Points"=w160) -> ("Overrides Out"=w145:T8, "Points out"=w141:cluster{"x":dbl, "y":dbl, "th":dbl}[])  [unwired: 3 in]
        n811 = call "GenNewTraj.vi"("Drive Type"="Drive Type", "Turn Rate"=w138, "Stoopid Overlap %"=w154, "Path Type"="Path Type", "Parameters"=w153, "Points in"=w141) -> ("Time & Dist"=w149:cluster{"Time (s)":dbl, "Distance (ft)":dbl}, "Trajectory Data"=w135:T12, "Updated Waypoints"=w159:cluster{"x":dbl, "y":dbl, "th":dbl}[])  [unwired: 2 in, 1 out]
        n812 = Unbundle(w149) -> ("Time (s)"=w147:dbl, "Distance (ft)"=w148:dbl)
        n813 = call "Update Annotations.vi"("Sample Period"=w134, "Commands"=w136, "Trajectory Data"=w135, "Robot Pt Index"=w137) -> ("Redraw"=w131:bool, "Velocity Trace"=w132:dbl[], "Annotation Data"=w133:T49)  [unwired: 5 in]
      }
      frame True {
        n814 = property on="Draw Menu" class="MCListbox (strict)"() -> ("ItemNames"=w200:string[][])  [unwired: 2 in, 2 out]
        n815 = Index Array(array=w200, index (col)=0) -> (element=w198:string[])  [unwired: 1 in]
        n816 = for {
          tunnel: w199 -> [w237]
          tunnel: w198 -> [w236] mode=indexing
          tunnel: [w204] -> w197 mode=concatenating
          tunnel: [w234] -> w196 mode=concatenating
          tunnel: [w232] -> w195 mode=concatenating
          tunnel: [w231] -> w186 mode=concatenating
          tunnel: [w230] -> w194 mode=indexing
          tunnel: [w229] -> w192
          tunnel: [w228] -> w191 mode=concatenating
          tunnel: [w227] -> w190
          tunnel: w189 -> [w223]
          tunnel: [w222] -> w188 mode=concatenating
          tunnel: [w205] -> w187 mode=concatenating
          shift-right: [w219] -> w185
          shift-left: cluster{"Time (s)":dbl, "Distance (ft)":dbl} {"Time (s)"=0.0, "Distance (ft)"=0.0} -> [w220]
          shift-right: [w216] -> _
          shift-left: cluster{"x":dbl, "y":dbl, "th":dbl} {"x"=0.0, "y"=0.0, "th"=0.0} ("Next Point") -> [w217]
          shift-right: [w212] -> w182
          shift-left: T23 {"Sample Period (s)"=0.0, {"Velocity (fps)"=0.0, "Accel (fps^2)"=0.0, "Jerk (fps^3)"=0.0, "StoopidFast (fps)"=0.0}, "Conditions"={"vInitial (fps)"=0.0, "vFinal (fps)"=0.0}, "Overrides"=[], "Angular Limits"={"Velocity (deg/s)"=0.0, "Accel (deg/s^2)"=0.0, "Jerk (deg/s^3)"=0.0}} ("Fields") -> [w211]
          tunnel: [w206] -> w177 mode=indexing
          i -> [w213]
          # "Playback doesn't work in draw menu \nwith paths that have diff sample periods"
          n817 = Build Path(base path=w237, name or relative path=w236) -> (appended path=w235:path)
          n818 = Equal To 0?(x=w213) -> (x = 0?=w214:bool)
          n819 = call "Versioned Load BDX.vi"("path"=w235) -> ("Trajectory Meta"=w226:cluster{"Drive Type":T11, "Path Type":T7}, "Points out"=w204:cluster{"x":dbl, "y":dbl, "th":dbl}[], "Fields"=w212:T23, "Commands out"=w228:T17, "Trajectory Data"=w233:T12)  [unwired: 17 in, 5 out]
          n820 = local read "Time (s)"() -> (w202:dbl)
          n821 = Unbundle By Name(w212) -> ("Conditions.vInitial (fps)"=w209:dbl)
          n822 = Unbundle By Name(w211) -> ("Conditions.vFinal (fps)"=w210:dbl)
          n823 = call "Adjust Points.vi"("Previous Point"=w217, "First Path?"=w214, "Points in"=w204) -> ("Points out"=w215:cluster{"x":dbl, "y":dbl, "th":dbl}[], "Theta Continuity?"=w207:bool, "Next Point"=w216:cluster{"x":dbl, "y":dbl, "th":dbl})  [unwired: 6 in]
          n824 = local read "Stoopid Overlap %"() -> (w218:dbl)
          n825 = Unbundle(w212) -> ("Sample Period (s)"=w227:dbl, "Overrides"=w234:T8)  [unwired: 3 out]
          n826 = Divide(x=w202, y=w227) -> (x/y=w229:dbl)
          n827 = Unbundle(w226) -> ("Drive Type"=w225:T11, "Path Type"=w224:T7)
          n828 = Array Size(array=w204) -> (size(s)=w203:i32)
          n829 = Not Equal?(x=w209, y=w210) -> (x != y?=w208:bool)
          n830 = call "GenNewTraj.vi"("Drive Type"=w225, "Turn Rate"=w223, "Stoopid Overlap %"=w218, "Path Type"=w224, "Parameters"=w212, "Points in"=w215) -> ("Time & Dist"=w221:cluster{"Time (s)":dbl, "Distance (ft)":dbl}, "Trajectory Data"=w205:T12, "Updated Waypoints"=w222:cluster{"x":dbl, "y":dbl, "th":dbl}[])  [unwired: 2 in, 1 out]
          n831 = call "Update Annotations.vi"("Sample Period"=w227, "Commands"=w228, "Trajectory Data"=w233, "Robot Pt Index"=w229) -> ("Redraw"=w230:bool, "Velocity Trace"=w231:dbl[], "Annotation Data"=w232:T49)  [unwired: 5 in]
          n832 = Add(x=w221, y=w220) -> (x+y=w219:cluster{"Time (s)":dbl, "Distance (ft)":dbl})
          n833 = Bundle(w203, "Theta Continuity?"=w207, w208) -> (w206:cluster{i32, "Theta Continuity?":bool, bool})  [unwired: 1 in]
        }
        n834 = local read "Hide Path"() -> (w181:bool)
        n835 = Unbundle(w185) -> ("Time (s)"=w184:dbl, "Distance (ft)"=w183:dbl)
        n836 = Or Array Elements(Boolean array=w194) -> (logical OR=w193:bool)
      }
    }
    "Duration (s)" <- w78
    "Distance (ft)" <- w79
    "Trajectory Data" <- w111
    n837 = Unbundle(w109) -> ("Hover Object"=w108:T19)  [unwired: 2 out]
    n838 = call "Draw Trajectory.vi"("Robot Index"=w120, "Hide Path"=w88, "new picture in"=picture data[5B] ("new picture"), "Trajectory Data"=w111, "Picture in"=w128) -> ("Path Points"=w115:cluster{"x":dbl, "y":dbl}[], "Output Point"=w126:T50, "new picture"=w127:picture)  [unwired: 4 in]
    n839 = call "Draw Shapes.vi"("Picture in"=w128, "Commands"=w94, "Sample Period (s)"=w103, "Points"=w114, "new picture in"=w127, "Results"=w108, "Output Point"=w126, "Continuity"=w62, "Path Points"=w115) -> ("new picture out"=→"Picture":picture)  [unwired: 6 in]
    n840 = local write "WayPoints"(w74) -> ()
    n841 = local write "Overrides"(w75) -> ()
    n842 = case shown="True" w65 {
      tunnel: w67 -> [_ w1737]
      tunnel: w66 -> [_ w1736]
      frame False {
      }
      frame True {
        n843 = property on="fps" class="WFGraph (strict)"("AnntList"=w1737) -> ()  [unwired: 2 in, 2 out]
        "fps" <- w1736
      }
    }
    n844 = property on="Time (s)" class="Slide (strict)"("Scale.Minimum"=0.0 ("Scale.Range:Minimum"), "Scale.Maximum"=w78) -> ()  [unwired: 2 in, 2 out]
    n845 = control-ref of="Save"() -> (w84:refnum<vi>)
    n846 = Bundle(cluster=T22 {"Trajectory Data"=[], "Updated Waypoints"=[], {"Sample Period (s)"=0.0, "Limits"={"Velocity (fps)"=0.0, "Accel (fps^2)"=0.0, "Jerk (fps^3)"=0.0, "StoopidFast (fps)"=0.0}, "Conditions"={"vInitial (fps)"=0.0, "vFinal (fps)"=0.0}, "Overrides"=[], "Angular Limits"={"Velocity (deg/s)"=6.0, "Accel (deg/s^2)"=15.0, "Jerk (deg/s^3)"=150.0}}, "Commands out"=[]} ("output cluster"), "Trajectory Data"=w111, "Updated Waypoints"=w114, w86, "Commands out"=w94) -> (w76:T22)
    n847 = Select(t=0, s=w104, f=2000) -> (s? t:f=w105:i32)
    n848 = call "Saved Checker.vi"("comp B"=w116, "comp A"=w76, "Save button ref"=w84) -> ()  [unwired: 1 in]
  }
  n849 = local write "Time (s)"(0.0 ("Time")) -> ()
